vi "Engine.vi"(8 "Error In":errorcluster, 11 "Message Queues":T1) -> (0 "Error Out":errorcluster)   [LabVIEW 2014]
uses:
  Thread.ctl
  Teszt/Teszt.ctl
  Teszt/Command.ctl
  support/Message Queue/All Message Queues.ctl
  support/Message Queue/Message Cluster.ctl
  Message.ctl
  Thread Flag Control.ctl
  <vilib>/Utility/miscctls.llb/LVRectTypeDef.ctl
  support/Message Queue/Enqueue Message (Single).vi
  global/Global 1.vi
  <vilib>/Utility/error.llb/Error Cluster From Error Code.vi
  <vilib>/ErrorRing/Error Ring.xnode
  support/Message Queue/Message Queue.lvlib
panel:
  out "Threads":T2[](array[typedef])
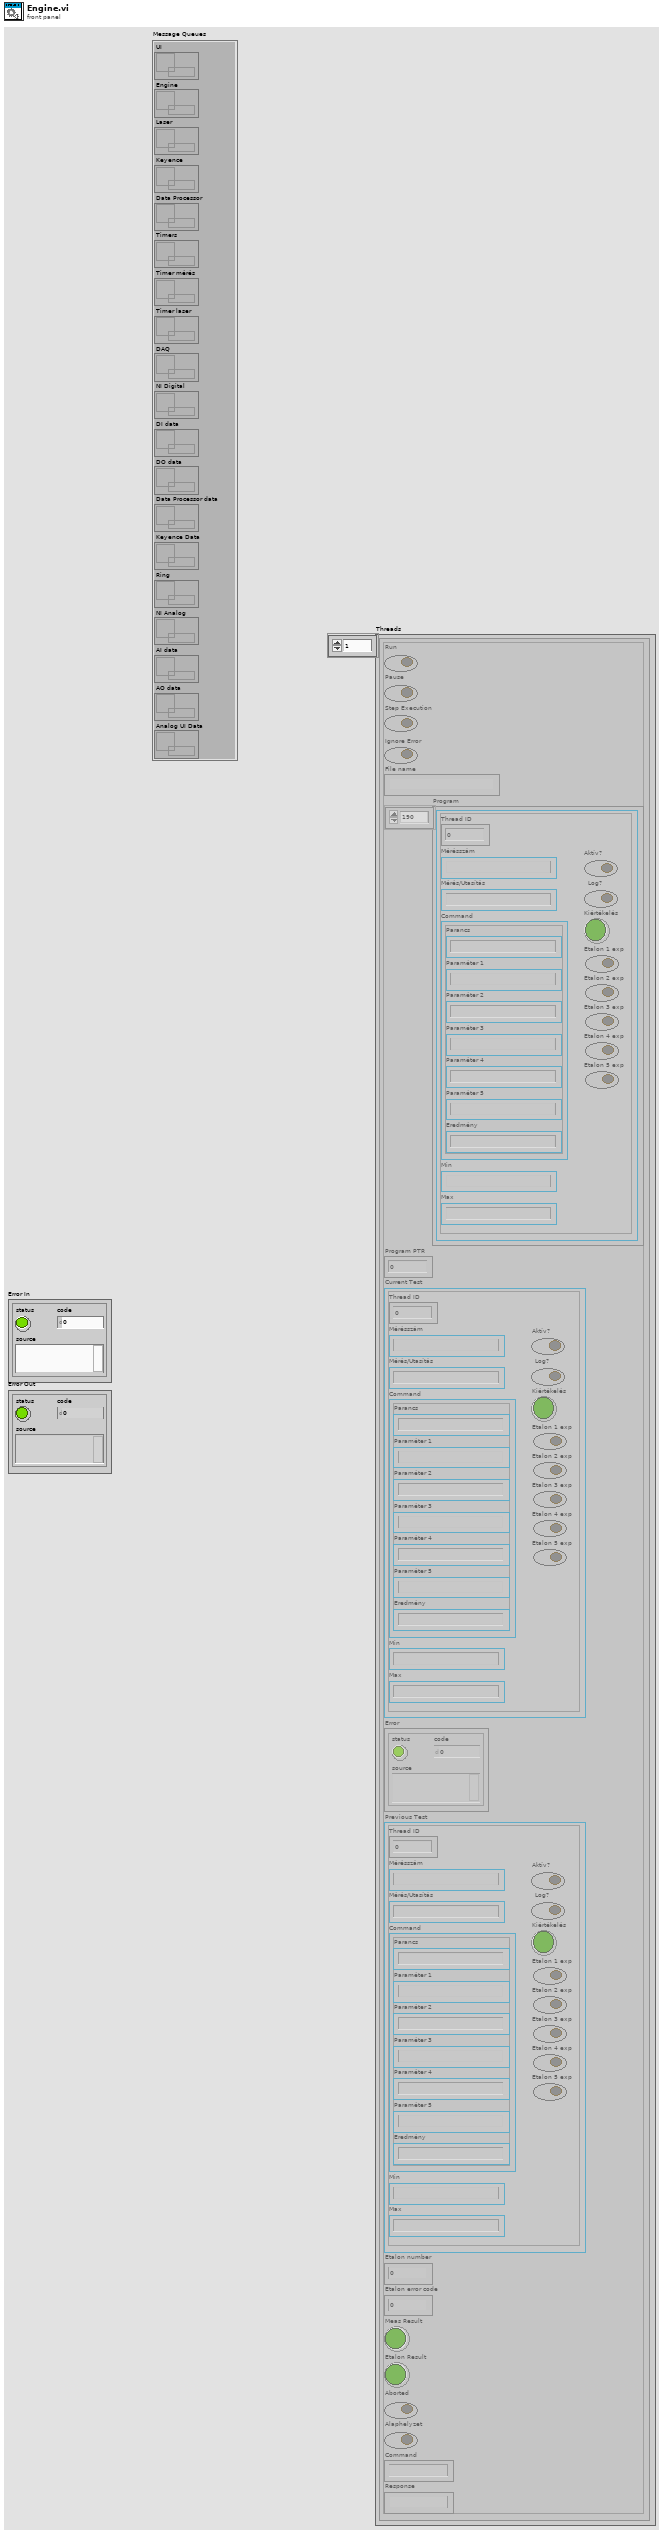
[diagram p1: front panel]
types:
  T1 = typedef "Message Queue.lvlib/All Message Queues.ctl" = cluster{"UI":refnum<queue>, "Engine":refnum<queue>, "Laser":refnum<queue>, "Keyence":refnum<queue>, "Data Processor":refnum<queue>, "Timers":refnum<queue>, "Timer mérés":refnum<queue>, "Timer laser":refnum<queue>, "DAQ":refnum<queue>, "NI Digital":refnum<queue>, "DI data":refnum<queue>, "DO data":refnum<queue>, "Data Processor data":refnum<queue>, "Keyence Data":refnum<queue>, "Ring":refnum<queue>, "NI Analog":refnum<queue>, "AI data":refnum<queue>, "AO data":refnum<queue>, "Analog UI Data":refnum<queue>}
  T2 = typedef "Thread.ctl" = cluster{"Run":bool, "Pause":bool, "Step Execution":bool, "Ignore Error":bool, "File name":string, "Program":T3[], "Program PTR":u32, "Current Test":T3, "Error":errorcluster, "Previous Test":T3, "Etalon number":u32, "Etalon error code":u32, "Meas Result":bool, "Etalon Result":bool, "Aborted":bool, "Alaphelyzet":bool, "Command":string, "Response":string}
  T3 = typedef "Teszt.ctl" = cluster{"Thread ID":dbl, "Mérésszám":string, "Mérés/Utasítás":string, "Command":T4, "Min":string, "Max":string, "Aktív?":bool, "Log?":bool, "Kiértékelés":bool, "Etalon 1 exp":bool, "Etalon 2 exp":bool, "Etalon 3 exp":bool, "Etalon 4 exp":bool, "Etalon 5 exp":bool}
  T4 = typedef "Command.ctl" = cluster{"Parancs":string, "Paraméter 1":string, "Paraméter 2":string, "Paraméter 3":string, "Paraméter 4":string, "Paraméter 5":string, "Eredmény":string}
  T5 = typedef "Termék cluster.ctl" = cluster{"Termék név":string, "Teszt szekvencia":path, "Etalonok száma":i8}
  T6 = typedef "LVRectTypeDef.ctl" = cluster{"Left":i16, "Top":i16, "Right":i16, "Bottom":i16}
  T7 = typedef "Message.ctl" = cluster{"Thread ID":u16, "Callback":string, "Data":variant, "Error":errorcluster}
  T8 = typedef "Thread Flag Control.ctl" = cluster{"Thread ID":u16, "Thread Flag":bool}
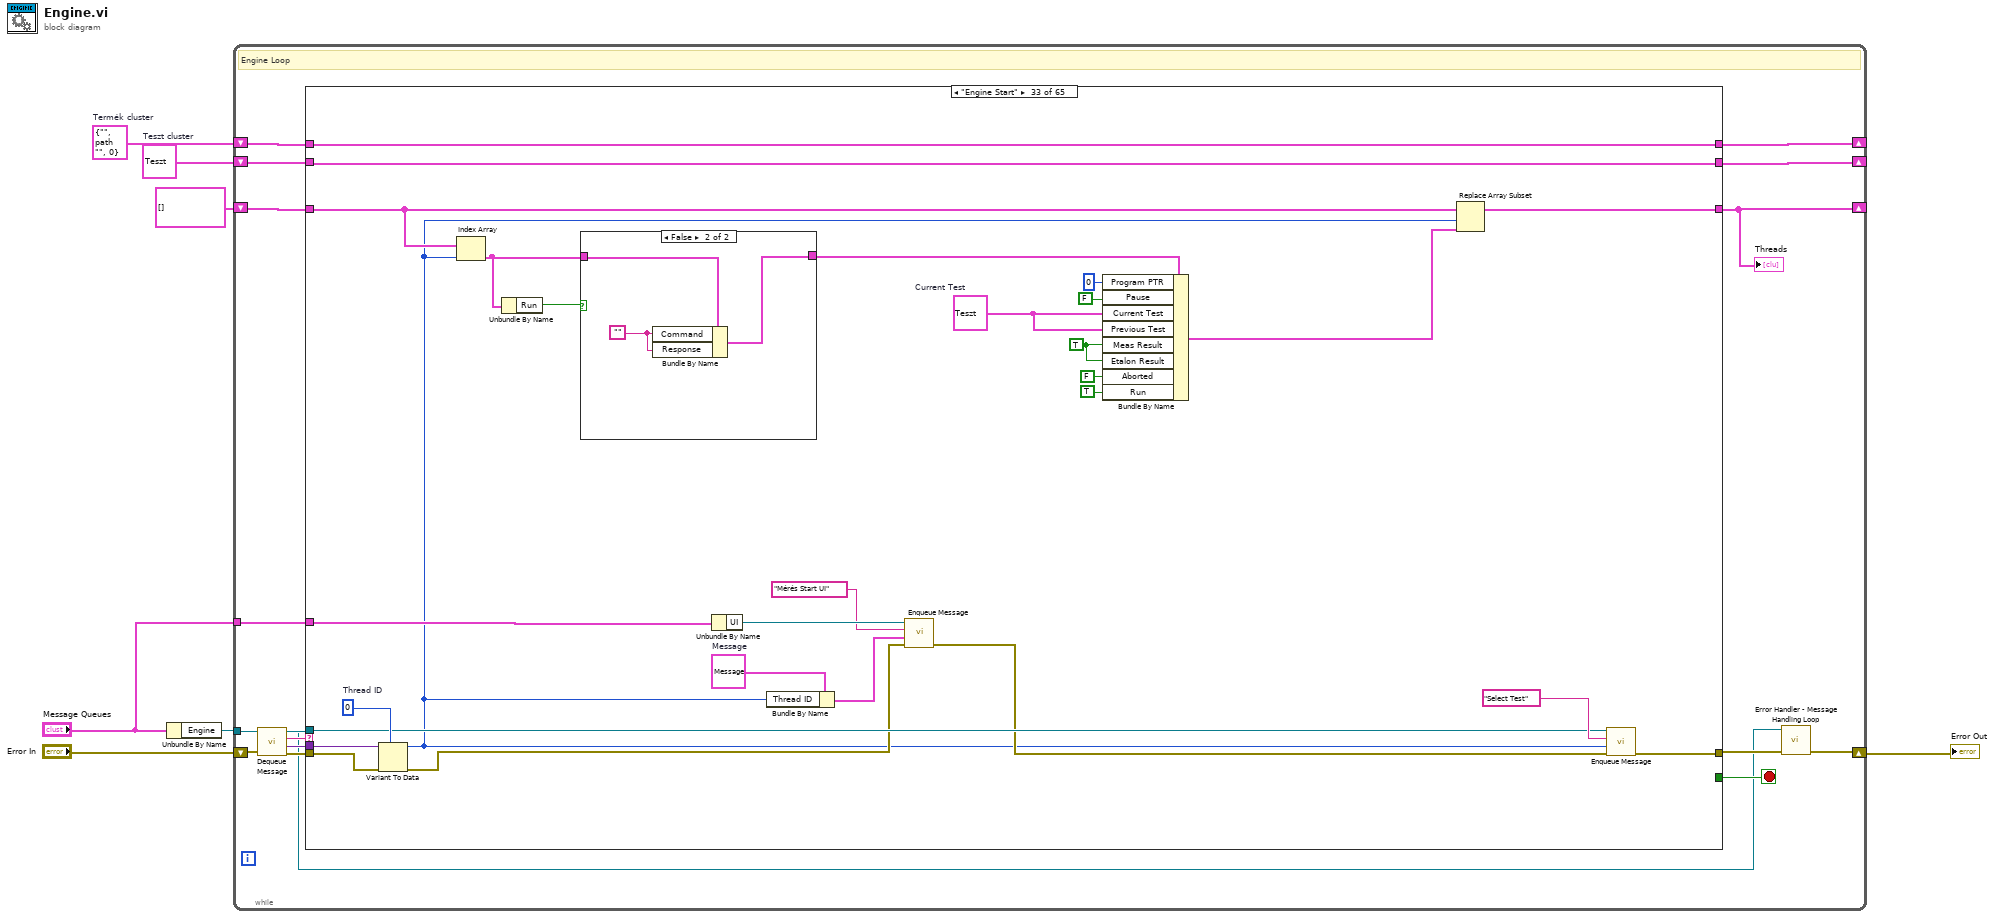
[diagram p0: block diagram]
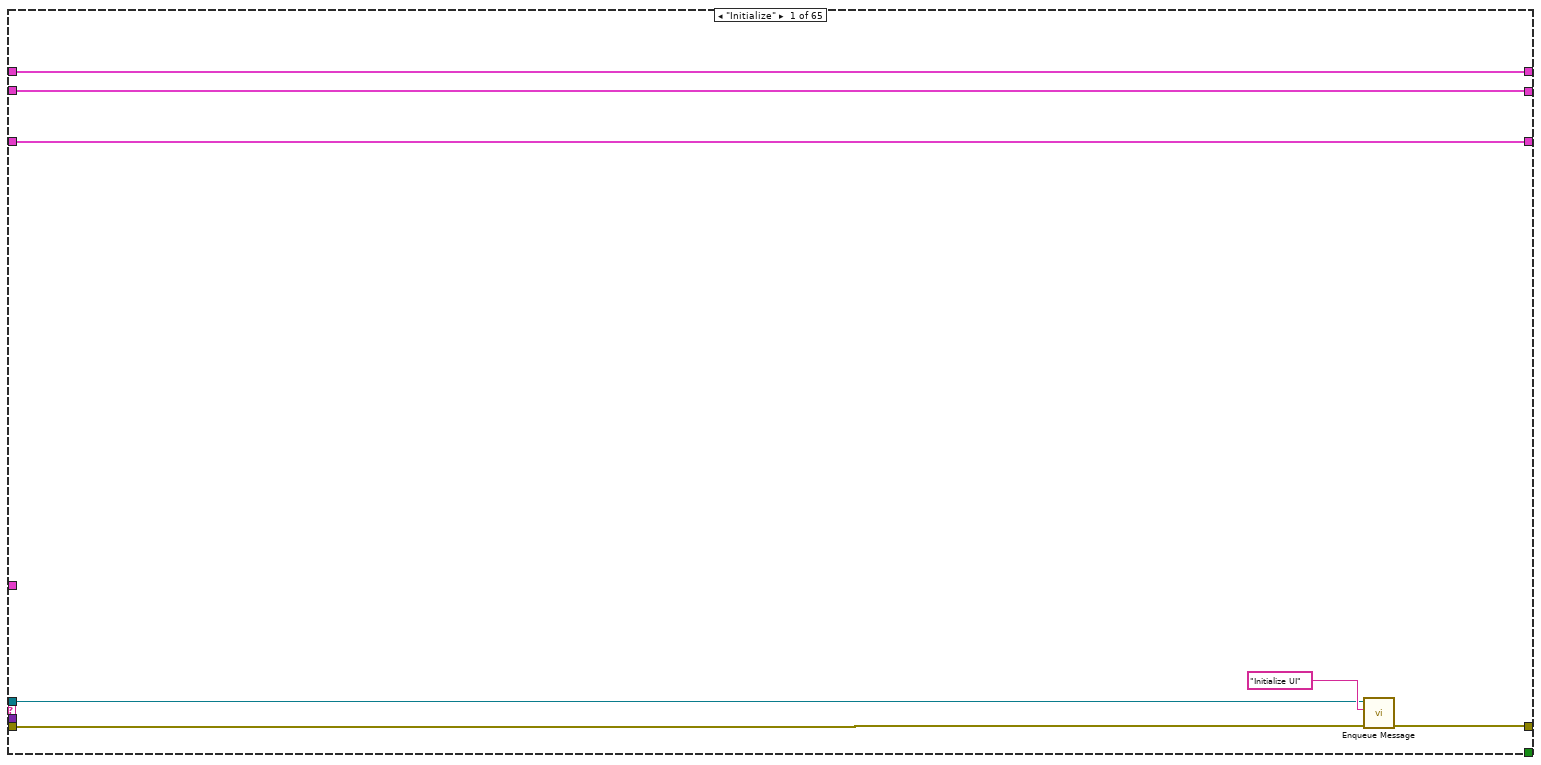
[diagram p2: hidden frame]
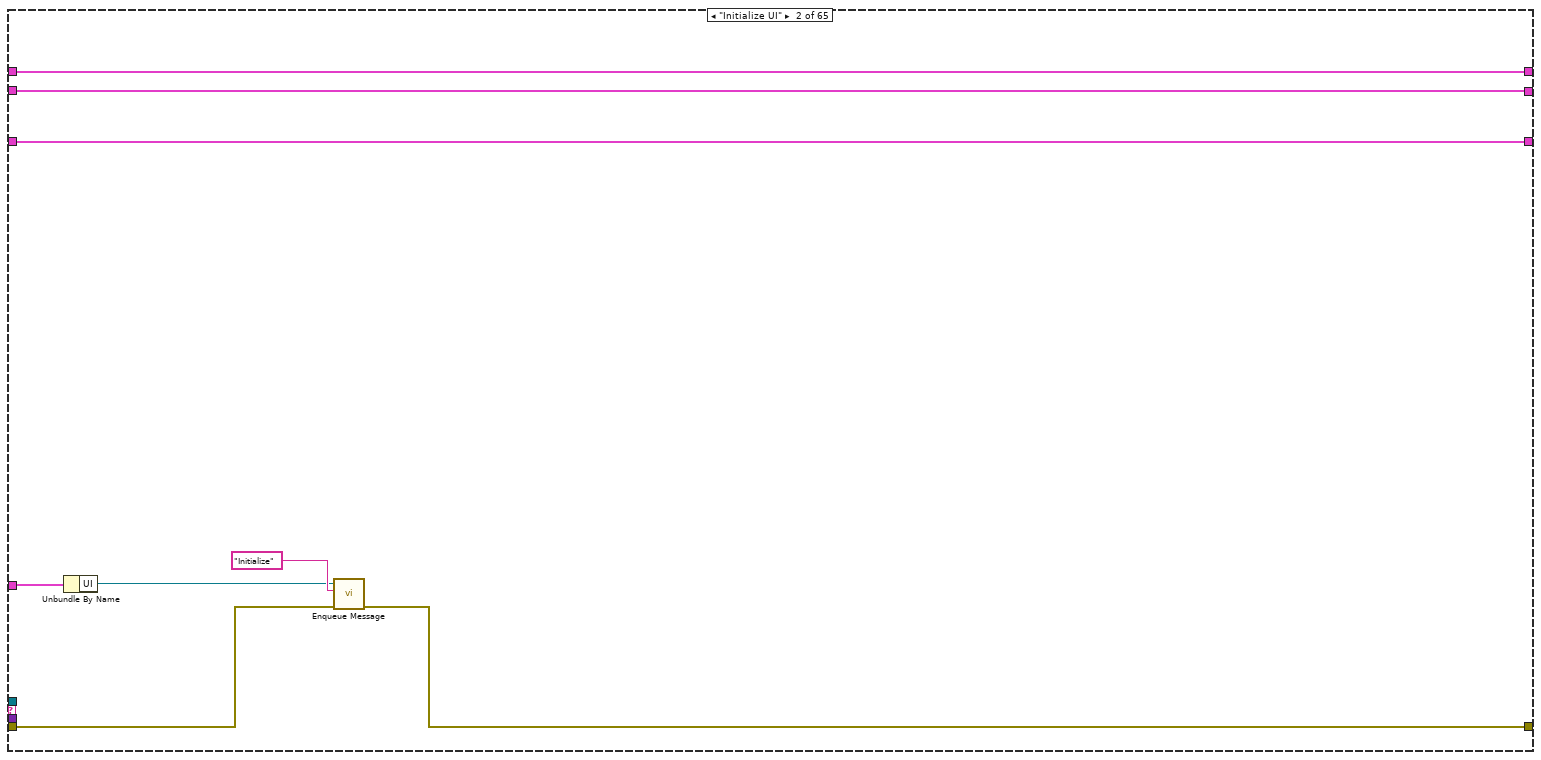
[diagram p3: hidden frame]
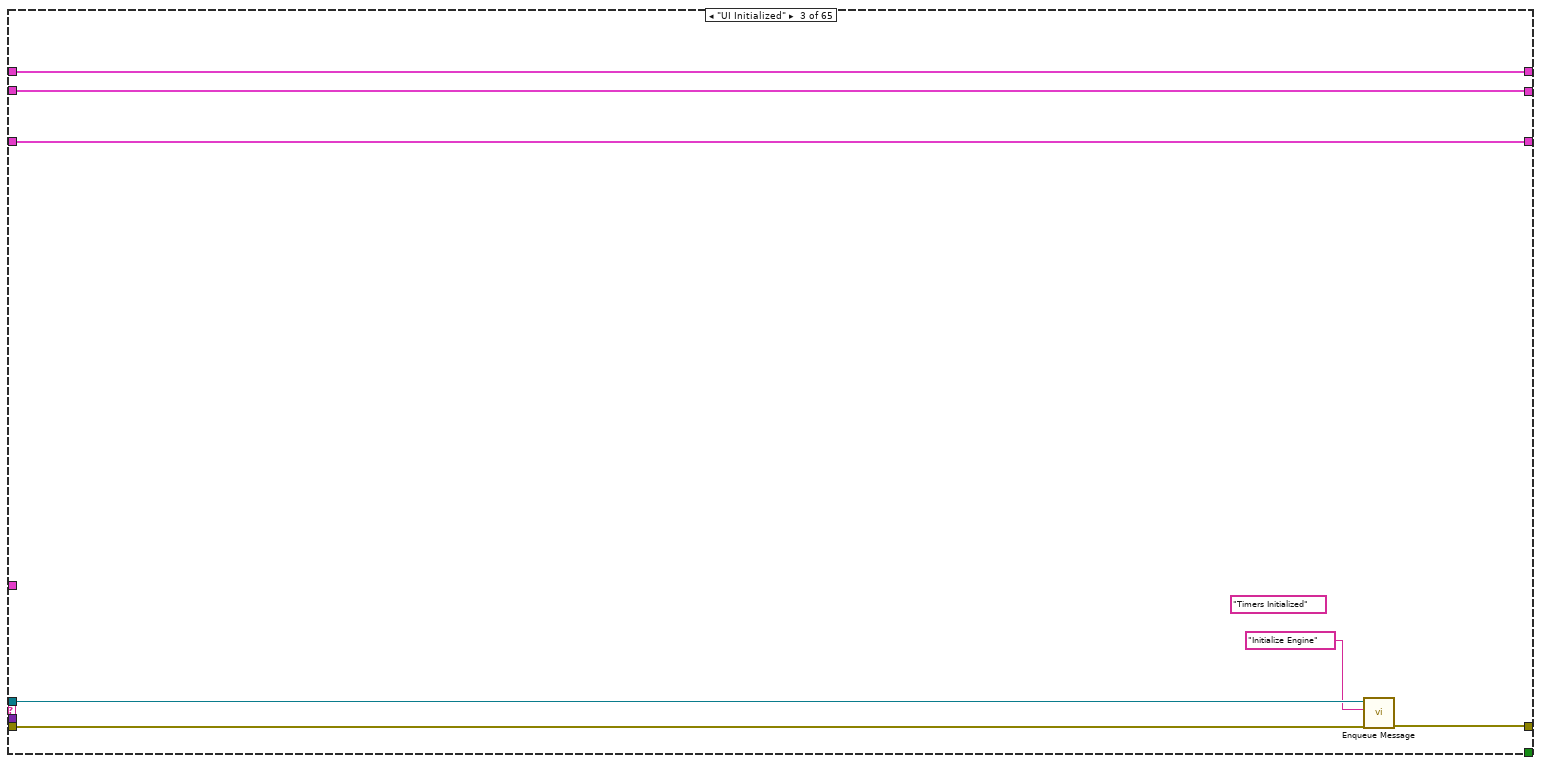
[diagram p4: hidden frame]
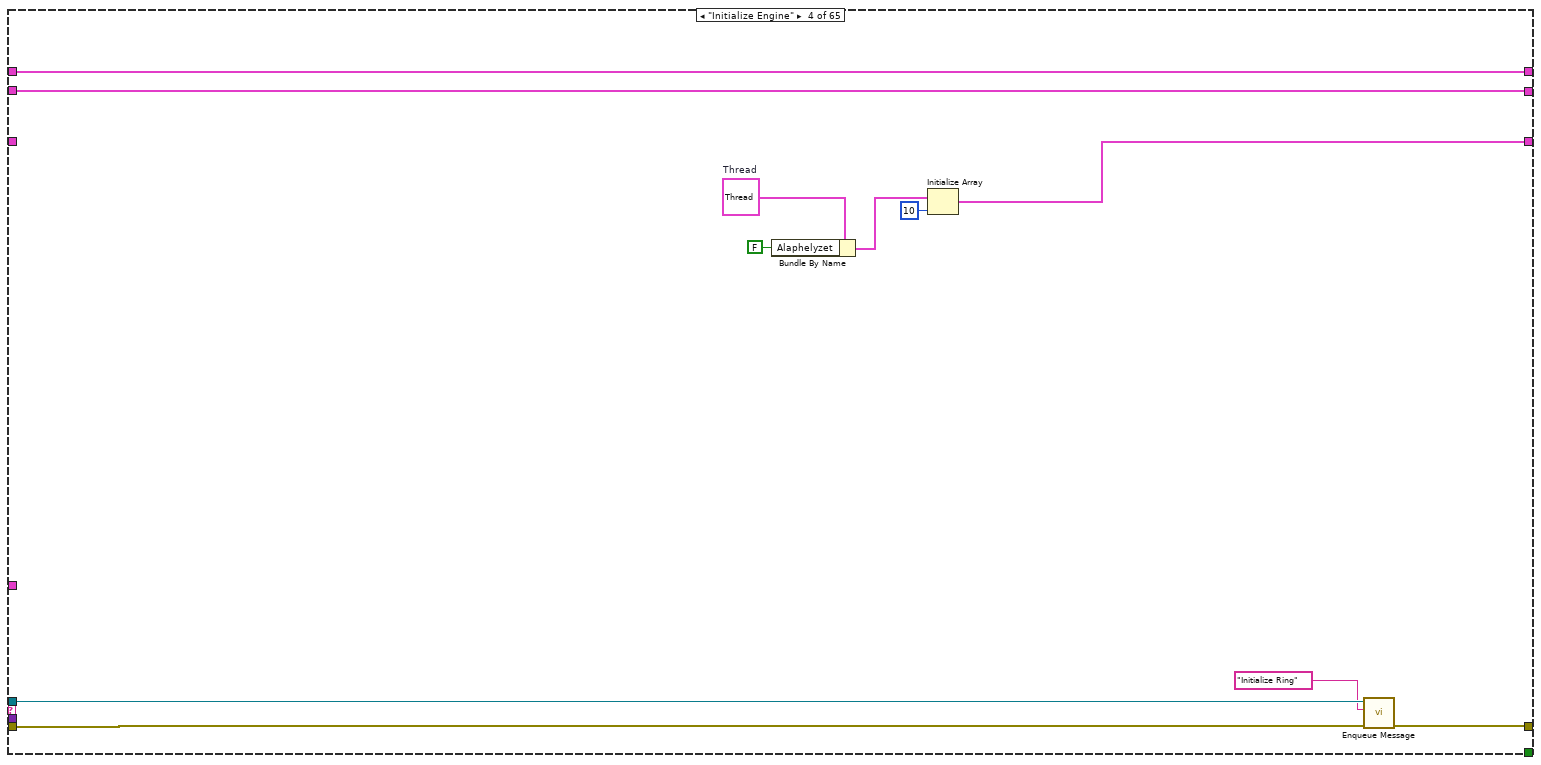
[diagram p5: hidden frame]
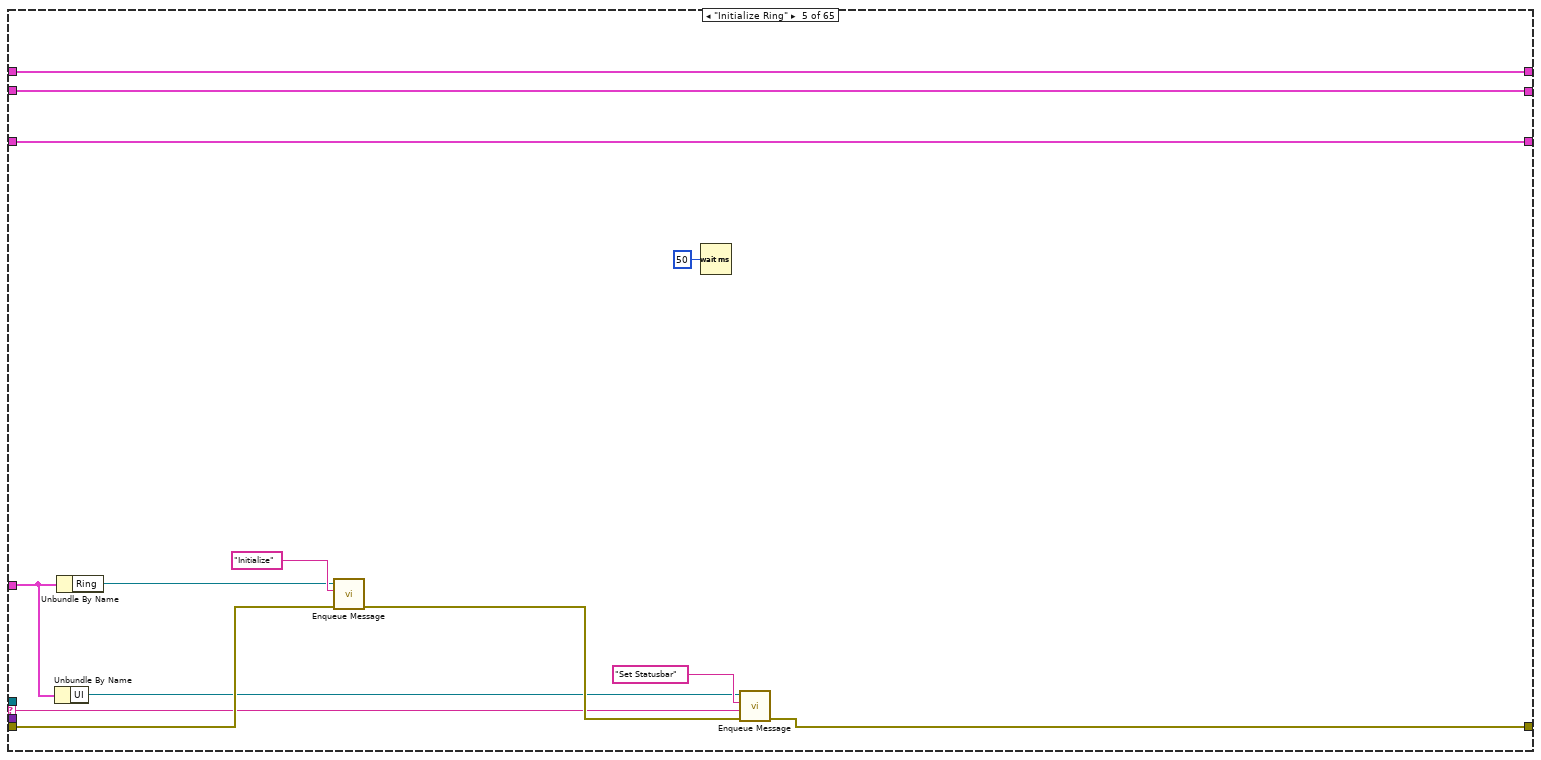
[diagram p6: hidden frame]
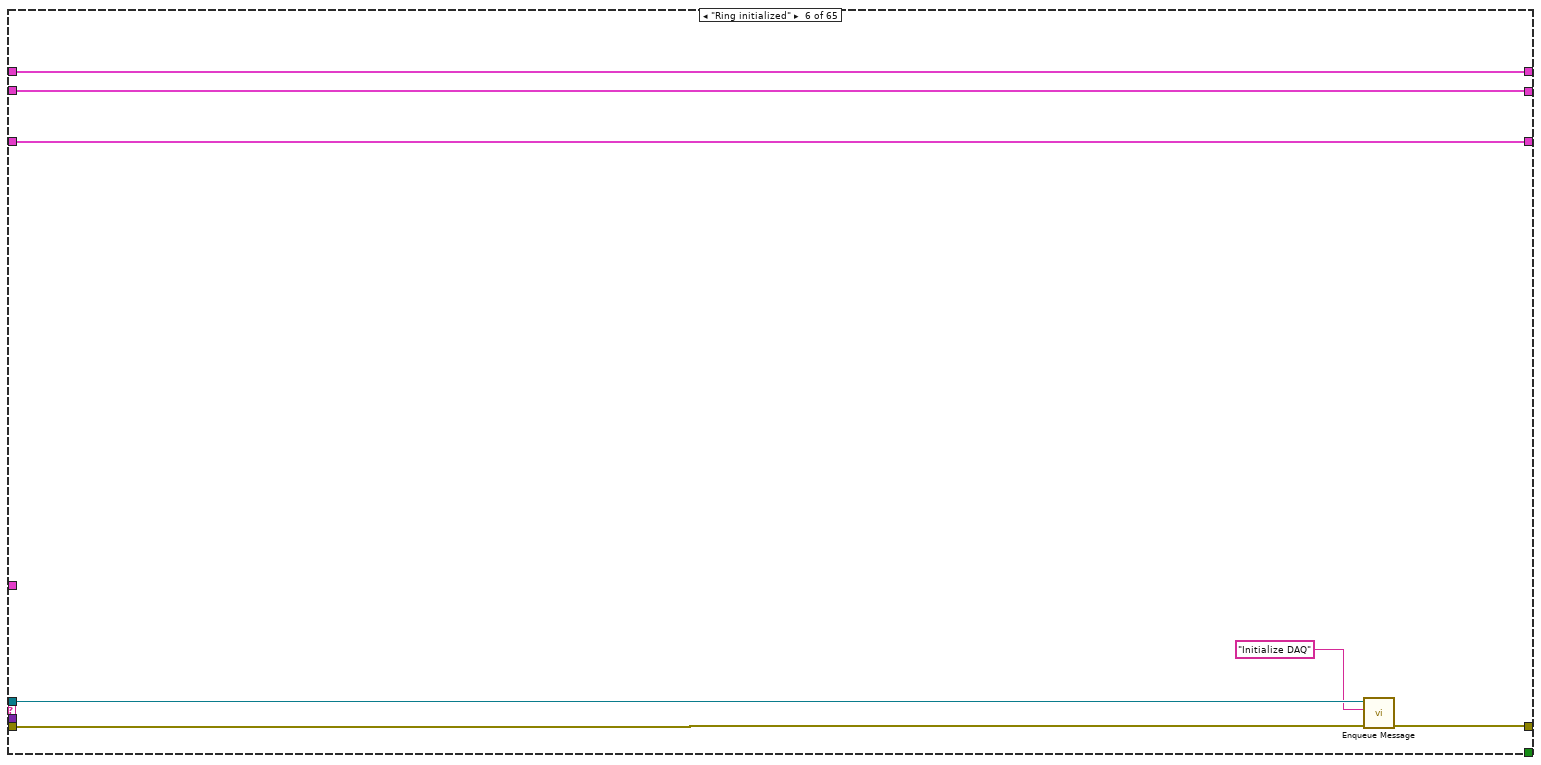
[diagram p7: hidden frame]
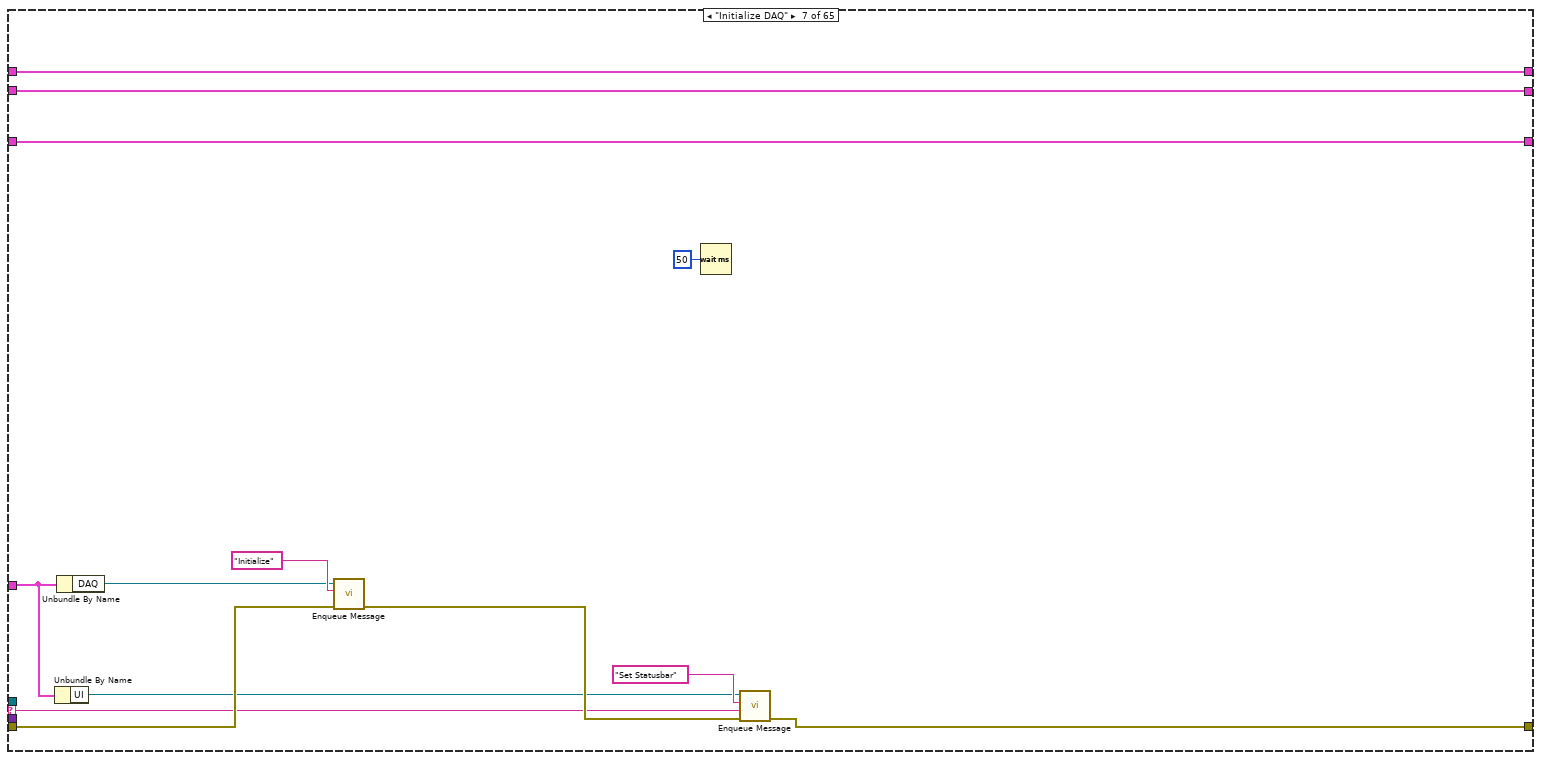
[diagram p8: hidden frame]
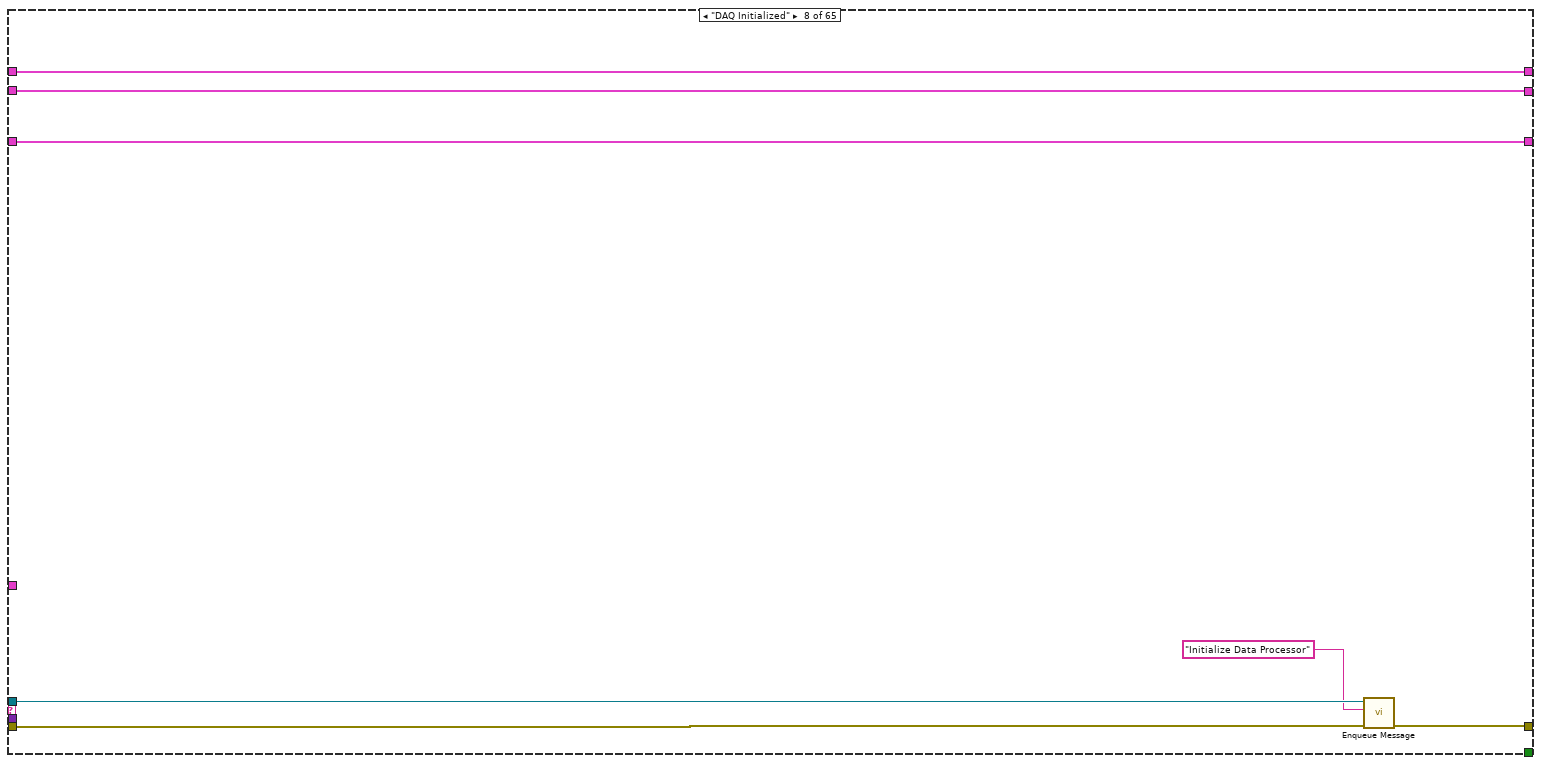
[diagram p9: hidden frame]
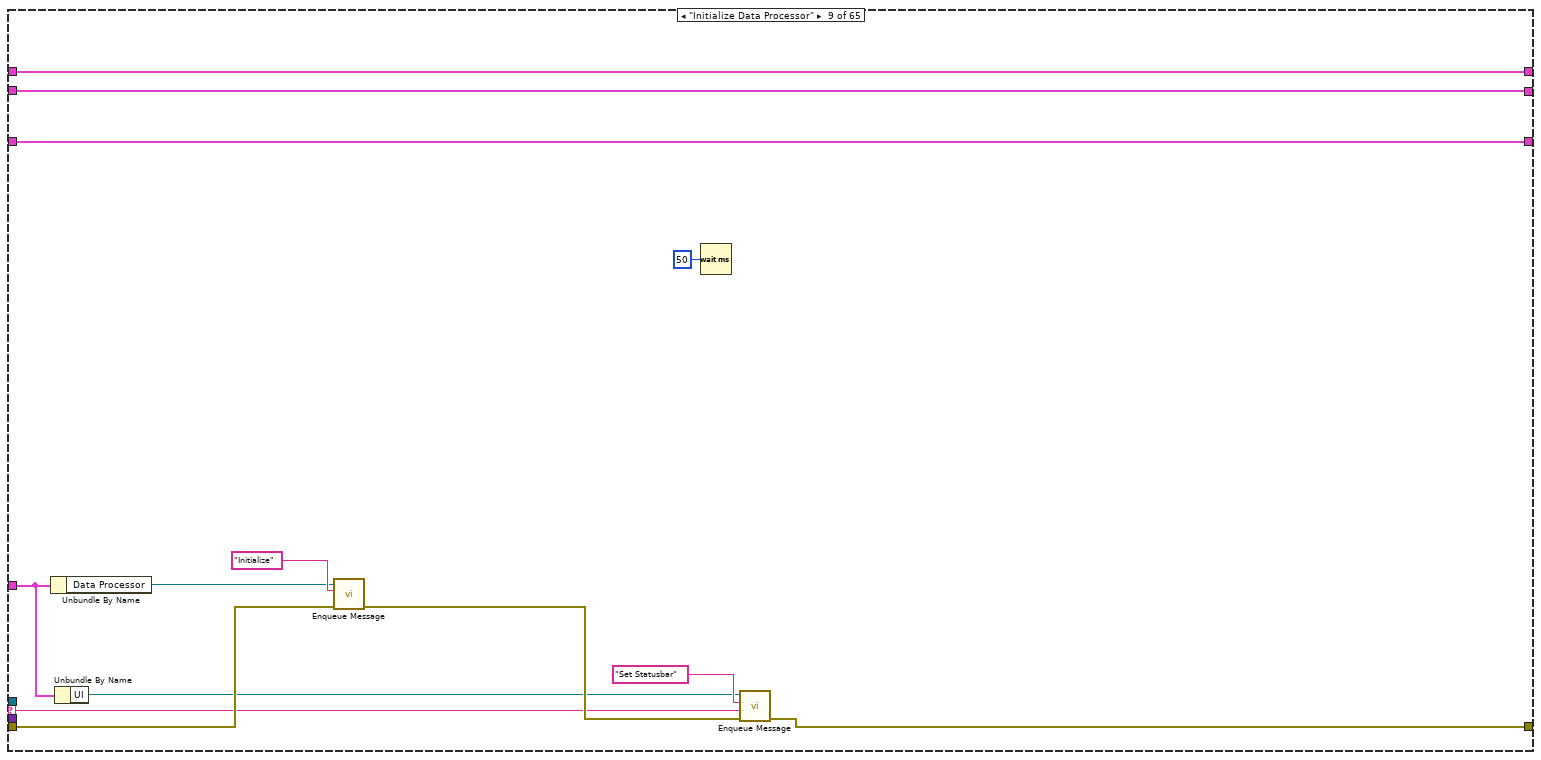
[diagram p10: hidden frame]
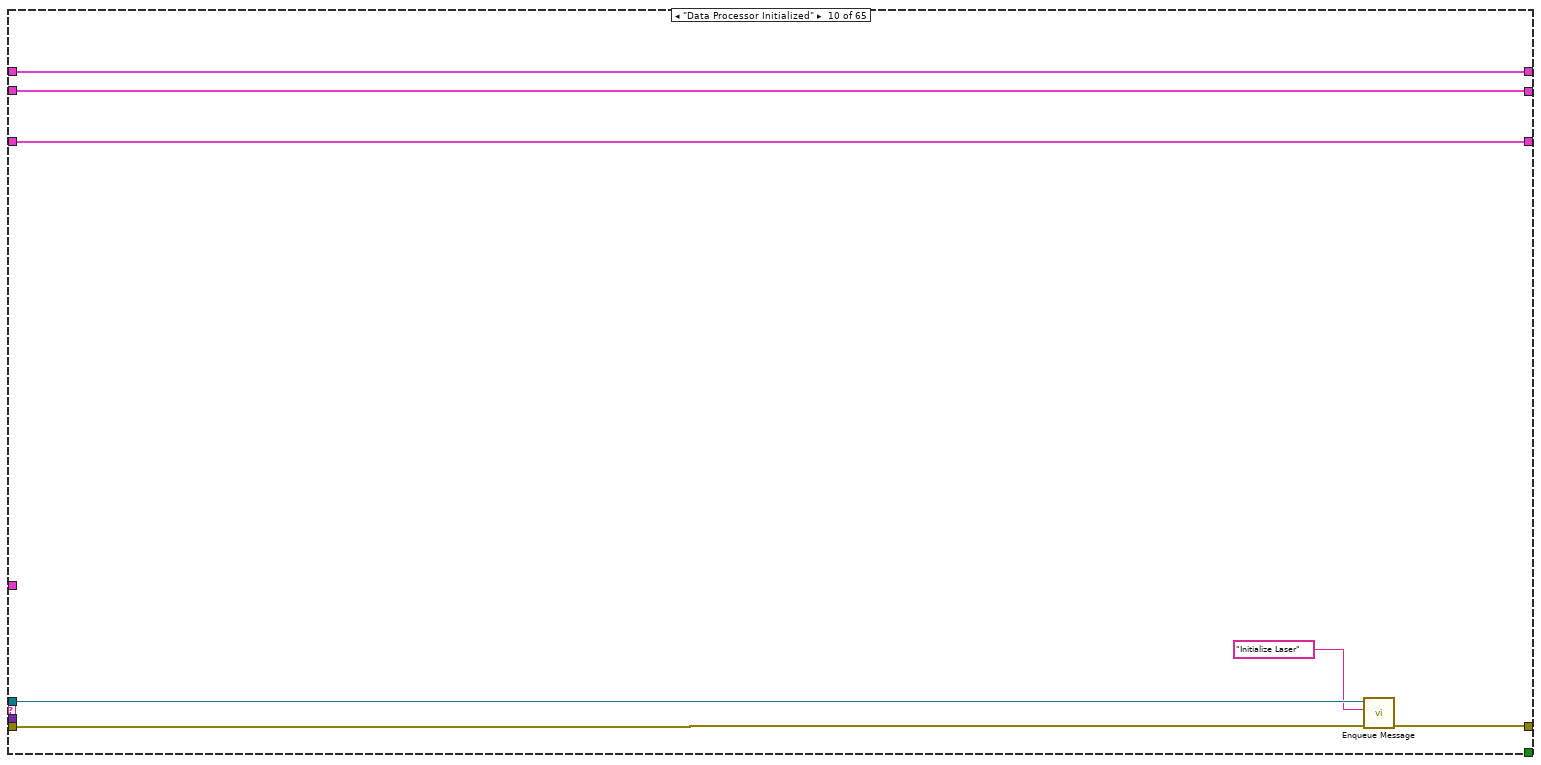
[diagram p11: hidden frame]
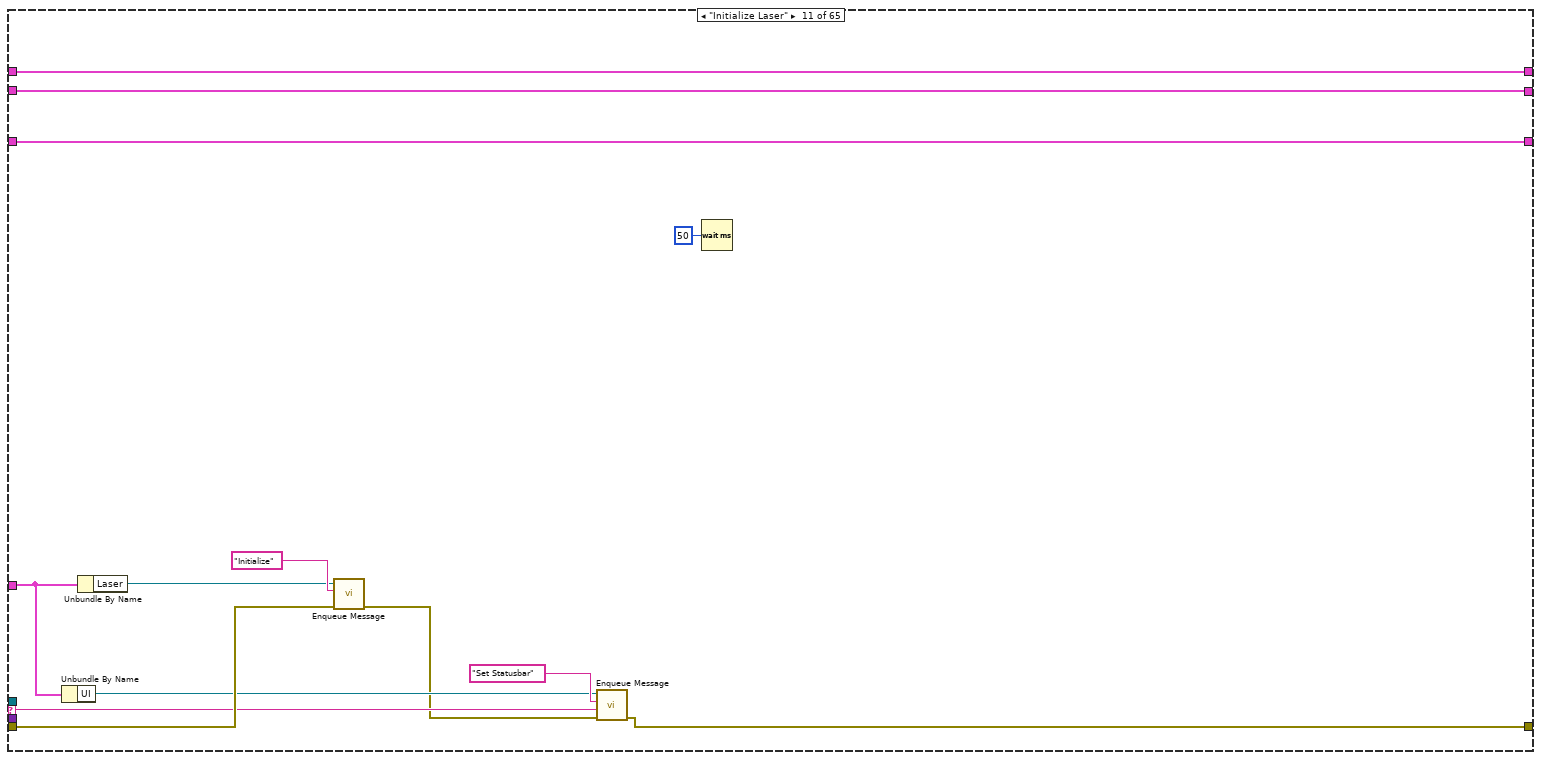
[diagram p12: hidden frame]
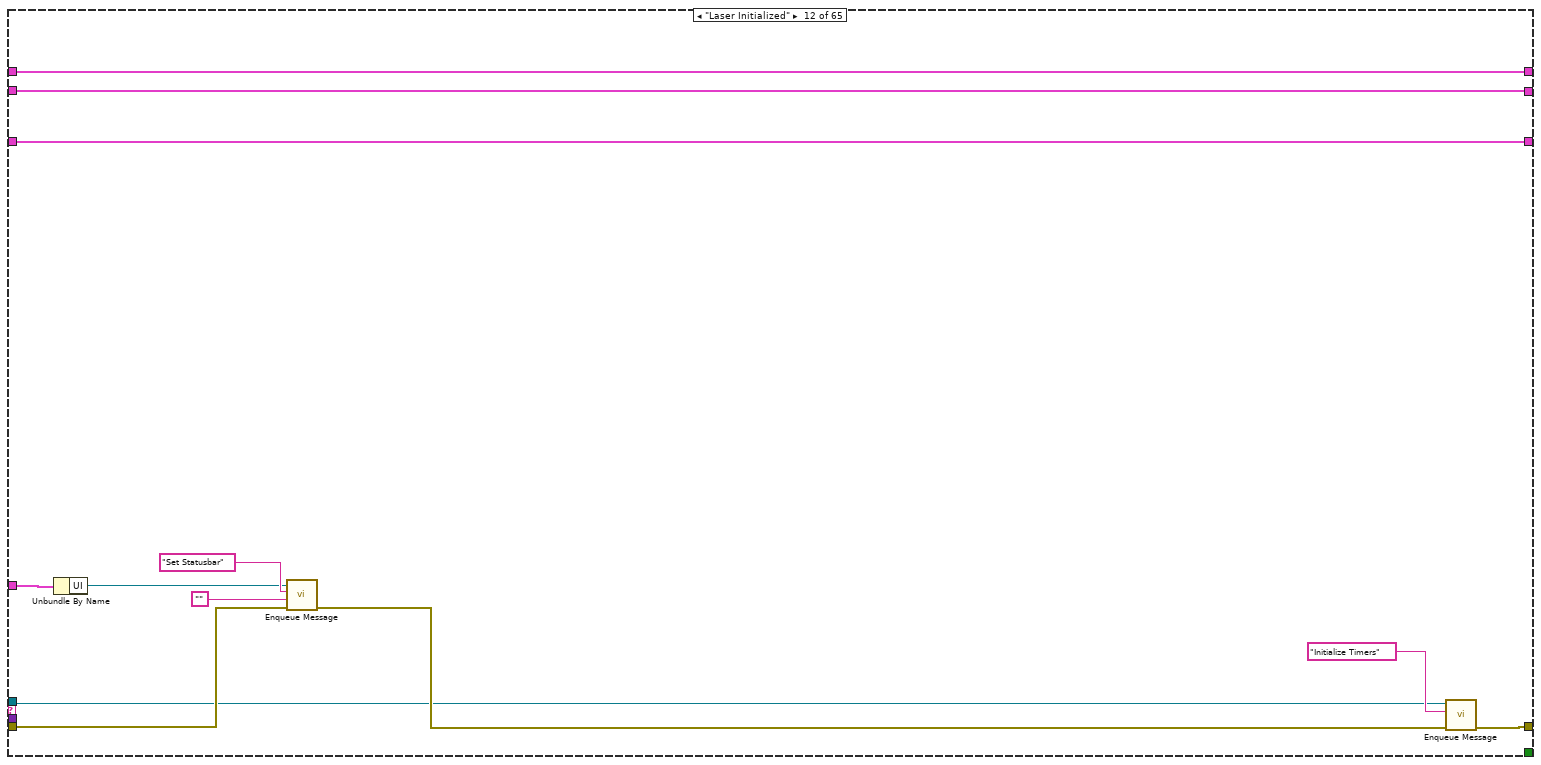
[diagram p13: hidden frame]
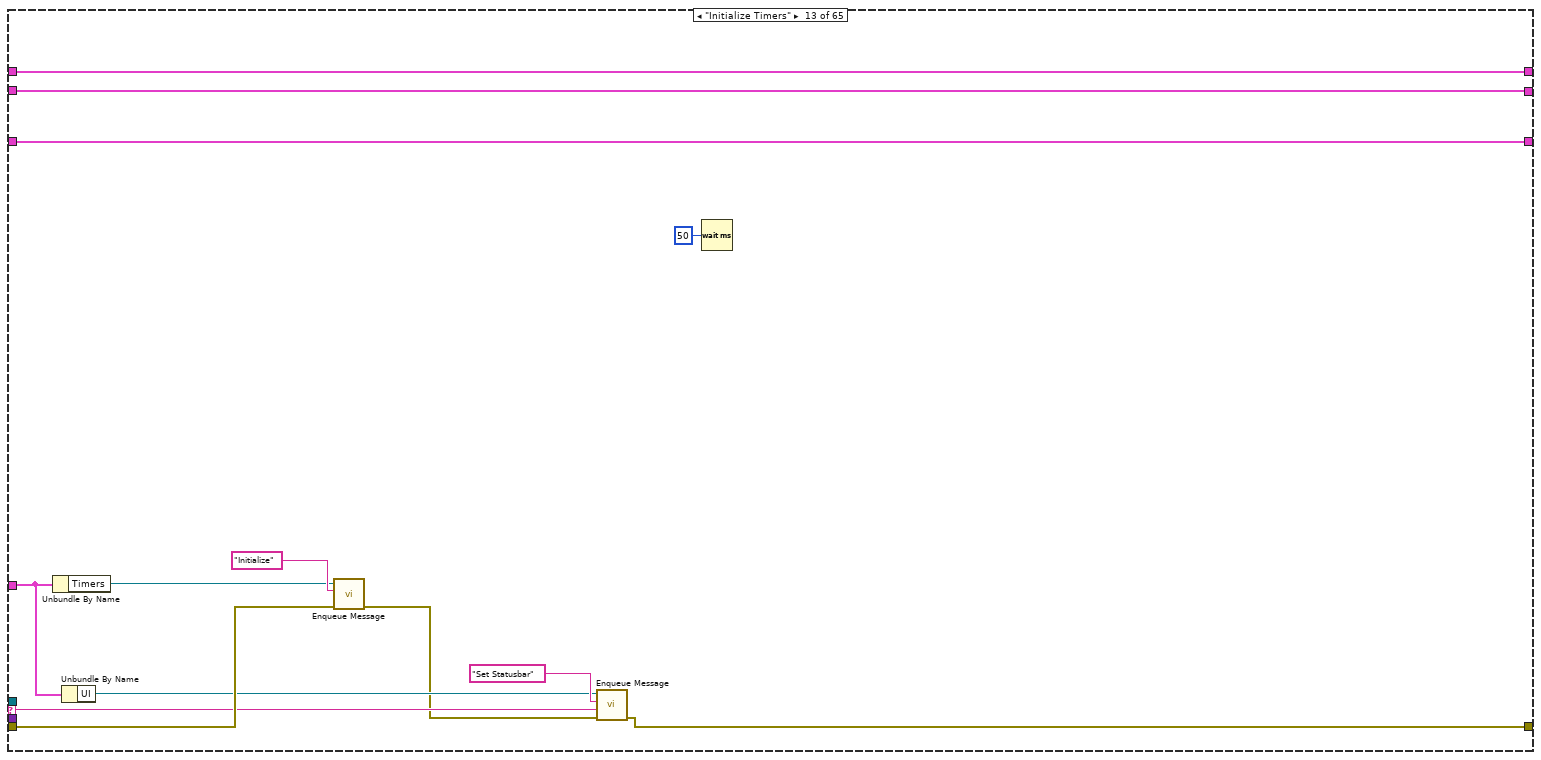
[diagram p14: hidden frame]
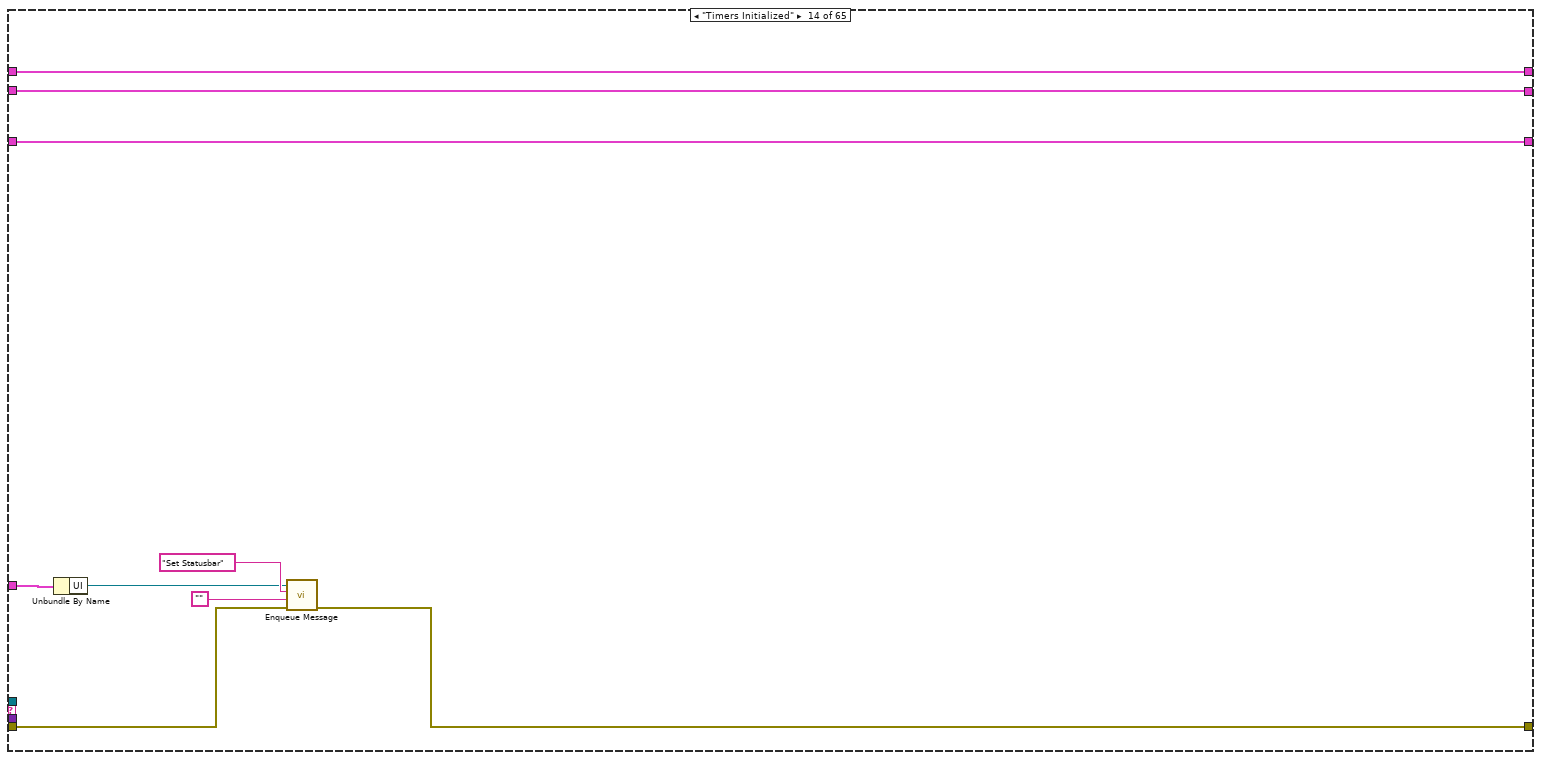
[diagram p15: hidden frame]
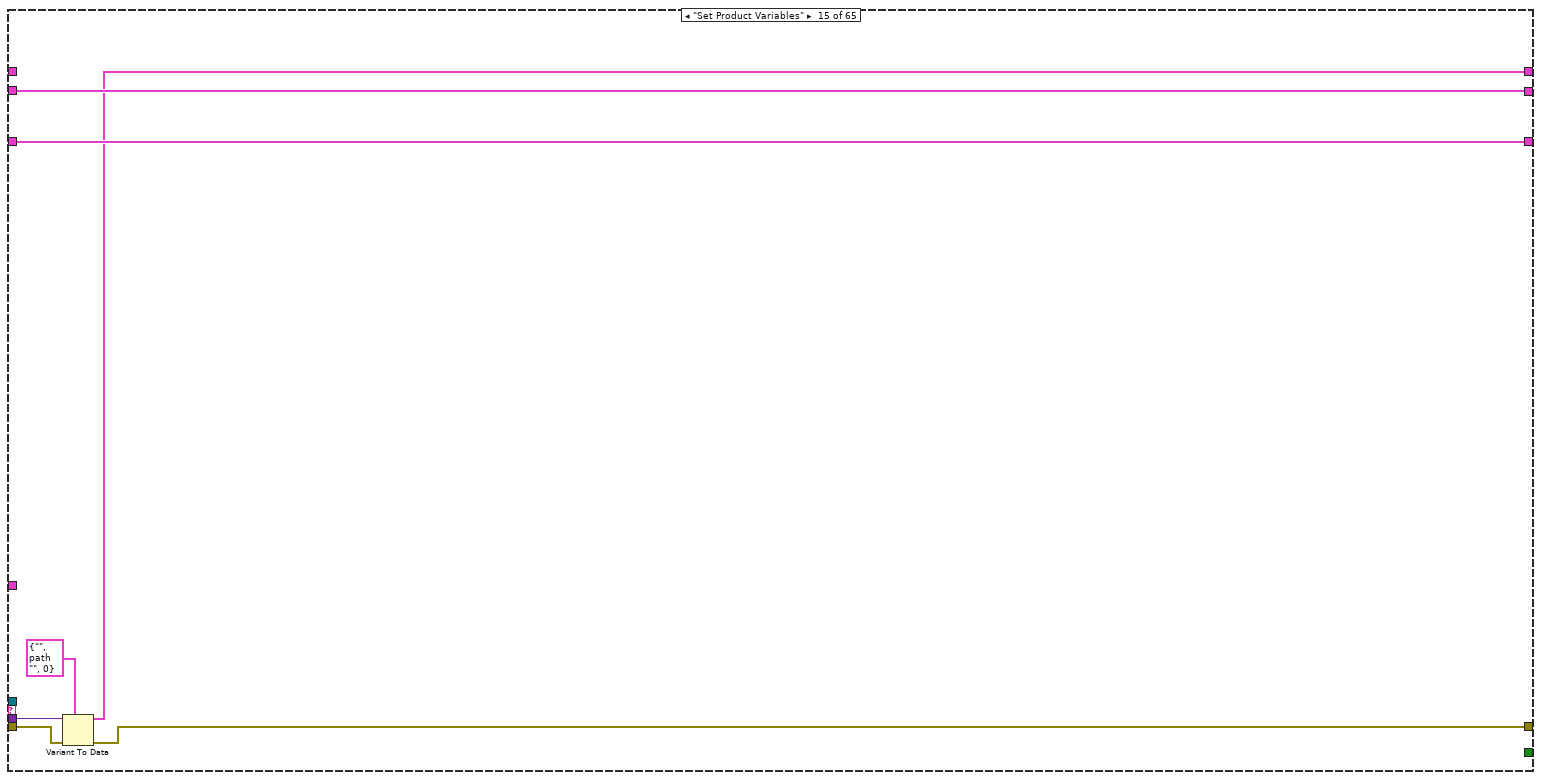
[diagram p16: hidden frame]
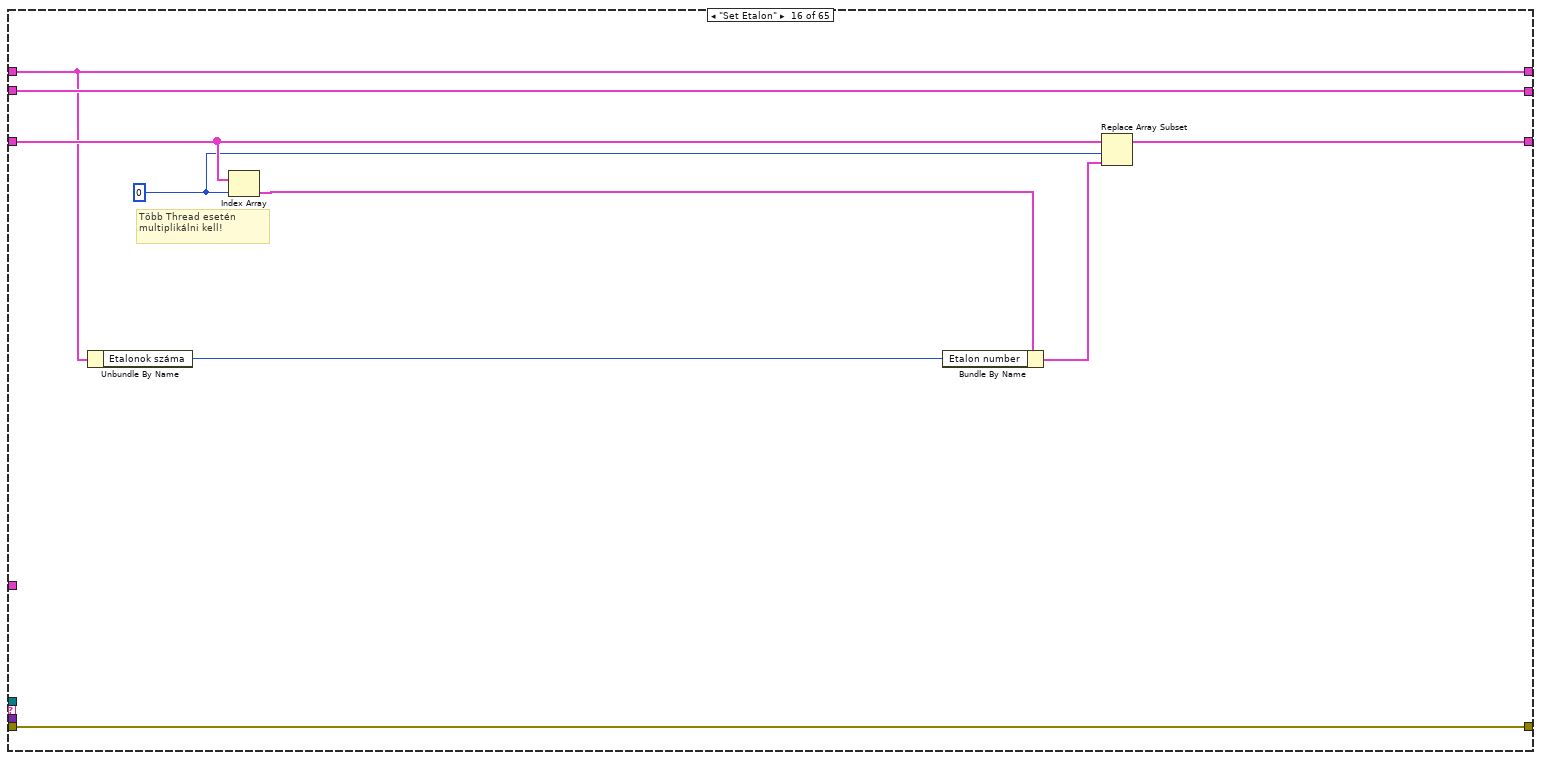
[diagram p17: hidden frame]
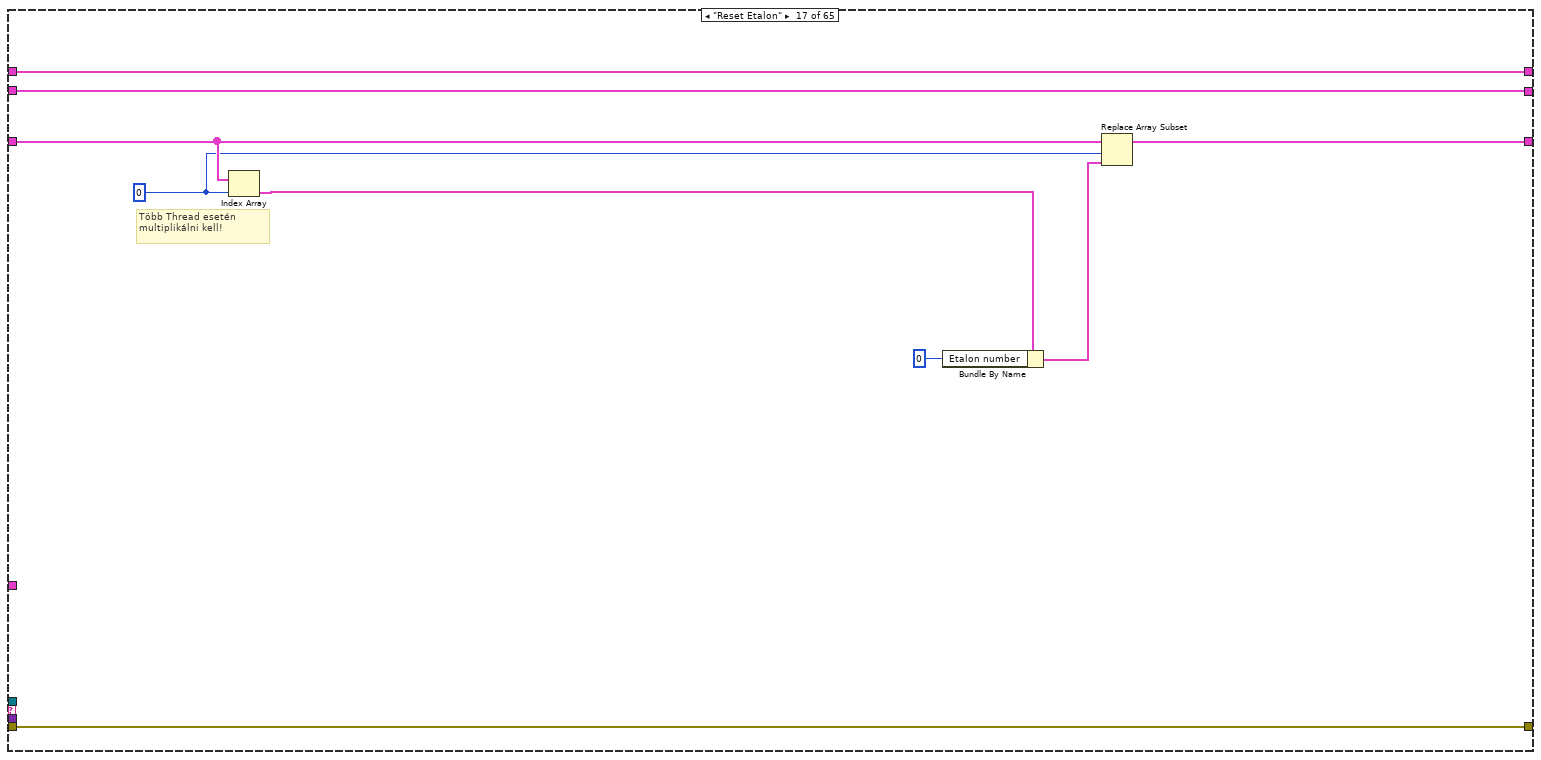
[diagram p18: hidden frame]
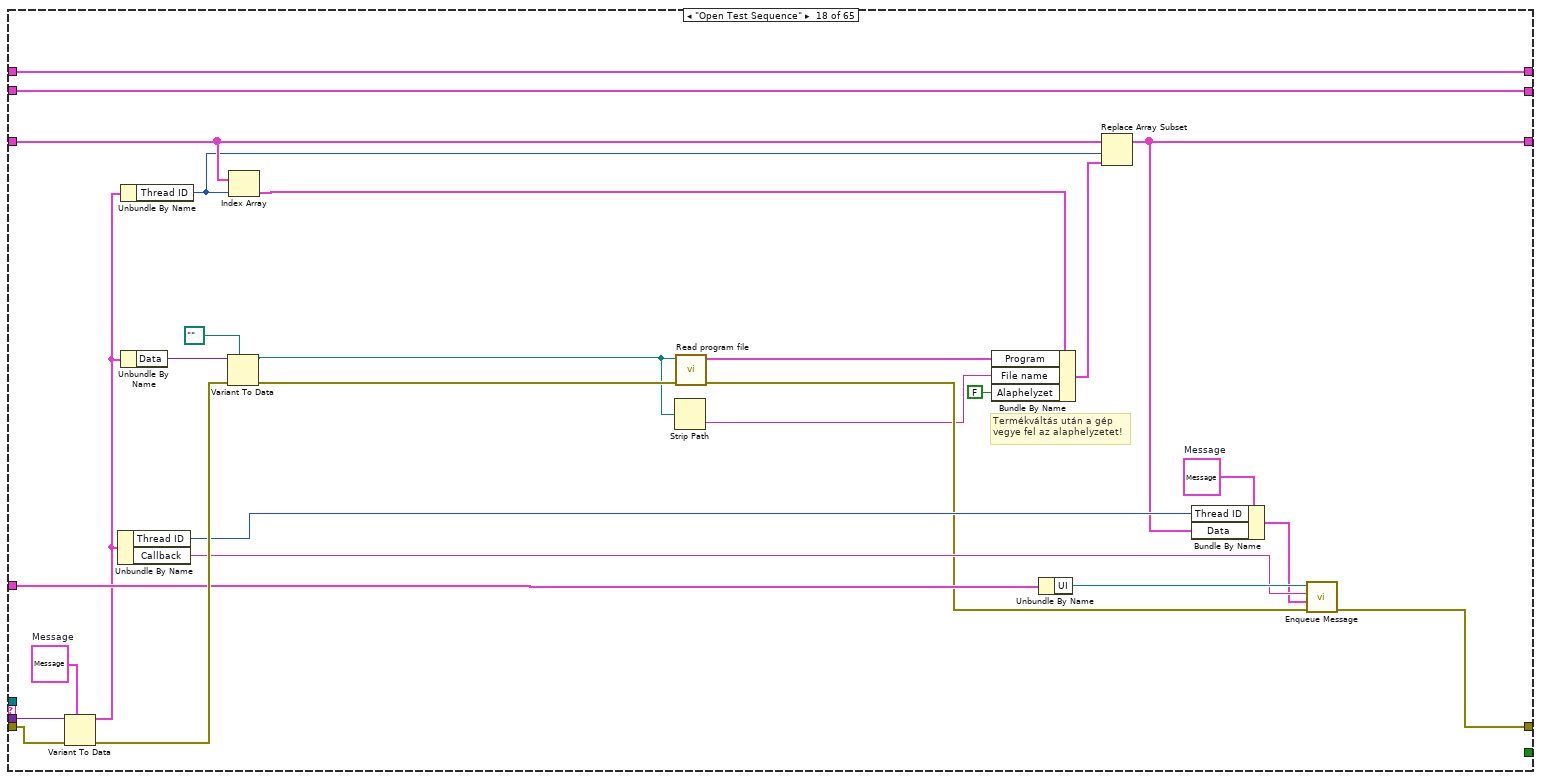
[diagram p19: hidden frame]
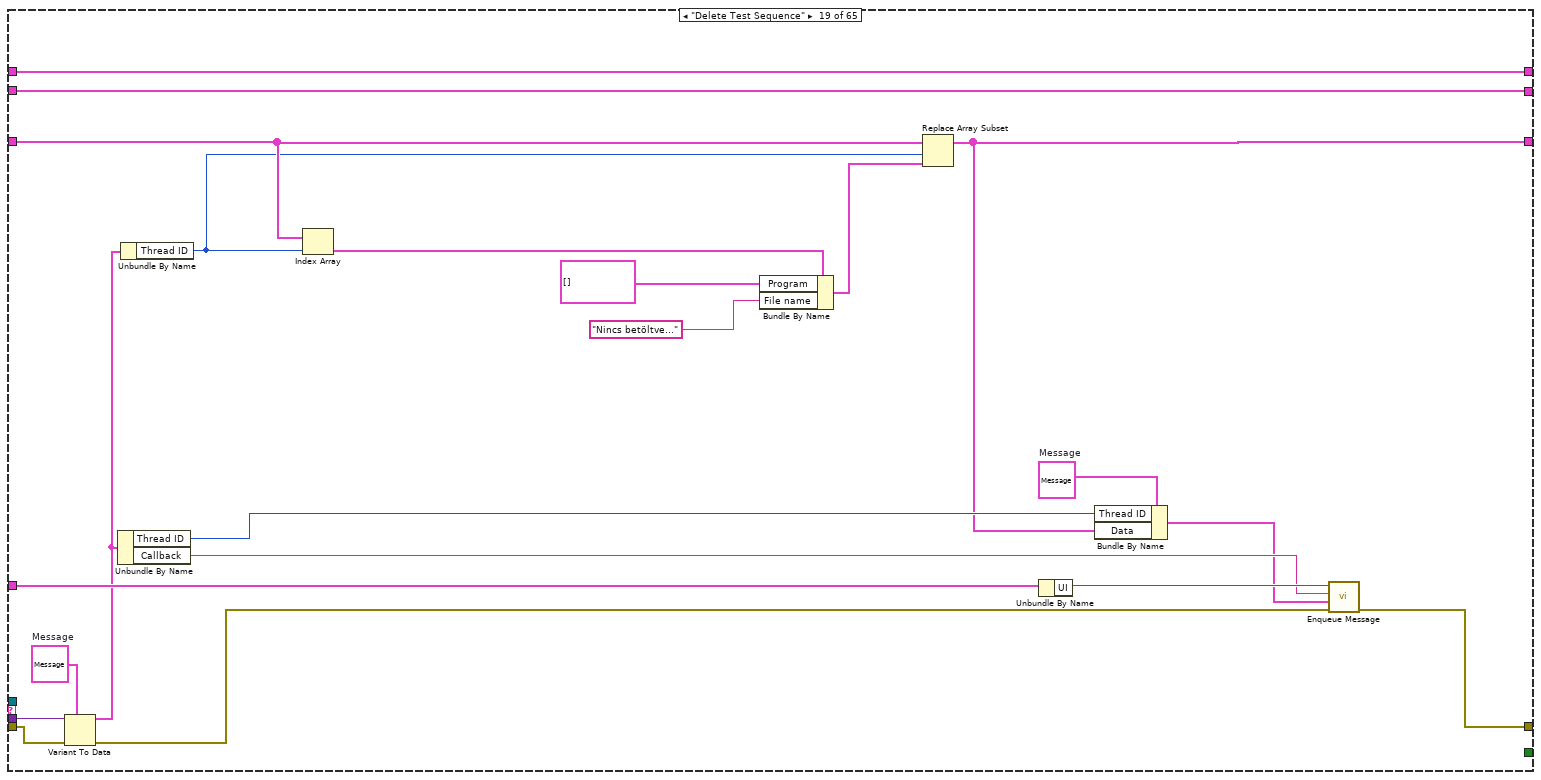
[diagram p20: hidden frame]
diagram:
  w2 = T5 {"Termék név"="", "Teszt szekvencia"=path "", "Etalonok száma"=0}  # Termék cluster
  w3 = T3 {"Thread ID"=0.0, "Mérésszám"="", "Mérés/Utasítás"="", "Command"={"Parancs"="", "Paraméter 1"="", "Paraméter 2"="", "Paraméter 3"="", "Paraméter 4"="", "Paraméter 5"="", "Eredmény"=""}, "Min"="", "Max"="", "Aktív?"=TRUE, "Log?"=TRUE, "Kiértékelés"=FALSE, "Etalon 1 exp"=TRUE, "Etalon 2 exp"=TRUE, "Etalon 3 exp"=TRUE, "Etalon 4 exp"=TRUE, "Etalon 5 exp"=TRUE}  # Teszt cluster
  n1 = Unbundle By Name("Message Queues") -> ("Engine"=w7:refnum<queue>)
  n2 = while {
    tunnel: "Message Queues" -> [w20]
    tunnel: w7 -> [w8]
    shift-right: [w16] -> _
    shift-left: T2[] [] -> [w18]
    shift-right: [w9] -> w5
    shift-left: "Error In" -> [w17]
    shift-right: [w14] -> _
    shift-left: w3 -> [w15]
    shift-right: [w13] -> _
    shift-left: w2 -> [w12]
    stop <- w19 stop-if-true
    # "Engine Loop"
    n3 = call "Dequeue Message.vi"("error in (no error)"=w17, "Message Queue"=w8) -> ("error out"=w23:errorcluster, "Message Data"=w22:variant, "Message"=w11:string, "dup Message Queue"=w21:refnum<queue>)  [unwired: 5 in, 1 out]
    n4 = case "Message Cases" shown="\"Engine Start\"" w11 {
      selector: w11 -> [_ _ _ _ w61 _ w81 _ w101 _ w121 _ w146 _ _ _ _ _ _ _ _ _ _ _ _ _ _ _ _ _ _ _ _ _ _ _ _ _ _ _ _ _ _ _ _ _ _ _ _ _ _ _ _ _ _ _ _ _ _ _ _ _ _ _ w1892]
      tunnel: w21 -> [w24 _ w42 w51 _ w72 _ w92 _ w112 _ w130 _ _ _ _ _ _ _ _ _ _ _ _ _ _ _ w405 w448 w486 _ _ w549 w582 w718 w766 w794 w878 w923 w951 w1038 w1061 w1095 w1136 w1205 w1255 w1287 w1318 w1381 w1402 w1431 w1454 w1538 w1583 w1639 w1665 w1694 w1730 w1769 w1801 w1826 w1862 w1877 w1887 _]
      tunnel: w23 -> [w25 w34 w40 w46 w66 w74 w86 w94 w106 w114 w126 w137 w151 w158 w167 w171 w181 w212 w232 w249 w275 w278 w299 w316 w339 w364 w390 w407 w452 w494 w516 w529 w557 w575 w726 w773 w790 w880 w934 w959 w1047 w1073 w1107 w1144 w1213 w1265 w1305 w1336 w1385 w1410 w1435 w1458 w1551 w1593 w1648 w1671 w1701 w1736 w1775 w1810 w1828 w1860 w1878 w1888 _]
      tunnel: [w28 w36 w43 w52 w60 w73 w80 w93 w100 w113 w118 w132 w143 w161 w166 w171 w181 w193 w222 w240 w259 w278 w289 w304 w330 w355 w381 w406 w467 w487 w507 w520 w551 w581 w704 w767 w793 w883 w924 w952 w1039 w1071 w1105 w1142 w1211 w1263 w1292 w1333 w1382 w1403 w1432 w1455 w1543 w1586 w1644 w1668 w1697 w1733 w1772 w1806 w1823 w1864 w1879 w1883 w1893] -> w10
      tunnel: w22 -> [_ _ _ _ _ _ _ _ _ _ _ _ _ _ w168 _ _ w213 w233 w250 w276 _ w300 w317 w340 w365 w391 w408 w451 w495 w517 w530 w558 w576 w727 w774 w791 w881 w935 w960 w1048 w1074 w1108 w1145 w1214 w1266 w1306 w1337 w1386 w1411 w1436 w1459 w1552 w1594 w1649 w1672 w1702 w1737 w1776 w1811 w1829 w1868 _ _ _]
      tunnel: w20 -> [_ w32 _ _ w59 _ w79 _ w99 _ w120 w136 w145 w157 _ _ _ w207 w229 w247 w261 _ w296 _ w336 w361 w387 w404 _ w485 _ _ w546 w567 w716 _ w795 w884 _ _ _ _ _ _ _ _ _ w1326 w1373 _ _ _ _ _ _ _ w1691 w1727 w1766 _ _ w1870 _ _ _]
      tunnel: [_ _ _ _ _ _ _ _ _ _ _ _ _ _ _ _ _ _ _ _ _ _ _ _ _ _ _ _ _ _ _ _ _ _ _ _ _ _ _ _ _ _ _ _ _ _ _ _ _ _ _ _ _ _ _ _ _ _ _ _ _ _ _ TRUE _] -> w19
      tunnel: w18 -> [w26 w33 w41 _ w65 w71 w85 w91 w105 w111 w125 w138 w150 w159 w170 w178 w187 w214 w234 w238 w255 w281 w301 w306 w341 w366 w392 w394 w456 w490 w512 w525 w553 w570 w710 w770 w783 w876 w928 w956 w1046 w1057 w1091 w1131 w1196 w1256 w1301 w1328 w1375 w1409 w1424 w1451 w1549 w1591 w1647 w1660 w1700 w1722 w1761 w1809 w1818 w1872 w1881 w1885 w1891]
      tunnel: [w26 w33 w41 w55 w65 w71 w85 w91 w105 w111 w125 w138 w150 w159 w170 w177 w186 w200 w221 w238 w252 w281 w288 w306 w329 w354 w380 w394 w454 w489 w511 w524 w552 w571 w721 w769 w788 w877 w927 w955 w1045 w1057 w1091 w1134 w1196 w1256 w1302 w1328 w1375 w1408 w1424 w1451 w1549 w1591 w1647 w1660 w1700 w1722 w1761 w1809 w1818 w1872 w1881 w1885 w1891] -> w16
      tunnel: w15 -> [w30 w38 w45 w54 w69 w76 w89 w96 w109 w116 w129 w141 w154 w163 w169 w175 w184 w195 w220 w239 w268 w280 w285 _ w321 w345 w373 w397 w466 w479 w506 w519 w540 w564 w714 w760 w784 w874 w940 w965 w1053 w1079 w1113 w1139 w1208 w1261 w1303 w1342 w1391 w1416 w1441 w1464 w1557 w1599 w1654 w1677 w1707 w1742 w1781 w1816 w1819 w1873 w1880 w1884 w1890]
      tunnel: [w30 w38 w45 w54 w69 w76 w89 w96 w109 w116 w129 w141 w154 w163 w169 w175 w184 w195 w220 w239 w268 w279 w285 w305 w321 w345 w373 w397 w466 w479 w506 w519 w540 w564 w714 w760 w784 w874 w940 w965 w1053 w1079 w1113 w1139 w1208 w1261 w1303 w1342 w1391 w1416 w1441 w1464 w1557 w1599 w1654 w1677 w1707 w1742 w1781 w1816 w1819 w1873 w1880 w1884 w1890] -> w14
      tunnel: [w29 w37 w44 w53 w68 w75 w88 w95 w108 w115 w128 w140 w153 w162 w165 w173 w182 w194 w217 w237 w251 w277 w282 w303 w318 w343 w368 w396 w465 w478 w505 w518 w538 w563 w712 w759 w779 w873 w918 w948 w1043 w1072 w1106 w1143 w1212 w1264 w1304 w1335 w1384 w1406 w1434 w1457 w1533 w1574 w1640 w1656 w1695 w1731 w1770 w1802 w1820 w1871 w1875 w1882 w1889] -> w13
      tunnel: w12 -> [w29 w37 w44 w53 w68 w75 w88 w95 w108 w115 w128 w140 w153 w162 _ w173 w182 w194 w217 w237 w251 w277 w282 w303 w318 w343 w368 w396 w465 w478 w505 w518 w538 w563 w712 w759 w779 w873 w918 w948 w1043 w1072 w1106 w1143 w1212 w1264 w1304 w1335 w1384 w1406 w1434 w1457 w1533 w1574 w1640 w1656 w1695 w1731 w1770 w1802 w1820 w1871 w1875 w1882 w1889]
      frame "Initialize" {
        n5 = call-poly "Enqueue Message.vi"("error in (no error)"=w25, "Message"="Initialize UI", "Message Queue"=w24) -> ("error out"=w28:errorcluster)  [unwired: 7 in, 1 out]
      }
      frame "Initialize UI" {
        n6 = Unbundle By Name(w32) -> ("UI"=w31:refnum<queue>)
        n7 = call-poly "Enqueue Message.vi"("error in (no error)"=w34, "Message"="Initialize", "Message Queue"=w31) -> ("error out"=w36:errorcluster)  [unwired: 7 in, 1 out]
      }
      frame "UI Initialized" {
        (unwired) "Timers Initialized" ("Message")
        n8 = call-poly "Enqueue Message.vi"("error in (no error)"=w40, "Message"="Initialize Engine", "Message Queue"=w42) -> ("error out"=w43:errorcluster)  [unwired: 7 in, 1 out]
      }
      frame "Initialize Engine" {
        w49 = T2 {"Run"=FALSE, "Pause"=FALSE, "Step Execution"=FALSE, "Ignore Error"=FALSE, "File name"="", "Program"=[], "Program PTR"=0, "Current Test"={"Thread ID"=0.0, "Mérésszám"="", "Mérés/Utasítás"="", "Command"={"Parancs"="", "Paraméter 1"="", "Paraméter 2"="", "Paraméter 3"="", "Paraméter 4"="", "Paraméter 5"="", "Eredmény"=""}, "Min"="", "Max"="", "Aktív?"=FALSE, "Log?"=FALSE, "Kiértékelés"=FALSE, "Etalon 1 exp"=FALSE, "Etalon 2 exp"=FALSE, "Etalon 3 exp"=FALSE, "Etalon 4 exp"=FALSE, "Etalon 5 exp"=FALSE}, "Error"={"status"=FALSE, "code"=0, "source"=""}, "Previous Test"={"Thread ID"=0.0, "Mérésszám"="", "Mérés/Utasítás"="", "Command"={"Parancs"="", "Paraméter 1"="", "Paraméter 2"="", "Paraméter 3"="", "Paraméter 4"="", "Paraméter 5"="", "Eredmény"=""}, "Min"="", "Max"="", "Aktív?"=FALSE, "Log?"=FALSE, "Kiértékelés"=FALSE, "Etalon 1 exp"=FALSE, "Etalon 2 exp"=FALSE, "Etalon 3 exp"=FALSE, "Etalon 4 exp"=FALSE, "Etalon 5 exp"=FALSE}, "Etalon number"=0, "Etalon error code"=0, "Meas Result"=FALSE, "Etalon Result"=FALSE, "Aborted"=FALSE, "Alaphelyzet"=FALSE, "Command"="", "Response"=""}  # Thread
        n9 = Bundle By Name(cluster=w49, "Alaphelyzet"=FALSE) -> (w47:T2)
        n10 = Initialize Array(w47, 10 ("dimension size")) -> (w55:T2[])
        n11 = call-poly "Enqueue Message.vi"("error in (no error)"=w46, "Message"="Initialize Ring", "Message Queue"=w51) -> ("error out"=w52:errorcluster)  [unwired: 7 in, 1 out]
      }
      frame "Initialize Ring" {
        n12 = Unbundle By Name(w59) -> ("UI"=w58:refnum<queue>)
        n13 = Unbundle By Name(w59) -> ("Ring"=w64:refnum<queue>)
        n14 = call-poly "Enqueue Message.vi"("error in (no error)"=w66, "Message"="Initialize", "Message Queue"=w64) -> ("error out"=w62:errorcluster)  [unwired: 7 in, 1 out]
        n15 = Wait (ms)(milliseconds to wait=u32 50) -> ()  [unwired: 1 out]
        n16 = call-poly "Enqueue Message.vi"("error in (no error)"=w62, "Message Data"=w61, "Message"="Set Statusbar", "Message Queue"=w58) -> ("error out"=w60:errorcluster)  [unwired: 6 in, 1 out]
      }
      frame "Ring initialized" {
        n17 = call-poly "Enqueue Message.vi"("error in (no error)"=w74, "Message"="Initialize DAQ", "Message Queue"=w72) -> ("error out"=w73:errorcluster)  [unwired: 7 in, 1 out]
      }
      frame "Initialize DAQ" {
        n18 = Unbundle By Name(w79) -> ("UI"=w78:refnum<queue>)
        n19 = Unbundle By Name(w79) -> ("DAQ"=w84:refnum<queue>)
        n20 = call-poly "Enqueue Message.vi"("error in (no error)"=w86, "Message"="Initialize", "Message Queue"=w84) -> ("error out"=w82:errorcluster)  [unwired: 7 in, 1 out]
        n21 = Wait (ms)(milliseconds to wait=u32 50) -> ()  [unwired: 1 out]
        n22 = call-poly "Enqueue Message.vi"("error in (no error)"=w82, "Message Data"=w81, "Message"="Set Statusbar", "Message Queue"=w78) -> ("error out"=w80:errorcluster)  [unwired: 6 in, 1 out]
      }
      frame "DAQ Initialized" {
        n23 = call-poly "Enqueue Message.vi"("error in (no error)"=w94, "Message"="Initialize Data Processor", "Message Queue"=w92) -> ("error out"=w93:errorcluster)  [unwired: 7 in, 1 out]
      }
      frame "Initialize Data Processor" {
        n24 = Unbundle By Name(w99) -> ("Data Processor"=w104:refnum<queue>)
        n25 = Unbundle By Name(w99) -> ("UI"=w98:refnum<queue>)
        n26 = call-poly "Enqueue Message.vi"("error in (no error)"=w106, "Message"="Initialize", "Message Queue"=w104) -> ("error out"=w102:errorcluster)  [unwired: 7 in, 1 out]
        n27 = Wait (ms)(milliseconds to wait=u32 50) -> ()  [unwired: 1 out]
        n28 = call-poly "Enqueue Message.vi"("error in (no error)"=w102, "Message Data"=w101, "Message"="Set Statusbar", "Message Queue"=w98) -> ("error out"=w100:errorcluster)  [unwired: 6 in, 1 out]
      }
      frame "Data Processor Initialized" {
        n29 = call-poly "Enqueue Message.vi"("error in (no error)"=w114, "Message"="Initialize Laser", "Message Queue"=w112) -> ("error out"=w113:errorcluster)  [unwired: 7 in, 1 out]
      }
      frame "Initialize Laser" {
        n30 = Unbundle By Name(w120) -> ("UI"=w122:refnum<queue>)
        n31 = Unbundle By Name(w120) -> ("Laser"=w124:refnum<queue>)
        n32 = call-poly "Enqueue Message.vi"("error in (no error)"=w126, "Message"="Initialize", "Message Queue"=w124) -> ("error out"=w119:errorcluster)  [unwired: 7 in, 1 out]
        n33 = call-poly "Enqueue Message.vi"("error in (no error)"=w119, "Message Data"=w121, "Message"="Set Statusbar", "Message Queue"=w122) -> ("error out"=w118:errorcluster)  [unwired: 6 in, 1 out]
        n34 = Wait (ms)(milliseconds to wait=u32 50) -> ()  [unwired: 1 out]
      }
      frame "Laser Initialized" {
        n35 = Unbundle By Name(w136) -> ("UI"=w135:refnum<queue>)
        n36 = call-poly "Enqueue Message.vi"("error in (no error)"=w137, "Message Data"="", "Message"="Set Statusbar", "Message Queue"=w135) -> ("error out"=w131:errorcluster)  [unwired: 6 in, 1 out]
        n37 = call-poly "Enqueue Message.vi"("error in (no error)"=w131, "Message"="Initialize Timers", "Message Queue"=w130) -> ("error out"=w132:errorcluster)  [unwired: 7 in, 1 out]
      }
      frame "Initialize Timers" {
        n38 = Unbundle By Name(w145) -> ("Timers"=w149:refnum<queue>)
        n39 = Unbundle By Name(w145) -> ("UI"=w147:refnum<queue>)
        n40 = call-poly "Enqueue Message.vi"("error in (no error)"=w151, "Message"="Initialize", "Message Queue"=w149) -> ("error out"=w144:errorcluster)  [unwired: 7 in, 1 out]
        n41 = call-poly "Enqueue Message.vi"("error in (no error)"=w144, "Message Data"=w146, "Message"="Set Statusbar", "Message Queue"=w147) -> ("error out"=w143:errorcluster)  [unwired: 6 in, 1 out]
        n42 = Wait (ms)(milliseconds to wait=u32 50) -> ()  [unwired: 1 out]
      }
      frame "Timers Initialized" {
        n43 = Unbundle By Name(w157) -> ("UI"=w156:refnum<queue>)
        n44 = call-poly "Enqueue Message.vi"("error in (no error)"=w158, "Message Data"="", "Message"="Set Statusbar", "Message Queue"=w156) -> ("error out"=w161:errorcluster)  [unwired: 6 in, 1 out]
      }
      frame "Set Product Variables" {
        n45 = Variant To Data(error in=w167, type=T5 {"Termék név"="", "Teszt szekvencia"=path "", "Etalonok száma"=0} ("Termék cluster"), Variant=w168) -> (data=w165:T5, error out=w166:errorcluster)
      }
      frame "Set Etalon" {
        w174 = u16 0 ("Thread ID")
        # "Több Thread esetén multiplikálni kell!"
        n46 = Unbundle By Name(w173) -> ("Etalonok száma"=w172:i8)
        n47 = Index Array(array=w178, index=w174) -> (element=w176:T2)
        n48 = Bundle By Name(cluster=w176, "Etalon number"=w172) -> (w179:T2)
        n49 = Replace Array Subset(array=w178, new element=w179, index=w174) -> (w177:T2[])
      }
      frame "Reset Etalon" {
        w183 = u16 0 ("Thread ID")
        # "Több Thread esetén multiplikálni kell!"
        n50 = Index Array(array=w187, index=w183) -> (element=w185:T2)
        n51 = Bundle By Name(cluster=w185, "Etalon number"=u32 0) -> (w188:T2)
        n52 = Replace Array Subset(array=w187, new element=w188, index=w183) -> (w186:T2[])
      }
      frame "Open Test Sequence" {
        w205 = T7 {"Thread ID"=0, "Callback"="", "Data"=variant, "Error"={"status"=FALSE, "code"=0, "source"=""}}  # Message
        w211 = T7 {"Thread ID"=0, "Callback"="", "Data"=variant, "Error"={"status"=FALSE, "code"=0, "source"=""}}  # Message
        # "Termékváltás után a gép\nvegye fel az alaphelyzetet!"
        n53 = Variant To Data(error in=w212, type=w211, Variant=w213) -> (data=w204:T7, error out=w208:errorcluster)
        n54 = Unbundle By Name(w204) -> ("Thread ID"=w202:u16, "Callback"=w203:string)
        n55 = Unbundle By Name(w204) -> ("Thread ID"=w210:u16)
        n56 = Unbundle By Name(w204) -> ("Data"=w209:variant)
        n57 = Variant To Data(error in=w208, type=path "" ("Teszt szekvencia"), Variant=w209) -> (data=w190:path, error out=w199:errorcluster)
        n58 = Index Array(array=w214, index=w210) -> (element=w196:T2)
        n59 = Strip Path(path=w190) -> (name=w197:string)  [unwired: 1 out]
        n60 = call "Read program file.vi"("error in (no error)"=w199, "selected path"=w190) -> ("error out"=w198:errorcluster, "Program out 2"=w192:T3[])  [unwired: 7 in, 1 out]
        n61 = Bundle By Name(cluster=w196, "Program"=w192, "File name"=w197, "Alaphelyzet"=FALSE) -> (w215:T2)
        n62 = Unbundle By Name(w207) -> ("UI"=w206:refnum<queue>)
        n63 = Replace Array Subset(array=w214, new element=w215, index=w210) -> (w200:T2[])
        n64 = Bundle By Name(cluster=w205, "Thread ID"=w202, "Data"=w200) -> (w201:T7)
        n65 = call-poly "Enqueue Message.vi"("error in (no error)"=w198, "Message Data"=w201, "Message"=w203, "Message Queue"=w206) -> ("error out"=w193:errorcluster)  [unwired: 6 in, 1 out]
      }
      frame "Delete Test Sequence" {
        w227 = T7 {"Thread ID"=0, "Callback"="", "Data"=variant, "Error"={"status"=FALSE, "code"=0, "source"=""}}  # Message
        w231 = T7 {"Thread ID"=0, "Callback"="", "Data"=variant, "Error"={"status"=FALSE, "code"=0, "source"=""}}  # Message
        n66 = Variant To Data(error in=w232, type=w231, Variant=w233) -> (data=w226:T7, error out=w219:errorcluster)
        n67 = Unbundle By Name(w226) -> ("Thread ID"=w224:u16, "Callback"=w225:string)
        n68 = Unbundle By Name(w226) -> ("Thread ID"=w230:u16)
        n69 = Index Array(array=w234, index=w230) -> (element=w236:T2)
        n70 = Bundle By Name(cluster=w236, "Program"=T3[] [], "File name"="Nincs betöltve...") -> (w235:T2)
        n71 = Replace Array Subset(array=w234, new element=w235, index=w230) -> (w221:T2[])
        n72 = Unbundle By Name(w229) -> ("UI"=w228:refnum<queue>)
        n73 = Bundle By Name(cluster=w227, "Thread ID"=w224, "Data"=w221) -> (w223:T7)
        n74 = call-poly "Enqueue Message.vi"("error in (no error)"=w219, "Message Data"=w223, "Message"=w225, "Message Queue"=w228) -> ("error out"=w222:errorcluster)  [unwired: 6 in, 1 out]
      }
      frame "Select Test Sequence" {
        w245 = T7 {"Thread ID"=0, "Callback"="", "Data"=variant, "Error"={"status"=FALSE, "code"=0, "source"=""}}  # Message
        w248 = T7 {"Thread ID"=0, "Callback"="", "Data"=variant, "Error"={"status"=FALSE, "code"=0, "source"=""}}  # Message
        # "Ha csak 1 thread van, ez nincs használva!"
        n75 = Variant To Data(error in=w249, type=w248, Variant=w250) -> (data=w244:T7)  [unwired: 1 out]
        n76 = Unbundle By Name(w244) -> ("Thread ID"=w242:u16, "Callback"=w243:string)
        n77 = Unbundle By Name(w247) -> ("UI"=w246:refnum<queue>)
        n78 = Bundle By Name(cluster=w245, "Thread ID"=w242, "Data"=w238) -> (w241:T7)
        n79 = call-poly "Enqueue Message.vi"("Message Data"=w241, "Message"=w243, "Message Queue"=w246) -> ("error out"=w240:errorcluster)  [unwired: 7 in, 1 out]
      }
      frame "Save Test Sequence" {
        w263 = T7 {"Thread ID"=0, "Callback"="", "Data"=variant, "Error"={"status"=FALSE, "code"=0, "source"=""}}  # Message
        w274 = T7 {"Thread ID"=0, "Callback"="", "Data"=variant, "Error"={"status"=FALSE, "code"=0, "source"=""}}  # Message
        n80 = Variant To Data(error in=w275, type=w274, Variant=w276) -> (data=w258:T7, error out=w272:errorcluster)
        n81 = Unbundle By Name(w258) -> ("Data"=w273:variant)
        n82 = Unbundle By Name(w258) -> ("Thread ID"=w257:u16, "Callback"=w256:string)
        n83 = Unbundle By Name(w258) -> ("Thread ID"=w253:u16)
        n84 = Variant To Data(error in=w272, type=path "", Variant=w273) -> (data=w267:path, error out=w270:errorcluster)
        n85 = Index Array(array=w255, index=w253) -> (element=w266:T2)
        n86 = Unbundle By Name(w266) -> ("Program"=w269:T3[])
        n87 = call "Write program file.vi"("error in"=w270, "Program in"=w269, "selected path"=w267) -> ("error out"=w260:errorcluster)  [unwired: 8 in]
        n88 = Strip Path(path=w267) -> (name=w265:string)  [unwired: 1 out]
        n89 = Bundle By Name(cluster=w266, "File name"=w265) -> (w254:T2)
        n90 = Replace Array Subset(array=w255, new element=w254, index=w253) -> (w252:T2[])
        n91 = Unbundle By Name(w261) -> ("UI"=w264:refnum<queue>)
        n92 = Bundle By Name(cluster=w263, "Thread ID"=w257, "Data"=w252) -> (w262:T7)
        n93 = call-poly "Enqueue Message.vi"("error in (no error)"=w260, "Message Data"=w262, "Message"=w256, "Message Queue"=w264) -> ("error out"=w259:errorcluster)  [unwired: 6 in, 1 out]
      }
      frame "Edit Test" {
        n94 = call "Teszt szerkesztõ2.vi"("Teszt cluster in"=w280) -> ("Teszt cluster out"=w279:T3)  [unwired: 10 in]
      }
      frame "Add Test" {
        w294 = T7 {"Thread ID"=0, "Callback"="", "Data"=variant, "Error"={"status"=FALSE, "code"=0, "source"=""}}  # Message
        w298 = T7 {"Thread ID"=0, "Callback"="", "Data"=variant, "Error"={"status"=FALSE, "code"=0, "source"=""}}  # Message
        n95 = Variant To Data(error in=w299, type=w298, Variant=w300) -> (data=w293:T7, error out=w283:errorcluster)
        n96 = Unbundle By Name(w293) -> ("Thread ID"=w291:u16, "Callback"=w292:string)
        n97 = Unbundle By Name(w293) -> ("Thread ID"=w297:u16)
        n98 = Index Array(array=w301, index=w297) -> (element=w287:T2)
        n99 = Unbundle By Name(w287) -> ("Program"=w286:T3[])
        n100 = Build Array (concatenate)(w286, w285) -> (w284:T3[])
        n101 = Bundle By Name(cluster=w287, "Program"=w284) -> (w302:T2)
        n102 = Replace Array Subset(array=w301, new element=w302, index=w297) -> (w288:T2[])
        n103 = Unbundle By Name(w296) -> ("UI"=w295:refnum<queue>)
        n104 = Bundle By Name(cluster=w294, "Thread ID"=w291, "Data"=w288) -> (w290:T7)
        n105 = call-poly "Enqueue Message.vi"("error in (no error)"=w283, "Message Data"=w290, "Message"=w292, "Message Queue"=w295) -> ("error out"=w289:errorcluster)  [unwired: 6 in, 1 out]
      }
      frame "Copy Test" {
        w315 = T7 {"Thread ID"=0, "Callback"="", "Data"=variant, "Error"={"status"=FALSE, "code"=0, "source"=""}}  # Message
        n106 = Variant To Data(error in=w316, type=w315, Variant=w317) -> (data=w312:T7, error out=w309:errorcluster)
        n107 = Unbundle By Name(w312) -> ("Thread ID"=w314:u16)
        n108 = Unbundle By Name(w312) -> ("Data"=w311:variant)
        n109 = Variant To Data(error in=w309, type=0, Variant=w311) -> (data=w307:i32, error out=w304:errorcluster)
        n110 = Index Array(array=w306, index=w314) -> (element=w313:T2)
        n111 = Unbundle By Name(w313) -> ("Program"=w308:T3[])
        n112 = Index Array(array=w308, index=w307) -> (element=w305:T3)
      }
      frame "Paste Test" {
        w334 = T7 {"Thread ID"=0, "Callback"="", "Data"=variant, "Error"={"status"=FALSE, "code"=0, "source"=""}}  # Message
        w338 = T7 {"Thread ID"=0, "Callback"="", "Data"=variant, "Error"={"status"=FALSE, "code"=0, "source"=""}}  # Message
        n113 = Variant To Data(error in=w339, type=w338, Variant=w340) -> (data=w325:T7, error out=w324:errorcluster)
        n114 = Unbundle By Name(w325) -> ("Thread ID"=w337:u16)
        n115 = Unbundle By Name(w325) -> ("Data"=w327:variant)
        n116 = Unbundle By Name(w325) -> ("Thread ID"=w332:u16, "Callback"=w333:string)
        n117 = Variant To Data(error in=w324, type=0, Variant=w327) -> (data=w322:i32, error out=w319:errorcluster)
        n118 = Index Array(array=w341, index=w337) -> (element=w328:T2)
        n119 = Unbundle By Name(w328) -> ("Program"=w323:T3[])
        n120 = Insert Into Array(array=w323, index=w322, new element=w321) -> (w320:T3[])
        n121 = Bundle By Name(cluster=w328, "Program"=w320) -> (w342:T2)
        n122 = Replace Array Subset(array=w341, new element=w342, index=w337) -> (w329:T2[])
        n123 = Unbundle By Name(w336) -> ("UI"=w335:refnum<queue>)
        n124 = Bundle By Name(cluster=w334, "Thread ID"=w332, "Data"=w329) -> (w331:T7)
        n125 = call-poly "Enqueue Message.vi"("error in (no error)"=w319, "Message Data"=w331, "Message"=w333, "Message Queue"=w335) -> ("error out"=w330:errorcluster)  [unwired: 6 in, 1 out]
      }
      frame "Modify Test" {
        w359 = T7 {"Thread ID"=0, "Callback"="", "Data"=variant, "Error"={"status"=FALSE, "code"=0, "source"=""}}  # Message
        w363 = T7 {"Thread ID"=0, "Callback"="", "Data"=variant, "Error"={"status"=FALSE, "code"=0, "source"=""}}  # Message
        n126 = Variant To Data(error in=w364, type=w363, Variant=w365) -> (data=w350:T7, error out=w349:errorcluster)
        n127 = Unbundle By Name(w350) -> ("Thread ID"=w362:u16)
        n128 = Unbundle By Name(w350) -> ("Data"=w352:variant)
        n129 = Unbundle By Name(w350) -> ("Thread ID"=w357:u16, "Callback"=w358:string)
        n130 = Variant To Data(error in=w349, type=0, Variant=w352) -> (data=w346:i32, error out=w348:errorcluster)
        n131 = Index Array(array=w366, index=w362) -> (element=w353:T2)
        n132 = Unbundle By Name(w353) -> ("Program"=w347:T3[])
        n133 = Replace Array Subset(array=w347, new element=w345, index=w346) -> (w344:T3[])
        n134 = Bundle By Name(cluster=w353, "Program"=w344) -> (w367:T2)
        n135 = Replace Array Subset(array=w366, new element=w367, index=w362) -> (w354:T2[])
        n136 = Unbundle By Name(w361) -> ("UI"=w360:refnum<queue>)
        n137 = Bundle By Name(cluster=w359, "Thread ID"=w357, "Data"=w354) -> (w356:T7)
        n138 = call-poly "Enqueue Message.vi"("error in (no error)"=w348, "Message Data"=w356, "Message"=w358, "Message Queue"=w360) -> ("error out"=w355:errorcluster)  [unwired: 6 in, 1 out]
      }
      frame "Delete Test" {
        w385 = T7 {"Thread ID"=0, "Callback"="", "Data"=variant, "Error"={"status"=FALSE, "code"=0, "source"=""}}  # Message
        w389 = T7 {"Thread ID"=0, "Callback"="", "Data"=variant, "Error"={"status"=FALSE, "code"=0, "source"=""}}  # Message
        n139 = Variant To Data(error in=w390, type=w389, Variant=w391) -> (data=w376:T7, error out=w375:errorcluster)
        n140 = Unbundle By Name(w376) -> ("Thread ID"=w388:u16)
        n141 = Unbundle By Name(w376) -> ("Data"=w378:variant)
        n142 = Unbundle By Name(w376) -> ("Thread ID"=w383:u16, "Callback"=w384:string)
        n143 = Variant To Data(error in=w375, type=0, Variant=w378) -> (data=w371:i32, error out=w374:errorcluster)
        n144 = Index Array(array=w392, index=w388) -> (element=w379:T2)
        n145 = Unbundle By Name(w379) -> ("Program"=w372:T3[])
        n146 = Delete From Array(array=w372, length=1, index=w371) -> (array with subset deleted=w369:T3[])  [unwired: 1 out]
        n147 = Bundle By Name(cluster=w379, "Program"=w369) -> (w393:T2)
        n148 = Replace Array Subset(array=w392, new element=w393, index=w388) -> (w380:T2[])
        n149 = Unbundle By Name(w387) -> ("UI"=w386:refnum<queue>)
        n150 = Bundle By Name(cluster=w385, "Thread ID"=w383, "Data"=w380) -> (w382:T7)
        n151 = call-poly "Enqueue Message.vi"("error in (no error)"=w374, "Message Data"=w382, "Message"=w384, "Message Queue"=w386) -> ("error out"=w381:errorcluster)  [unwired: 6 in, 1 out]
      }
      frame "Run" {
        w401 = T8 {"Thread ID"=0, "Thread Flag"=FALSE}  # Thread Flag
        n152 = Variant To Data(error in=w407, type=w401, Variant=w408) -> (data=w402:T8, error out=w400:errorcluster)
        n153 = Unbundle By Name(w402) -> ("Thread ID"=w403:u16, "Thread Flag"=w395:bool)
        n154 = Index Array(array=w394, index=w403) -> (element=w399:T2)
        n155 = Unbundle By Name(w399) -> ("Run"=w398:bool)
        n156 = case shown="False" w398 {
          tunnel: [w412 w429] -> w406
          tunnel: w405 -> [w411 w428]
          tunnel: w404 -> [w409 w426]
          tunnel: w402 -> [w410 w427]
          tunnel: w400 -> [w413 w430]
          tunnel: w395 -> [w414 w431]
          frame False {
            # "MÉRÉS NEM FUT"
            n157 = case shown="True" w414 {
              tunnel: w413 -> [w415 w418]
              tunnel: [w415 w425] -> w412
              tunnel: w411 -> [_ w424]
              tunnel: w410 -> [_ w423]
              tunnel: w409 -> [_ w421]
              frame False {
                # "SEMMI"
              }
              frame True {
                # "MÉRÉS INDÍTÁS"
                n158 = Unbundle By Name(w423) -> ("Thread ID"=w422:u16)
                n159 = Unbundle By Name(w421) -> ("Ring"=w419:refnum<queue>)
                n160 = call-poly "Enqueue Message.vi"("error in (no error)"=w418, "Message"="Home", "Message Queue"=w419) -> ("error out"=w417:errorcluster)  [unwired: 7 in, 1 out]
                n161 = call-poly "Enqueue Message.vi"("error in (no error)"=w417, "Message Data"=w422, "Message"="Engine Start", "Message Queue"=w424) -> ("error out"=w425:errorcluster)  [unwired: 6 in, 1 out]
              }
            }
          }
          frame True {
            # "MÉRÉS FUT"
            n162 = case shown="False" w431 {
              tunnel: w430 -> [w434 w440]
              tunnel: [w439 w440] -> w429
              tunnel: w428 -> [w438 _]
              tunnel: w427 -> [w437 _]
              tunnel: w426 -> [w436 _]
              frame False {
                w435 = "Abort" ("Message")
                # "MÉRÉS MEGÁLLÍTÁS"
                n163 = call "Enqueue Message to all_.vi"("Priority Message? (F)"=TRUE, "error in (no error)"=w434, "Message"=w435, "Message Queues in"=w436) -> ("error out"=w433:errorcluster)  [unwired: 7 in]
                n164 = call-poly "Enqueue Message.vi"("error in (no error)"=w433, "Message Data"=w437, "Message"=w435, "Message Queue"=w438) -> ("error out"=w439:errorcluster)  [unwired: 6 in, 1 out]
              }
              frame True {
                # "SEMMI, KÉTSZERI GOMBNYOMÁS"
              }
            }
          }
        }
      }
      frame "Abort" {
        w453 = T8 {"Thread ID"=0, "Thread Flag"=FALSE}  # Thread Flag
        w464 = "ENGINE Jump" ("Command.Parancs")
        w461 = T3 {"Thread ID"=0.0, "Mérésszám"="", "Mérés/Utasítás"="", "Command"={"Parancs"="", "Paraméter 1"="", "Paraméter 2"="", "Paraméter 3"="", "Paraméter 4"="", "Paraméter 5"="", "Eredmény"=""}, "Min"="", "Max"="", "Aktív?"=FALSE, "Log?"=FALSE, "Kiértékelés"=FALSE, "Etalon 1 exp"=FALSE, "Etalon 2 exp"=FALSE, "Etalon 3 exp"=FALSE, "Etalon 4 exp"=FALSE, "Etalon 5 exp"=FALSE}  # Teszt cluster
        w462 = T7 {"Thread ID"=0, "Callback"="", "Data"=variant, "Error"={"status"=FALSE, "code"=0, "source"=""}}  # Message
        n165 = Variant To Data(error in=w452, type=w453, Variant=w451) -> (data=w450:T8, error out=w445:errorcluster)
        n166 = Unbundle By Name(w450) -> ("Thread ID"=w444:u16)
        n167 = flat-sequence {
          tunnel: w445 -> [w475]
          tunnel: [w475] -> w449
          frame #0 {
            n168 = Wait (ms)(milliseconds to wait=u32 200) -> ()  [unwired: 1 out]
          }
        }
        n169 = Index Array(array=w456, index=w444) -> (element=w458:T2)
        n170 = Bundle By Name(cluster=w458, "Aborted"=TRUE, "Etalon Result"=FALSE ("Alaphelyzet"), "Meas Result"=FALSE ("Aborted")) -> (w455:T2)
        n171 = Equal To 0?(x=w444) -> (x = 0?=w443:bool)
        n172 = case shown="False" w443 {
          tunnel: w449 -> [w468 w473]
          tunnel: w448 -> [w469 w472]
          tunnel: [w468 w471] -> w447
          tunnel: [w469 w470] -> w446
          frame False {
          }
          frame True {
            n173 = Flush Queue(queue=w472, error in (no error)=w473) -> (queue out=w470:refnum<queue>, error out=w471:errorcluster)  [unwired: 1 out]
          }
        }
        n174 = Replace Array Subset(array=w456, new element=w455, index=w444) -> (w454:T2[])
        n175 = Bundle By Name(cluster=w461, "Command.Parancs"=w464, "Command.Paraméter 1"="ABORT") -> (w459:T3)
        n176 = Bundle By Name(cluster=w462, "Thread ID"=w444, "Data"=w459) -> (w463:T7)
        n177 = call-poly "Enqueue Message.vi"("error in (no error)"=w447, "Message Data"=w463, "Message"=w464, "Message Queue"=w446) -> ("error out"=w467:errorcluster)  [unwired: 6 in, 1 out]
      }
      frame "Pause" {
        w488 = T8 {"Thread ID"=0, "Thread Flag"=FALSE}  # Thread Flag
        n178 = Variant To Data(error in=w494, type=w488, Variant=w495) -> (data=w483:T8, error out=w481:errorcluster)
        n179 = Unbundle By Name(w483) -> ("Thread ID"=w492:u16, "Thread Flag"=w484:bool)
        n180 = Unbundle By Name(w483) -> ("Thread ID"=w482:u16)
        n181 = Index Array(array=w490, index=w492) -> (element=w493:T2)
        n182 = case shown="False" w484 {
          tunnel: w485 -> [w499 _]
          tunnel: w482 -> [w498 _]
          tunnel: w481 -> [w497 w504]
          tunnel: [w496 w504] -> w480
          frame False {
            w501 = T7 {"Thread ID"=0, "Callback"="", "Data"=variant, "Error"={"status"=FALSE, "code"=0, "source"=""}}  # Message
            n183 = Unbundle By Name(w499) -> ("UI"=w503:refnum<queue>)
            n184 = Bundle By Name(cluster=w501, "Thread ID"=w498) -> (w500:T7)
            n185 = call-poly "Enqueue Message.vi"("error in (no error)"=w497, "Message Data"=w500, "Message"="Mérés Continue UI", "Message Queue"=w503) -> ("error out"=w496:errorcluster)  [unwired: 6 in, 1 out]
          }
          frame True {
          }
        }
        n186 = Bundle By Name(cluster=w493, "Pause"=w484) -> (w491:T2)
        n187 = Replace Array Subset(array=w490, new element=w491, index=w492) -> (w489:T2[])
        n188 = Unbundle By Name(w483) -> ("Thread ID"=w476:u16)
        n189 = call-poly "Enqueue Message.vi"("error in (no error)"=w480, "Message Data"=w476, "Message"="Select Test", "Message Queue"=w486) -> ("error out"=w487:errorcluster)  [unwired: 6 in, 1 out]
      }
      frame "Step Execution" {
        w509 = T8 {"Thread ID"=0, "Thread Flag"=FALSE}  # Thread Flag
        n190 = Variant To Data(error in=w516, type=w509, Variant=w517) -> (data=w510:T8, error out=w507:errorcluster)
        n191 = Unbundle By Name(w510) -> ("Thread ID"=w514:u16, "Thread Flag"=w508:bool)
        n192 = Index Array(array=w512, index=w514) -> (element=w515:T2)
        n193 = Bundle By Name(cluster=w515, "Step Execution"=w508) -> (w513:T2)
        n194 = Replace Array Subset(array=w512, new element=w513, index=w514) -> (w511:T2[])
      }
      frame "Ignore Error" {
        w522 = T8 {"Thread ID"=0, "Thread Flag"=FALSE}  # Thread Flag
        n195 = Variant To Data(error in=w529, type=w522, Variant=w530) -> (data=w523:T8, error out=w520:errorcluster)
        n196 = Unbundle By Name(w523) -> ("Thread ID"=w527:u16, "Thread Flag"=w521:bool)
        n197 = Index Array(array=w525, index=w527) -> (element=w528:T2)
        n198 = Bundle By Name(cluster=w528, "Ignore Error"=w521) -> (w526:T2)
        n199 = Replace Array Subset(array=w525, new element=w526, index=w527) -> (w524:T2[])
      }
      frame "Engine Start" {
        w537 = TRUE ("Meas Result")
        w539 = T3 {"Thread ID"=0.0, "Mérésszám"="", "Mérés/Utasítás"="", "Command"={"Parancs"="", "Paraméter 1"="", "Paraméter 2"="", "Paraméter 3"="", "Paraméter 4"="", "Paraméter 5"="", "Eredmény"=""}, "Min"="", "Max"="", "Aktív?"=FALSE, "Log?"=FALSE, "Kiértékelés"=FALSE, "Etalon 1 exp"=FALSE, "Etalon 2 exp"=FALSE, "Etalon 3 exp"=FALSE, "Etalon 4 exp"=FALSE, "Etalon 5 exp"=FALSE}  # Current Test
        w545 = T7 {"Thread ID"=0, "Callback"="", "Data"=variant, "Error"={"status"=FALSE, "code"=0, "source"=""}}  # Message
        w556 = u16 0  # Thread ID
        n200 = Variant To Data(error in=w557, type=w556, Variant=w558) -> (data=w541:u16, error out=w543:errorcluster)
        n201 = Index Array(array=w553, index=w541) -> (element=w533:T2)
        n202 = Unbundle By Name(w533) -> ("Run"=w534:bool)
        n203 = case shown="False" w534 {
          tunnel: w533 -> [w559 w562]
          tunnel: [w559 w560] -> w532
          frame True {
          }
          frame False {
            w561 = ""
            n204 = Bundle By Name(cluster=w562, "Command"=w561, "Response"=w561) -> (w560:T2)
          }
        }
        n205 = Unbundle By Name(w546) -> ("UI"=w548:refnum<queue>)
        n206 = Bundle By Name(cluster=w545, "Thread ID"=w541) -> (w544:T7)
        n207 = call-poly "Enqueue Message.vi"("error in (no error)"=w543, "Message Data"=w544, "Message"="Mérés Start UI", "Message Queue"=w548) -> ("error out"=w542:errorcluster)  [unwired: 6 in, 1 out]
        n208 = Bundle By Name(cluster=w532, "Program PTR"=u32 0, "Pause"=FALSE, "Current Test"=w539, "Previous Test"=w539, "Meas Result"=w537, "Etalon Result"=w537, "Aborted"=FALSE, "Run"=TRUE) -> (w531:T2)
        n209 = Replace Array Subset(array=w553, new element=w531, index=w541) -> (w552:T2[])
        n210 = call-poly "Enqueue Message.vi"("error in (no error)"=w542, "Message Data"=w541, "Message"="Select Test", "Message Queue"=w549) -> ("error out"=w551:errorcluster)  [unwired: 6 in, 1 out]
      }
      frame "Select Test" {
        w568 = u16 0  # Thread ID
        # "OK, de még ki kell egészíteni"
        n211 = Variant To Data(error in=w575, type=w568, Variant=w576) -> (data=w566:u16, error out=w565:errorcluster)
        n212 = Index Array(array=w570, index=w566) -> (element=w572:T2)
        n213 = Unbundle By Name(w572) -> ("Run"=w577:bool, "Pause"=w578:bool, "Step Execution"=w579:bool, "Program PTR"=w580:u32, "Program"=w574:T3[])
        n214 = Array Size(array=w574) -> (size(s)=w573:i32)
        n215 = case shown="True" w577 {
          tunnel: w582 -> [w587 w600]
          tunnel: [w588 w598] -> w581
          tunnel: w580 -> [_ w594]
          tunnel: w579 -> [_ w593]
          tunnel: w578 -> [_ w597]
          tunnel: w573 -> [_ w596]
          tunnel: w572 -> [w585 w595]
          tunnel: [w585 w592] -> w569
          tunnel: w567 -> [_ w591]
          tunnel: w566 -> [w583 w590]
          tunnel: w565 -> [w584 w589]
          frame False {
            # "ENGINE NEM FUT"
            n216 = call-poly "Enqueue Message.vi"("error in (no error)"=w584, "Message Data"=w583, "Message"="Meas End", "Message Queue"=w587) -> ("error out"=w588:errorcluster)  [unwired: 6 in, 1 out]
          }
          frame True {
            # "ENGINE FUT"
            n217 = Less?(x=w594, y=w596) -> (x < y?=w599:bool)
            n218 = case shown="True" w593 {
              tunnel: w600 -> [w608 w649]
              tunnel: w599 -> [w607 w650]
              tunnel: [w606 w648] -> w598
              tunnel: w597 -> [_ w647]
              tunnel: w595 -> [w605 w646]
              tunnel: [w604 w645] -> w592
              tunnel: w591 -> [w603 w644]
              tunnel: w590 -> [w601 w643]
              tunnel: w589 -> [w602 w642]
              frame False {
                # "FOLYAMATOS MÉRÉS"
                n219 = case shown="True" w607 {
                  tunnel: w608 -> [w614 w616]
                  tunnel: [w612 w621] -> w606
                  tunnel: w605 -> [w611 w623]
                  tunnel: [w611 w617] -> w604
                  tunnel: w603 -> [_ w622]
                  tunnel: w602 -> [w610 w624]
                  tunnel: w601 -> [w609 w620]
                  frame False {
                    (unwired) "Score" ("Message")
                    # "TESZT VEKTOR VÉGE"
                    n220 = call-poly "Enqueue Message.vi"("error in (no error)"=w610, "Message Data"=w609, "Message"="Meas End", "Message Queue"=w614) -> ("error out"=w612:errorcluster)  [unwired: 6 in, 1 out]
                  }
                  frame True {
                    # "TESZT KIVÁLASZTÁSA"
                    n221 = call "Select Test.vi"("Thread in"=w623) -> ("Aktív?"=w615:bool, "Current Test"=w619:T3, "Thread out"=w618:T2)  [unwired: 7 in, 1 out]
                    n222 = case shown="True" w615 {
                      tunnel: w624 -> [w628 w641]
                      tunnel: w622 -> [_ w640]
                      tunnel: [w627 w639] -> w621
                      tunnel: w620 -> [w625 w634]
                      tunnel: w619 -> [_ w632]
                      tunnel: w618 -> [w630 w631]
                      tunnel: [w630 w631] -> w617
                      tunnel: w616 -> [w626 _]
                      frame False {
                        n223 = call-poly "Enqueue Message.vi"("error in (no error)"=w628, "Message Data"=w625, "Message"="Step Up PTR", "Message Queue"=w626) -> ("error out"=w627:errorcluster)  [unwired: 6 in, 1 out]
                      }
                      frame True {
                        w635 = T7 {"Thread ID"=0, "Callback"="", "Data"=variant, "Error"={"status"=FALSE, "code"=0, "source"=""}}  # Message
                        # "Ide fel kell még venni mindent!"
                        n224 = call "Send Command.vi"("error in (no error)"=w641, "Thread ID"=w634, "Message Queues"=w640, "Current Test"=w632) -> ("error out"=w638:errorcluster)  [unwired: 7 in]
                        n225 = Bundle By Name(cluster=w635, "Thread ID"=w634, "Data"=w632) -> (w633:T7)
                        n226 = Unbundle By Name(w640) -> ("UI"=w637:refnum<queue>)
                        n227 = call-poly "Enqueue Message.vi"("error in (no error)"=w638, "Message Data"=w633, "Message"="Set Meas Statusbar", "Message Queue"=w637) -> ("error out"=w639:errorcluster)  [unwired: 6 in, 1 out]
                      }
                    }
                  }
                }
              }
              frame True {
                # "LÉPÉSENKÉNTI MÉRÉS"
                n228 = case shown="False" w647 {
                  tunnel: w650 -> [w658 _]
                  tunnel: w649 -> [w657 _]
                  tunnel: [w656 w693] -> w648
                  tunnel: w646 -> [w655 w700]
                  tunnel: [w654 w700] -> w645
                  tunnel: w644 -> [w653 w696]
                  tunnel: w643 -> [w652 w695]
                  tunnel: w642 -> [w651 w694]
                  frame False {
                    # "KÖVETKEZÕ MÉRÉS"
                    n229 = case shown="True" w658 {
                      tunnel: w657 -> [w664 w666]
                      tunnel: [w662 w672] -> w656
                      tunnel: w655 -> [w661 w674]
                      tunnel: [w661 w667] -> w654
                      tunnel: w653 -> [_ w671]
                      tunnel: w652 -> [w659 w669]
                      tunnel: w651 -> [w660 w673]
                      frame False {
                        (unwired) "Score" ("Message")
                        # "TESZT VEKTOR VÉGE"
                        n230 = call-poly "Enqueue Message.vi"("error in (no error)"=w660, "Message Data"=w659, "Message"="Meas End", "Message Queue"=w664) -> ("error out"=w662:errorcluster)  [unwired: 6 in, 1 out]
                      }
                      frame True {
                        # "TESZT KIVÁLASZTÁSA"
                        n231 = call "Select Test.vi"("Thread in"=w674) -> ("Aktív?"=w665:bool, "Current Test"=w670:T3, "Thread out"=w668:T2)  [unwired: 7 in, 1 out]
                        n232 = case shown="True" w665 {
                          tunnel: w673 -> [w679 w691]
                          tunnel: [w678 w686] -> w672
                          tunnel: w671 -> [_ w684]
                          tunnel: w670 -> [_ w683]
                          tunnel: w669 -> [w676 w682]
                          tunnel: w668 -> [w675 w681]
                          tunnel: [w675 w681] -> w667
                          tunnel: w666 -> [w677 _]
                          frame False {
                            n233 = call-poly "Enqueue Message.vi"("error in (no error)"=w679, "Message Data"=w676, "Message"="Step Up PTR", "Message Queue"=w677) -> ("error out"=w678:errorcluster)  [unwired: 6 in, 1 out]
                          }
                          frame True {
                            w688 = T7 {"Thread ID"=0, "Callback"="", "Data"=variant, "Error"={"status"=FALSE, "code"=0, "source"=""}}  # Message
                            n234 = call "Send Command.vi"("error in (no error)"=w691, "Thread ID"=w682, "Message Queues"=w684, "Current Test"=w683) -> ("error out"=w685:errorcluster)  [unwired: 7 in]
                            n235 = Bundle By Name(cluster=w688, "Thread ID"=w682, "Data"=w683) -> (w687:T7)
                            n236 = Unbundle By Name(w684) -> ("UI"=w690:refnum<queue>)
                            n237 = call-poly "Enqueue Message.vi"("error in (no error)"=w685, "Message Data"=w687, "Message"="Set Meas Statusbar", "Message Queue"=w690) -> ("error out"=w686:errorcluster)  [unwired: 6 in, 1 out]
                          }
                        }
                      }
                    }
                  }
                  frame True {
                    w698 = T7 {"Thread ID"=0, "Callback"="", "Data"=variant, "Error"={"status"=FALSE, "code"=0, "source"=""}}  # Message
                    # "PAUSE ÁLLAPOT"
                    n238 = Unbundle By Name(w696) -> ("UI"=w699:refnum<queue>)
                    n239 = Bundle By Name(cluster=w698, "Thread ID"=w695) -> (w697:T7)
                    n240 = call-poly "Enqueue Message.vi"("error in (no error)"=w694, "Message Data"=w697, "Message"="Mérés Pause UI", "Message Queue"=w699) -> ("error out"=w693:errorcluster)  [unwired: 6 in, 1 out]
                  }
                }
              }
            }
          }
        }
        n241 = Replace Array Subset(array=w570, new element=w569, index=w566) -> (w571:T2[])
      }
      frame "DAQ Result", "DATAPROC Result", "ENGINE Result", "LASER Result", "TIMER Result" {
        w719 = T3 {"Thread ID"=0.0, "Mérésszám"="", "Mérés/Utasítás"="", "Command"={"Parancs"="", "Paraméter 1"="", "Paraméter 2"="", "Paraméter 3"="", "Paraméter 4"="", "Paraméter 5"="", "Eredmény"=""}, "Min"="", "Max"="", "Aktív?"=FALSE, "Log?"=FALSE, "Kiértékelés"=FALSE, "Etalon 1 exp"=FALSE, "Etalon 2 exp"=FALSE, "Etalon 3 exp"=FALSE, "Etalon 4 exp"=FALSE, "Etalon 5 exp"=FALSE}  # Teszt cluster
        w725 = T7 {"Thread ID"=0, "Callback"="", "Data"=variant, "Error"={"status"=FALSE, "code"=0, "source"=""}}  # Message
        n242 = Variant To Data(error in=w726, type=w725, Variant=w727) -> (data=w707:T7, error out=w723:errorcluster)
        n243 = Unbundle By Name(w707) -> ("Thread ID"=w711:u16, "Data"=w724:variant, "Error"=w722:errorcluster)
        n244 = Unbundle By Name(w716) -> ("UI"=w701:refnum<queue>)
        n245 = Index Array(array=w710, index=w711) -> (element=w713:T2)
        n246 = Variant To Data(error in=w723, type=w719, Variant=w724) -> (data=w709:T3, error out=w717:errorcluster)
        n247 = disable-structure shown="Disabled" {
          disable-tunnel: w717 -> [w732 w733]
          disable-tunnel: [w730 w733] -> w715
          disable-tunnel: w707 -> [w729 _]
          disable-tunnel: w701 -> [w728 _]
          frame Disabled {
            n248 = call-poly "Enqueue Message.vi"("error in (no error)"=w732, "Message Data"=w729, "Message"="Méréseredmény UI", "Message Queue"=w728) -> ("error out"=w730:errorcluster)  [unwired: 6 in, 1 out]
          }
          frame Enabled {
          }
        }
        n249 = case shown="No Error" w722 {
          selector: w722 -> [_ w756]
          tunnel: w713 -> [w737 w757]
          tunnel: w709 -> [w748 w755]
          tunnel: [w754 w758] -> w720
          tunnel: [w753 w756] -> w705
          tunnel: w718 -> [w752 _]
          tunnel: w711 -> [w751 _]
          tunnel: w715 -> [w750 _]
          tunnel: [w746 w755] -> w708
          frame No Error {
            n250 = Unbundle By Name(w737) -> ("Etalon number"=w745:u32, "Ignore Error"=w740:bool, "Aborted"=w739:bool)
            n251 = Or(x=w740, y=w739) -> (x .or. y?=w738:bool)
            n252 = call "Test Line Result.vi"("Etalon number"=w745, "Ignore Error"=w738, "error in (no error)"=w750, "Teszt cluster"=w748, "Thread ID"=w751, "Queue in"=w752) -> ("error out"=w753:errorcluster, "Abort"=w735:bool, "Etalon Kiértékelés"=w741:bool, "Kiértékelés"=w747:bool)  [unwired: 2 in]
            n253 = Unbundle By Name(w737) -> ("Etalon Result"=w743:bool)
            n254 = Unbundle By Name(w737) -> ("Meas Result"=w749:bool)
            n255 = Unbundle By Name(w737) -> ("Aborted"=w736:bool)
            n256 = And(x=w749, y=w747) -> (x .and. y?=w744:bool)
            n257 = And(x=w743, y=w741) -> (x .and. y?=w742:bool)
            n258 = Or(x=w736, y=w735) -> (x .or. y?=w734:bool)
            n259 = Bundle By Name(cluster=w748, "Kiértékelés"=w747) -> (w746:T3)
            n260 = Bundle By Name(cluster=w737, "Current Test"=w748, "Meas Result"=w744, "Etalon Result"=w742, "Aborted"=w734) -> (w754:T2)
          }
          frame Error {
            # "Ezt ki kell még találni!"
            n261 = Bundle By Name(cluster=w757, "Current Test"=w755) -> (w758:T2)
          }
        }
        n262 = To Variant(anything=w708) -> (Variant=w702:variant)
        n263 = Bundle By Name(cluster=w707, "Data"=w702) -> (w703:T7)
        n264 = call-poly "Enqueue Message.vi"("error in (no error)"=w705, "Message Data"=w703, "Message"="Méréseredmény UI", "Message Queue"=w701) -> ("error out"=w704:errorcluster)  [unwired: 6 in, 1 out]
        n265 = Replace Array Subset(array=w710, new element=w720, index=w711) -> (w721:T2[])
      }
      frame "Step Up PTR" {
        w775 = u16 0  # Thread ID
        n266 = Variant To Data(error in=w773, type=w775, Variant=w774) -> (data=w764:u16, error out=w765:errorcluster)
        n267 = Index Array(array=w770, index=w764) -> (element=w762:T2)
        n268 = Unbundle By Name(w762) -> ("Program PTR"=w772:u32, "Step Execution"=w761:bool)
        n269 = Increment(x=w772) -> (x+1=w771:u32)
        n270 = Bundle By Name(cluster=w762, "Program PTR"=w771, "Pause"=w761) -> (w768:T2)
        n271 = call-poly "Enqueue Message.vi"("error in (no error)"=w765, "Message Data"=w764, "Message"="Select Test", "Message Queue"=w766) -> ("error out"=w767:errorcluster)  [unwired: 6 in, 1 out]
        n272 = Replace Array Subset(array=w770, new element=w768, index=w764) -> (w769:T2[])
      }
      frame "Score" {
        w786 = T7 {"Thread ID"=0, "Callback"="", "Data"=variant, "Error"={"status"=FALSE, "code"=0, "source"=""}}  # Message
        w792 = u16 0  # Thread ID
        # "NINCS HASZNÁLVA"
        n273 = Variant To Data(error in=w790, type=w792, Variant=w791) -> (data=w782:u16, error out=w789:errorcluster)
        n274 = Index Array(array=w783, index=w782) -> (element=w781:T2)
        n275 = Unbundle By Name(w781) -> ("Etalon number"=w776:u32)
        n276 = Unbundle By Name(w781) -> ("Meas Result"=w780:bool, "Etalon Result"=w777:bool)
        n277 = Bundle By Name(cluster=w786, "Thread ID"=w782, "Data"=w780) -> (w785:T7)
        n278 = Greater Than 0?(x=w776) -> (x > 0?=w778:bool)
        n279 = case shown="True" w778 {
          selector: w778 -> [_ w825]
          tunnel: w789 -> [w804 w823]
          tunnel: [w803 w827] -> w793
          tunnel: w795 -> [w802 w826]
          tunnel: w794 -> [w801 w824]
          tunnel: w780 -> [w800 _]
          tunnel: w781 -> [w799 w821]
          tunnel: [w798 w822] -> w787
          tunnel: w782 -> [w797 w819]
          tunnel: w785 -> [w796 w820]
          tunnel: w779 -> [_ w818]
          tunnel: w777 -> [_ w817]
          frame False {
            # "TERMÉK MÉRÉS"
            n280 = case shown="False" w800 {
              tunnel: [w810 w814] -> w803
              tunnel: w804 -> [w805 w812]
              tunnel: w802 -> [_ _]
              tunnel: w801 -> [w806 w811]
              tunnel: w799 -> [w808 w813]
              tunnel: [w808 w813] -> w798
              tunnel: w797 -> [w807 w815]
              tunnel: w796 -> [_ _]
              frame True {
                # "TERMÉK OK"
                n281 = call-poly "Enqueue Message.vi"("error in (no error)"=w805, "Message Data"=w807, "Message"="Meas End", "Message Queue"=w806) -> ("error out"=w810:errorcluster)  [unwired: 6 in, 1 out]
              }
              frame False {
                # "TERMÉK NEM OK"
                n282 = call-poly "Enqueue Message.vi"("error in (no error)"=w812, "Message Data"=w815, "Message"="Meas End", "Message Queue"=w811) -> ("error out"=w814:errorcluster)  [unwired: 6 in, 1 out]
              }
            }
          }
          frame True {
            # "ETALON MÉRÉS"
            n283 = case shown="True" w817 {
              tunnel: [w828 w849] -> w827
              tunnel: w826 -> [w829 w850]
              tunnel: w825 -> [_ _]
              tunnel: w824 -> [w833 w854]
              tunnel: w823 -> [w831 w852]
              tunnel: [w836 w845] -> w822
              tunnel: w821 -> [w836 w846]
              tunnel: w820 -> [w832 w853]
              tunnel: w819 -> [w830 w851]
              tunnel: w818 -> [_ _]
              frame False {
                # "ETALON NEM OK"
                n284 = disable-structure shown="Disabled" {
                  disable-tunnel: [w840 w843] -> w835
                  disable-tunnel: w832 -> [w839 _]
                  disable-tunnel: w831 -> [w838 w843]
                  disable-tunnel: w829 -> [w837 _]
                  frame Disabled {
                    n285 = Unbundle By Name(w837) -> ("UI"=w841:refnum<queue>)
                    n286 = call-poly "Enqueue Message.vi"("error in (no error)"=w838, "Message Data"=w839, "Message"="Kiértékelés UI", "Message Queue"=w841) -> ("error out"=w840:errorcluster)  [unwired: 6 in, 1 out]
                  }
                  frame Enabled {
                  }
                }
                n287 = call-poly "Enqueue Message.vi"("error in (no error)"=w835, "Message Data"=w830, "Message"="Meas End", "Message Queue"=w833) -> ("error out"=w828:errorcluster)  [unwired: 6 in, 1 out]
              }
              frame True {
                # "ETALON OK"
                n288 = disable-structure shown="Disabled" {
                  disable-tunnel: w853 -> [w862 _]
                  disable-tunnel: w852 -> [w861 w865]
                  disable-tunnel: w850 -> [w860 _]
                  disable-tunnel: [w856 w865] -> w844
                  frame Disabled {
                    # "Hogy ne számolja a számláló az etalont"
                    n289 = Unbundle By Name(w860) -> ("UI"=w863:refnum<queue>)
                    n290 = call-poly "Enqueue Message.vi"("error in (no error)"=w861, "Message Data"=w862, "Message"="Kiértékelés UI", "Message Queue"=w863) -> ("error out"=w859:errorcluster, "dup Message Queue"=w858:refnum<queue>)  [unwired: 6 in]
                    n291 = call-poly "Enqueue Message.vi"("error in (no error)"=w859, "Message"="Reset Result Number Variables", "Message Queue"=w858) -> ("error out"=w856:errorcluster)  [unwired: 7 in, 1 out]
                  }
                  frame Enabled {
                  }
                }
                n292 = Unbundle By Name(w846) -> ("Etalon number"=w848:u32)
                n293 = Decrement(x=w848) -> (x-1=w847:u32)
                n294 = Bundle By Name(cluster=w846, "Etalon number"=w847) -> (w845:T2)
                n295 = call-poly "Enqueue Message.vi"("error in (no error)"=w844, "Message Data"=w851, "Message"="Meas End", "Message Queue"=w854) -> ("error out"=w849:errorcluster)  [unwired: 6 in, 1 out]
              }
            }
          }
        }
        n296 = Replace Array Subset(array=w783, new element=w787, index=w782) -> (w788:T2[])
      }
      frame "Meas End" {
        w882 = u16 0  # Thread ID
        n297 = Variant To Data(error in=w880, type=w882, Variant=w881) -> (data=w875:u16, error out=w879:errorcluster)
        n298 = Index Array(array=w876, index=w875) -> (element=w868:T2)
        n299 = Unbundle By Name(w868) -> ("Etalon number"=w871:u32, "Etalon Result"=w869:bool)
        n300 = Unbundle By Name(w868) -> ("Run"=w872:bool)
        n301 = Greater Than 0?(x=w871) -> (x > 0?=w870:bool)
        n302 = And(x=w870, y=w869) -> (x .and. y?=w867:bool)
        n303 = case shown="False" w872 {
          tunnel: [w894 w910] -> w883
          tunnel: w879 -> [w893 w903]
          tunnel: w884 -> [w895 w911]
          tunnel: w878 -> [_ w907]
          tunnel: w875 -> [w891 w905]
          frame False {
            w892 = T7 {"Thread ID"=0, "Callback"="", "Data"=variant, "Error"={"status"=FALSE, "code"=0, "source"=""}}  # Message
            # "ENGINE LEÁLL"
            n304 = Unbundle By Name(w895) -> ("UI"=w896:refnum<queue>)
            n305 = Bundle By Name(cluster=w892, "Thread ID"=w891) -> (w890:T7)
            n306 = call-poly "Enqueue Message.vi"("error in (no error)"=w893, "Message Data"=w890, "Message"="Mérés Vége UI", "Message Queue"=w896) -> ("error out"=w894:errorcluster)  [unwired: 6 in, 1 out]
          }
          frame True {
            w908 = T7 {"Thread ID"=0, "Callback"="", "Data"=variant, "Error"={"status"=FALSE, "code"=0, "source"=""}}  # Message
            # "ENGINE TOVÁBB FUT"
            n307 = Unbundle By Name(w911) -> ("UI"=w900:refnum<queue>)
            n308 = Bundle By Name(cluster=w908, "Thread ID"=w905) -> (w899:T7)
            n309 = flat-sequence {
              tunnel: w907 -> [w917]
              tunnel: [w917] -> w906
              tunnel: w905 -> [w916]
              tunnel: [w916] -> w904
              tunnel: w903 -> [w915]
              tunnel: [w915] -> w902
              tunnel: [w913] -> w898
              tunnel: w899 -> [w913]
              frame #0 {
                n310 = Wait (ms)(milliseconds to wait=u32 1000) -> ()  [unwired: 1 out]
              }
            }
            n311 = call-poly "Enqueue Message.vi"("error in (no error)"=w902, "Message Data"=w898, "Message"="Mérés Start UI", "Message Queue"=w900) -> ("error out"=w901:errorcluster)  [unwired: 6 in, 1 out]
            n312 = call-poly "Enqueue Message.vi"("error in (no error)"=w901, "Message Data"=w904, "Message"="Engine Start", "Message Queue"=w906) -> ("error out"=w910:errorcluster)  [unwired: 6 in, 1 out]
          }
        }
        n313 = case shown="True" w867 {
          tunnel: w868 -> [w885 w887]
          tunnel: [w885 w886] -> w866
          frame False {
          }
          frame True {
            # "Score állaptból ide áthelyezve\nScore állapot innentõl kezdve nem szükséges"
            n314 = Unbundle By Name(w887) -> ("Etalon number"=w889:u32)
            n315 = Decrement(x=w889) -> (x-1=w888:u32)
            n316 = Bundle By Name(cluster=w887, "Etalon number"=w888) -> (w886:T2)
          }
        }
        n317 = Replace Array Subset(array=w876, new element=w866, index=w875) -> (w877:T2[])
      }
      frame "ENGINE Jump" {
        w937 = T3 {"Thread ID"=0.0, "Mérésszám"="", "Mérés/Utasítás"="", "Command"={"Parancs"="", "Paraméter 1"="", "Paraméter 2"="", "Paraméter 3"="", "Paraméter 4"="", "Paraméter 5"="", "Eredmény"=""}, "Min"="", "Max"="", "Aktív?"=FALSE, "Log?"=FALSE, "Kiértékelés"=FALSE, "Etalon 1 exp"=FALSE, "Etalon 2 exp"=FALSE, "Etalon 3 exp"=FALSE, "Etalon 4 exp"=FALSE, "Etalon 5 exp"=FALSE}  # Teszt cluster
        w939 = T7 {"Thread ID"=0, "Callback"="", "Data"=variant, "Error"={"status"=FALSE, "code"=0, "source"=""}}  # Message
        n318 = Variant To Data(error in=w934, type=w939, Variant=w935) -> (data=w933:T7, error out=w936:errorcluster)
        n319 = Unbundle By Name(w933) -> ("Thread ID"=w921:u16)
        n320 = Unbundle By Name(w933) -> ("Data"=w938:variant)
        n321 = Index Array(array=w928, index=w921) -> (element=w929:T2)
        n322 = Variant To Data(error in=w936, type=w937, Variant=w938) -> (data=w931:T3, error out=w922:errorcluster)
        n323 = Unbundle By Name(w929) -> ("Program"=w932:T3[])
        n324 = Unbundle By Name(w931) -> ("Command.Paraméter 1"=w930:string)
        n325 = for {
          tunnel: w932 -> [w945] mode=indexing
          tunnel: w930 -> [w943]
          tunnel: [w941] -> w920
          i -> [w941]
          stop <- w942 stop-if-true
          n326 = Unbundle By Name(w945) -> ("Command.Parancs"=w944:string)
          n327 = Equal?(x=w944, y=w943) -> (x = y?=w942:bool)
        }
        n328 = Increment(x=w920) -> (x+1=w919:i32)
        n329 = Bundle By Name(cluster=w929, "Program PTR"=w919) -> (w926:T2)
        n330 = Replace Array Subset(array=w928, new element=w926, index=w921) -> (w927:T2[])
        n331 = call-poly "Enqueue Message.vi"("error in (no error)"=w922, "Message Data"=w921, "Message"="Select Test", "Message Queue"=w923) -> ("error out"=w924:errorcluster)  [unwired: 6 in, 1 out]
      }
      frame "ENGINE Etalon Meas?" {
        w962 = T3 {"Thread ID"=0.0, "Mérésszám"="", "Mérés/Utasítás"="", "Command"={"Parancs"="", "Paraméter 1"="", "Paraméter 2"="", "Paraméter 3"="", "Paraméter 4"="", "Paraméter 5"="", "Eredmény"=""}, "Min"="", "Max"="", "Aktív?"=FALSE, "Log?"=FALSE, "Kiértékelés"=FALSE, "Etalon 1 exp"=FALSE, "Etalon 2 exp"=FALSE, "Etalon 3 exp"=FALSE, "Etalon 4 exp"=FALSE, "Etalon 5 exp"=FALSE}  # Teszt cluster
        w964 = T7 {"Thread ID"=0, "Callback"="", "Data"=variant, "Error"={"status"=FALSE, "code"=0, "source"=""}}  # Message
        # "5 etalon lehet max"
        n332 = Variant To Data(error in=w959, type=w964, Variant=w960) -> (data=w958:T7, error out=w961:errorcluster)
        n333 = Unbundle By Name(w958) -> ("Thread ID"=w949:u16)
        n334 = Unbundle By Name(w958) -> ("Data"=w963:variant)
        n335 = Index Array(array=w956, index=w949) -> (element=w947:T2)
        n336 = Variant To Data(error in=w961, type=w962, Variant=w963) -> (data=w957:T3, error out=w950:errorcluster)
        n337 = Unbundle By Name(w947) -> ("Etalon number"=w946:u32)
        n338 = case shown="0, Default" w946 {
          tunnel: w957 -> [_ w975 w987 w999 w1011 w1023]
          tunnel: [w966 w973 w985 w997 w1009 w1021] -> w954
          tunnel: w947 -> [w968 w970 w982 w994 w1006 w1018]
          frame 0, Default {
            n339 = Unbundle By Name(w968) -> ("Program PTR"=w967:u32)
            n340 = Increment(x=w967) -> (x+1=w969:u32)
            n341 = Bundle By Name(cluster=w968, "Program PTR"=w969) -> (w966:T2)
          }
          frame 1 {
            n342 = Unbundle By Name(w970) -> ("Program"=w976:T3[])
            n343 = Unbundle By Name(w975) -> ("Command.Paraméter 1"=w974:string)
            n344 = for {
              tunnel: w976 -> [w981] mode=indexing
              tunnel: w974 -> [w979]
              tunnel: [w977] -> w972
              i -> [w977]
              stop <- w978 stop-if-true
              n345 = Unbundle By Name(w981) -> ("Command.Parancs"=w980:string)
              n346 = Equal?(x=w980, y=w979) -> (x = y?=w978:bool)
            }
            n347 = Increment(x=w972) -> (x+1=w971:i32)
            n348 = Bundle By Name(cluster=w970, "Program PTR"=w971) -> (w973:T2)
          }
          frame 2 {
            n349 = Unbundle By Name(w982) -> ("Program"=w988:T3[])
            n350 = Unbundle By Name(w987) -> ("Command.Paraméter 2"=w986:string)
            n351 = for {
              tunnel: w988 -> [w993] mode=indexing
              tunnel: w986 -> [w991]
              tunnel: [w989] -> w984
              i -> [w989]
              stop <- w990 stop-if-true
              n352 = Unbundle By Name(w993) -> ("Command.Parancs"=w992:string)
              n353 = Equal?(x=w992, y=w991) -> (x = y?=w990:bool)
            }
            n354 = Increment(x=w984) -> (x+1=w983:i32)
            n355 = Bundle By Name(cluster=w982, "Program PTR"=w983) -> (w985:T2)
          }
          frame 3 {
            n356 = Unbundle By Name(w994) -> ("Program"=w1000:T3[])
            n357 = Unbundle By Name(w999) -> ("Command.Paraméter 3"=w998:string)
            n358 = for {
              tunnel: w1000 -> [w1005] mode=indexing
              tunnel: w998 -> [w1003]
              tunnel: [w1001] -> w996
              i -> [w1001]
              stop <- w1002 stop-if-true
              n359 = Unbundle By Name(w1005) -> ("Command.Parancs"=w1004:string)
              n360 = Equal?(x=w1004, y=w1003) -> (x = y?=w1002:bool)
            }
            n361 = Increment(x=w996) -> (x+1=w995:i32)
            n362 = Bundle By Name(cluster=w994, "Program PTR"=w995) -> (w997:T2)
          }
          frame 4 {
            n363 = Unbundle By Name(w1006) -> ("Program"=w1012:T3[])
            n364 = Unbundle By Name(w1011) -> ("Command.Paraméter 4"=w1010:string)
            n365 = for {
              tunnel: w1012 -> [w1017] mode=indexing
              tunnel: w1010 -> [w1015]
              tunnel: [w1013] -> w1008
              i -> [w1013]
              stop <- w1014 stop-if-true
              n366 = Unbundle By Name(w1017) -> ("Command.Parancs"=w1016:string)
              n367 = Equal?(x=w1016, y=w1015) -> (x = y?=w1014:bool)
            }
            n368 = Increment(x=w1008) -> (x+1=w1007:i32)
            n369 = Bundle By Name(cluster=w1006, "Program PTR"=w1007) -> (w1009:T2)
          }
          frame 5 {
            n370 = Unbundle By Name(w1018) -> ("Program"=w1024:T3[])
            n371 = Unbundle By Name(w1023) -> ("Command.Paraméter 5"=w1022:string)
            n372 = for {
              tunnel: w1024 -> [w1029] mode=indexing
              tunnel: w1022 -> [w1027]
              tunnel: [w1025] -> w1020
              i -> [w1025]
              stop <- w1026 stop-if-true
              n373 = Unbundle By Name(w1029) -> ("Command.Parancs"=w1028:string)
              n374 = Equal?(x=w1028, y=w1027) -> (x = y?=w1026:bool)
            }
            n375 = Increment(x=w1020) -> (x+1=w1019:i32)
            n376 = Bundle By Name(cluster=w1018, "Program PTR"=w1019) -> (w1021:T2)
          }
        }
        n377 = Replace Array Subset(array=w956, new element=w954, index=w949) -> (w955:T2[])
        n378 = call-poly "Enqueue Message.vi"("error in (no error)"=w950, "Message Data"=w949, "Message"="Select Test", "Message Queue"=w951) -> ("error out"=w952:errorcluster)  [unwired: 6 in, 1 out]
      }
      frame "ENGINE Stop" {
        w1050 = T3 {"Thread ID"=0.0, "Mérésszám"="", "Mérés/Utasítás"="", "Command"={"Parancs"="", "Paraméter 1"="", "Paraméter 2"="", "Paraméter 3"="", "Paraméter 4"="", "Paraméter 5"="", "Eredmény"=""}, "Min"="", "Max"="", "Aktív?"=FALSE, "Log?"=FALSE, "Kiértékelés"=FALSE, "Etalon 1 exp"=FALSE, "Etalon 2 exp"=FALSE, "Etalon 3 exp"=FALSE, "Etalon 4 exp"=FALSE, "Etalon 5 exp"=FALSE}  # Teszt cluster
        w1052 = T7 {"Thread ID"=0, "Callback"="", "Data"=variant, "Error"={"status"=FALSE, "code"=0, "source"=""}}  # Message
        n379 = Variant To Data(error in=w1047, type=w1052, Variant=w1048) -> (data=w1034:T7, error out=w1049:errorcluster)
        n380 = Unbundle By Name(w1034) -> ("Data"=w1051:variant)
        n381 = Variant To Data(error in=w1049, type=w1050, Variant=w1051) -> (data=w1037:T3, error out=w1030:errorcluster)
        n382 = Unbundle By Name(w1034) -> ("Thread ID"=w1040:u16)
        n383 = Index Array(array=w1046, index=w1040) -> (element=w1042:T2)
        n384 = Bundle By Name(cluster=w1042, "Run"=FALSE) -> (w1044:T2)
        n385 = Bundle By Name(cluster=w1037, "Kiértékelés"=TRUE, "Command.Eredmény"="Program futás leállítva!") -> (w1033:T3)
        n386 = Bundle By Name(cluster=w1034, "Data"=w1033) -> (w1032:T7)
        n387 = Replace Array Subset(array=w1046, new element=w1044, index=w1040) -> (w1045:T2[])
        n388 = Unbundle By Name(w1032) -> ("Callback"=w1031:string)
        n389 = call-poly "Enqueue Message.vi"("error in (no error)"=w1030, "Message Data"=w1032, "Message"=w1031, "Message Queue"=w1038) -> ("error out"=w1039:errorcluster)  [unwired: 6 in, 1 out]
      }
      frame "ENGINE Start Thread" {
        w1076 = T3 {"Thread ID"=0.0, "Mérésszám"="", "Mérés/Utasítás"="", "Command"={"Parancs"="", "Paraméter 1"="", "Paraméter 2"="", "Paraméter 3"="", "Paraméter 4"="", "Paraméter 5"="", "Eredmény"=""}, "Min"="", "Max"="", "Aktív?"=FALSE, "Log?"=FALSE, "Kiértékelés"=FALSE, "Etalon 1 exp"=FALSE, "Etalon 2 exp"=FALSE, "Etalon 3 exp"=FALSE, "Etalon 4 exp"=FALSE, "Etalon 5 exp"=FALSE}  # Teszt cluster
        w1078 = T7 {"Thread ID"=0, "Callback"="", "Data"=variant, "Error"={"status"=FALSE, "code"=0, "source"=""}}  # Message
        n390 = Variant To Data(error in=w1073, type=w1078, Variant=w1074) -> (data=w1068:T7, error out=w1075:errorcluster)
        n391 = Unbundle By Name(w1068) -> ("Data"=w1077:variant)
        n392 = Variant To Data(error in=w1075, type=w1076, Variant=w1077) -> (data=w1064:T3, error out=w1060:errorcluster)
        n393 = Unbundle By Name(w1064) -> ("Command.Paraméter 1"=w1063:string)
        n394 = Decimal String To Number(string=w1063, default (0L)=u16 0 ("default (0 I32)")) -> (number=w1056:u16)  [unwired: 1 in, 1 out]
        n395 = Index Array(array=w1057, index=w1056) -> (element=w1055:T2)
        n396 = Unbundle By Name(w1055) -> ("Run"=w1054:bool)
        n397 = case shown="False" w1054 {
          tunnel: w1061 -> [w1084 w1086]
          tunnel: w1060 -> [w1083 w1087]
          tunnel: [w1082 w1086] -> w1059
          tunnel: [w1081 w1087] -> w1058
          tunnel: w1056 -> [w1080 _]
          frame False {
            n398 = call-poly "Enqueue Message.vi"("error in (no error)"=w1083, "Message Data"=w1080, "Message"="Engine Start", "Message Queue"=w1084) -> ("error out"=w1081:errorcluster, "dup Message Queue"=w1082:refnum<queue>)  [unwired: 6 in]
          }
          frame True {
          }
        }
        n399 = Bundle By Name(cluster=w1064, "Kiértékelés"=TRUE, "Command.Eredmény"="Párhuzamos szál elindítása") -> (w1067:T3)
        n400 = Bundle By Name(cluster=w1068, "Data"=w1067) -> (w1066:T7)
        n401 = Unbundle By Name(w1066) -> ("Callback"=w1065:string)
        n402 = call-poly "Enqueue Message.vi"("error in (no error)"=w1058, "Message Data"=w1066, "Message"=w1065, "Message Queue"=w1059) -> ("error out"=w1071:errorcluster)  [unwired: 6 in, 1 out]
      }
      frame "ENGINE Stop Thread" {
        w1110 = T3 {"Thread ID"=0.0, "Mérésszám"="", "Mérés/Utasítás"="", "Command"={"Parancs"="", "Paraméter 1"="", "Paraméter 2"="", "Paraméter 3"="", "Paraméter 4"="", "Paraméter 5"="", "Eredmény"=""}, "Min"="", "Max"="", "Aktív?"=FALSE, "Log?"=FALSE, "Kiértékelés"=FALSE, "Etalon 1 exp"=FALSE, "Etalon 2 exp"=FALSE, "Etalon 3 exp"=FALSE, "Etalon 4 exp"=FALSE, "Etalon 5 exp"=FALSE}  # Teszt cluster
        w1112 = T7 {"Thread ID"=0, "Callback"="", "Data"=variant, "Error"={"status"=FALSE, "code"=0, "source"=""}}  # Message
        n403 = Variant To Data(error in=w1107, type=w1112, Variant=w1108) -> (data=w1102:T7, error out=w1109:errorcluster)
        n404 = Unbundle By Name(w1102) -> ("Data"=w1111:variant)
        n405 = Variant To Data(error in=w1109, type=w1110, Variant=w1111) -> (data=w1098:T3, error out=w1094:errorcluster)
        n406 = Unbundle By Name(w1098) -> ("Command.Paraméter 1"=w1097:string)
        n407 = Decimal String To Number(string=w1097, default (0L)=u16 0 ("default (0 I32)")) -> (number=w1090:u16)  [unwired: 1 in, 1 out]
        n408 = Index Array(array=w1091, index=w1090) -> (element=w1089:T2)
        n409 = Unbundle By Name(w1089) -> ("Run"=w1088:bool)
        n410 = case shown="True" w1088 {
          tunnel: w1095 -> [w1114 w1122]
          tunnel: w1094 -> [w1115 w1121]
          tunnel: [w1114 w1120] -> w1093
          tunnel: [w1115 w1119] -> w1092
          tunnel: w1090 -> [_ w1117]
          frame False {
          }
          frame True {
            w1118 = T8 {"Thread ID"=0, "Thread Flag"=FALSE}  # Thread Flag
            n411 = Bundle By Name(cluster=w1118, "Thread ID"=w1117) -> (w1116:T8)
            n412 = call-poly "Enqueue Message.vi"("error in (no error)"=w1121, "Message Data"=w1116, "Message"="Abort", "Message Queue"=w1122) -> ("error out"=w1119:errorcluster, "dup Message Queue"=w1120:refnum<queue>)  [unwired: 6 in]
          }
        }
        n413 = Bundle By Name(cluster=w1098, "Kiértékelés"=TRUE, "Command.Eredmény"="Párhuzamos szál leállítása") -> (w1101:T3)
        n414 = Bundle By Name(cluster=w1102, "Data"=w1101) -> (w1100:T7)
        n415 = Unbundle By Name(w1100) -> ("Callback"=w1099:string)
        n416 = call-poly "Enqueue Message.vi"("error in (no error)"=w1092, "Message Data"=w1100, "Message"=w1099, "Message Queue"=w1093) -> ("error out"=w1105:errorcluster)  [unwired: 6 in, 1 out]
      }
      frame "ENGINE Send Command" {
        w1126 = ""
        w1147 = T3 {"Thread ID"=0.0, "Mérésszám"="", "Mérés/Utasítás"="", "Command"={"Parancs"="", "Paraméter 1"="", "Paraméter 2"="", "Paraméter 3"="", "Paraméter 4"="", "Paraméter 5"="", "Eredmény"=""}, "Min"="", "Max"="", "Aktív?"=FALSE, "Log?"=FALSE, "Kiértékelés"=FALSE, "Etalon 1 exp"=FALSE, "Etalon 2 exp"=FALSE, "Etalon 3 exp"=FALSE, "Etalon 4 exp"=FALSE, "Etalon 5 exp"=FALSE}  # Teszt cluster
        w1149 = T7 {"Thread ID"=0, "Callback"="", "Data"=variant, "Error"={"status"=FALSE, "code"=0, "source"=""}}  # Message
        # "Command"
        # "Thread ID"
        n417 = Variant To Data(error in=w1144, type=w1149, Variant=w1145) -> (data=w1138:T7, error out=w1146:errorcluster)
        n418 = Unbundle By Name(w1138) -> ("Data"=w1148:variant)
        n419 = Variant To Data(error in=w1146, type=w1147, Variant=w1148) -> (data=w1137:T3, error out=w1135:errorcluster)
        n420 = Unbundle By Name(w1137) -> ("Command.Paraméter 1"=w1141:string)
        n421 = Unbundle By Name(w1137) -> ("Command.Paraméter 2"=w1128:string)
        n422 = Decimal String To Number(string=w1141, default (0L)=u16 0 ("default (0 I32)")) -> (number=w1133:u16)  [unwired: 1 in, 1 out]
        n423 = Index Array(array=w1131, index=w1133) -> (element=w1130:T2)
        n424 = Unbundle By Name(w1130) -> ("Command"=w1132:string, "Response"=w1124:string)
        n425 = Equal?(x=w1132, y=w1126) -> (x = y?=w1127:bool)
        n426 = Equal?(x=w1124, y=w1126) -> (x = y?=w1125:bool)
        n427 = case shown="True" w1127 {
          tunnel: [w1160 w1195] -> w1142
          tunnel: w1138 -> [w1159 w1189]
          tunnel: w1137 -> [w1158 _]
          tunnel: w1136 -> [w1157 w1194]
          tunnel: w1135 -> [w1156 w1193]
          tunnel: w1132 -> [w1151 w1190]
          tunnel: w1130 -> [w1155 w1192]
          tunnel: [w1154 w1191] -> w1129
          tunnel: w1128 -> [w1153 _]
          tunnel: w1125 -> [w1152 _]
          tunnel: w1124 -> [w1150 _]
          frame True {
            # "Elõzõ parancs lefutott"
            n428 = case shown="True" w1152 {
              tunnel: [w1173 w1186] -> w1160
              tunnel: w1159 -> [w1168 w1181]
              tunnel: w1158 -> [w1167 w1180]
              tunnel: w1157 -> [w1166 w1179]
              tunnel: w1156 -> [w1165 w1178]
              tunnel: w1155 -> [w1163 w1177]
              tunnel: [w1162 w1176] -> w1154
              tunnel: w1153 -> [w1161 _]
              tunnel: w1151 -> [_ w1175]
              tunnel: w1150 -> [_ w1174]
              frame True {
                # "Nem volt hiba ->új parancs küldése"
                n429 = Bundle By Name(cluster=w1163, "Command"=w1161) -> (w1162:T2)
                n430 = Bundle By Name(cluster=w1167, "Kiértékelés"=TRUE, "Command.Eredmény"="Command Sent") -> (w1171:T3)
                n431 = Bundle By Name(cluster=w1168, "Data"=w1171) -> (w1170:T7)
                n432 = Unbundle By Name(w1170) -> ("Callback"=w1169:string)
                n433 = call-poly "Enqueue Message.vi"("error in (no error)"=w1165, "Message Data"=w1170, "Message"=w1169, "Message Queue"=w1166) -> ("error out"=w1173:errorcluster)  [unwired: 6 in, 1 out]
              }
              frame False {
                # "Hiba volt -> nem küldhetõ új parancs"
                n434 = Bundle By Name(cluster=w1177, "Command"=w1175) -> (w1176:T2)
                n435 = Bundle By Name(cluster=w1180, "Kiértékelés"=FALSE, "Command.Eredmény"=w1174) -> (w1184:T3)
                n436 = Bundle By Name(cluster=w1181, "Data"=w1184) -> (w1183:T7)
                n437 = Unbundle By Name(w1183) -> ("Callback"=w1182:string)
                n438 = call-poly "Enqueue Message.vi"("error in (no error)"=w1178, "Message Data"=w1183, "Message"=w1182, "Message Queue"=w1179) -> ("error out"=w1186:errorcluster)  [unwired: 6 in, 1 out]
              }
            }
          }
          frame False {
            # "Elõzõ parancs nem futott le"
            n439 = Bundle By Name(cluster=w1192, "Command"=w1190) -> (w1191:T2)
            n440 = Wait (ms)(milliseconds to wait=u32 10) -> ()  [unwired: 1 out]
            n441 = call-poly "Enqueue Message.vi"("error in (no error)"=w1193, "Message Data"=w1189, "Message"="ENGINE Send Command", "Message Queue"=w1194) -> ("error out"=w1195:errorcluster)  [unwired: 6 in, 1 out]
          }
        }
        n442 = Replace Array Subset(array=w1131, new element=w1129, index=w1133) -> (w1134:T2[])
      }
      frame "ENGINE Wait Command Execution" {
        w1199 = ""
        w1216 = T3 {"Thread ID"=0.0, "Mérésszám"="", "Mérés/Utasítás"="", "Command"={"Parancs"="", "Paraméter 1"="", "Paraméter 2"="", "Paraméter 3"="", "Paraméter 4"="", "Paraméter 5"="", "Eredmény"=""}, "Min"="", "Max"="", "Aktív?"=FALSE, "Log?"=FALSE, "Kiértékelés"=FALSE, "Etalon 1 exp"=FALSE, "Etalon 2 exp"=FALSE, "Etalon 3 exp"=FALSE, "Etalon 4 exp"=FALSE, "Etalon 5 exp"=FALSE}  # Teszt cluster
        w1218 = T7 {"Thread ID"=0, "Callback"="", "Data"=variant, "Error"={"status"=FALSE, "code"=0, "source"=""}}  # Message
        # "Thread ID"
        n443 = Variant To Data(error in=w1213, type=w1218, Variant=w1214) -> (data=w1207:T7, error out=w1215:errorcluster)
        n444 = Unbundle By Name(w1207) -> ("Data"=w1217:variant)
        n445 = Variant To Data(error in=w1215, type=w1216, Variant=w1217) -> (data=w1206:T3, error out=w1204:errorcluster)
        n446 = Unbundle By Name(w1206) -> ("Command.Paraméter 1"=w1210:string)
        n447 = Decimal String To Number(string=w1210, default (0L)=u16 0 ("default (0 I32)")) -> (number=w1203:u16)  [unwired: 1 in, 1 out]
        n448 = Index Array(array=w1196, index=w1203) -> (element=w1201:T2)
        n449 = Unbundle By Name(w1201) -> ("Command"=w1202:string, "Response"=w1197:string)
        n450 = Equal?(x=w1202, y=w1199) -> (x = y?=w1200:bool)
        n451 = Equal?(x=w1197, y=w1199) -> (x = y?=w1198:bool)
        n452 = case shown="True" w1200 {
          tunnel: [w1225 w1251] -> w1211
          tunnel: w1207 -> [w1224 w1248]
          tunnel: w1206 -> [w1223 _]
          tunnel: w1205 -> [w1222 w1250]
          tunnel: w1204 -> [w1221 w1249]
          tunnel: w1198 -> [w1220 _]
          tunnel: w1197 -> [w1219 _]
          frame True {
            # "Elõzõ parancs lefutott"
            n453 = case shown="True" w1220 {
              tunnel: [w1235 w1245] -> w1225
              tunnel: w1224 -> [w1230 w1240]
              tunnel: w1223 -> [w1229 w1239]
              tunnel: w1222 -> [w1228 w1238]
              tunnel: w1221 -> [w1227 w1237]
              tunnel: w1219 -> [_ w1236]
              frame True {
                # "Nem volt hiba"
                n454 = Bundle By Name(cluster=w1229, "Kiértékelés"=TRUE, "Command.Eredmény"="Command Exetuted") -> (w1233:T3)
                n455 = Bundle By Name(cluster=w1230, "Data"=w1233) -> (w1232:T7)
                n456 = Unbundle By Name(w1232) -> ("Callback"=w1231:string)
                n457 = call-poly "Enqueue Message.vi"("error in (no error)"=w1227, "Message Data"=w1232, "Message"=w1231, "Message Queue"=w1228) -> ("error out"=w1235:errorcluster)  [unwired: 6 in, 1 out]
              }
              frame False {
                # "Hiba volt"
                n458 = Bundle By Name(cluster=w1239, "Kiértékelés"=FALSE, "Command.Eredmény"=w1236) -> (w1243:T3)
                n459 = Bundle By Name(cluster=w1240, "Data"=w1243) -> (w1242:T7)
                n460 = Unbundle By Name(w1242) -> ("Callback"=w1241:string)
                n461 = call-poly "Enqueue Message.vi"("error in (no error)"=w1237, "Message Data"=w1242, "Message"=w1241, "Message Queue"=w1238) -> ("error out"=w1245:errorcluster)  [unwired: 6 in, 1 out]
              }
            }
          }
          frame False {
            # "Vátakozás lefutásra"
            n462 = Wait (ms)(milliseconds to wait=u32 10) -> ()  [unwired: 1 out]
            n463 = call-poly "Enqueue Message.vi"("error in (no error)"=w1249, "Message Data"=w1248, "Message"="ENGINE Wait Command Execution", "Message Queue"=w1250) -> ("error out"=w1251:errorcluster)  [unwired: 6 in, 1 out]
          }
        }
      }
      frame "ENGINE Wait Command" {
        w1268 = T3 {"Thread ID"=0.0, "Mérésszám"="", "Mérés/Utasítás"="", "Command"={"Parancs"="", "Paraméter 1"="", "Paraméter 2"="", "Paraméter 3"="", "Paraméter 4"="", "Paraméter 5"="", "Eredmény"=""}, "Min"="", "Max"="", "Aktív?"=FALSE, "Log?"=FALSE, "Kiértékelés"=FALSE, "Etalon 1 exp"=FALSE, "Etalon 2 exp"=FALSE, "Etalon 3 exp"=FALSE, "Etalon 4 exp"=FALSE, "Etalon 5 exp"=FALSE}  # Teszt cluster
        w1270 = T7 {"Thread ID"=0, "Callback"="", "Data"=variant, "Error"={"status"=FALSE, "code"=0, "source"=""}}  # Message
        n464 = Variant To Data(error in=w1265, type=w1270, Variant=w1266) -> (data=w1260:T7, error out=w1267:errorcluster)
        n465 = Unbundle By Name(w1260) -> ("Data"=w1269:variant)
        n466 = Unbundle By Name(w1260) -> ("Thread ID"=w1259:u16)
        n467 = Variant To Data(error in=w1267, type=w1268, Variant=w1269) -> (data=w1262:T3, error out=w1254:errorcluster)
        n468 = Index Array(array=w1256, index=w1259) -> (element=w1258:T2)
        n469 = Unbundle By Name(w1258) -> ("Command"=w1252:string)
        n470 = Not Equal?(x=w1252, y="") -> (x != y?=w1253:bool)
        n471 = case shown="False" w1253 {
          tunnel: [w1279 w1285] -> w1263
          tunnel: w1262 -> [w1276 _]
          tunnel: w1260 -> [w1275 w1282]
          tunnel: w1255 -> [w1273 w1284]
          tunnel: w1254 -> [w1272 w1283]
          tunnel: w1252 -> [w1271 _]
          frame True {
            w1274 = "Engine Jump" ("Message")
            n472 = Bundle By Name(cluster=w1276, "Command.Parancs"=w1274, "Command.Paraméter 1"=w1271) -> (w1278:T3)
            n473 = Bundle By Name(cluster=w1275, "Data"=w1278) -> (w1277:T7)
            n474 = call-poly "Enqueue Message.vi"("error in (no error)"=w1272, "Message Data"=w1277, "Message"=w1274, "Message Queue"=w1273) -> ("error out"=w1279:errorcluster)  [unwired: 6 in, 1 out]
          }
          frame False {
            n475 = Wait (ms)(milliseconds to wait=u32 10) -> ()  [unwired: 1 out]
            n476 = call-poly "Enqueue Message.vi"("error in (no error)"=w1283, "Message Data"=w1282, "Message"="ENGINE Wait Command", "Message Queue"=w1284) -> ("error out"=w1285:errorcluster)  [unwired: 6 in, 1 out]
          }
        }
      }
      frame "ENGINE Send Response" {
        w1308 = T3 {"Thread ID"=0.0, "Mérésszám"="", "Mérés/Utasítás"="", "Command"={"Parancs"="", "Paraméter 1"="", "Paraméter 2"="", "Paraméter 3"="", "Paraméter 4"="", "Paraméter 5"="", "Eredmény"=""}, "Min"="", "Max"="", "Aktív?"=FALSE, "Log?"=FALSE, "Kiértékelés"=FALSE, "Etalon 1 exp"=FALSE, "Etalon 2 exp"=FALSE, "Etalon 3 exp"=FALSE, "Etalon 4 exp"=FALSE, "Etalon 5 exp"=FALSE}  # Teszt cluster
        w1310 = T7 {"Thread ID"=0, "Callback"="", "Data"=variant, "Error"={"status"=FALSE, "code"=0, "source"=""}}  # Message
        # "OK / ERROR"
        n477 = Variant To Data(error in=w1305, type=w1310, Variant=w1306) -> (data=w1290:T7, error out=w1307:errorcluster)
        n478 = Unbundle By Name(w1290) -> ("Data"=w1309:variant)
        n479 = Unbundle By Name(w1290) -> ("Thread ID"=w1300:u16)
        n480 = Variant To Data(error in=w1307, type=w1308, Variant=w1309) -> (data=w1289:T3, error out=w1291:errorcluster)
        n481 = Unbundle By Name(w1289) -> ("Command.Paraméter 1"=w1296:string)
        n482 = Index Array(array=w1301, index=w1300) -> (element=w1299:T2)
        n483 = Bundle By Name(cluster=w1299, "Command"="", "Response"=w1296) -> (w1298:T2)
        n484 = Bundle By Name(cluster=w1289, "Kiértékelés"=TRUE, "Command.Eredmény"="Response Sent") -> (w1294:T3)
        n485 = Replace Array Subset(array=w1301, new element=w1298, index=w1300) -> (w1302:T2[])
        n486 = Bundle By Name(cluster=w1290, "Data"=w1294) -> (w1293:T7)
        n487 = Unbundle By Name(w1293) -> ("Callback"=w1288:string)
        n488 = call-poly "Enqueue Message.vi"("error in (no error)"=w1291, "Message Data"=w1293, "Message"=w1288, "Message Queue"=w1287) -> ("error out"=w1292:errorcluster)  [unwired: 6 in, 1 out]
      }
      frame "ENGINE Score" {
        w1339 = T3 {"Thread ID"=0.0, "Mérésszám"="", "Mérés/Utasítás"="", "Command"={"Parancs"="", "Paraméter 1"="", "Paraméter 2"="", "Paraméter 3"="", "Paraméter 4"="", "Paraméter 5"="", "Eredmény"=""}, "Min"="", "Max"="", "Aktív?"=FALSE, "Log?"=FALSE, "Kiértékelés"=FALSE, "Etalon 1 exp"=FALSE, "Etalon 2 exp"=FALSE, "Etalon 3 exp"=FALSE, "Etalon 4 exp"=FALSE, "Etalon 5 exp"=FALSE}  # Teszt cluster
        w1341 = T7 {"Thread ID"=0, "Callback"="", "Data"=variant, "Error"={"status"=FALSE, "code"=0, "source"=""}}  # Message
        n489 = Variant To Data(error in=w1336, type=w1341, Variant=w1337) -> (data=w1312:T7, error out=w1338:errorcluster)
        n490 = Unbundle By Name(w1312) -> ("Data"=w1340:variant)
        n491 = Unbundle By Name(w1312) -> ("Thread ID"=w1334:u16)
        n492 = Index Array(array=w1328, index=w1334) -> (element=w1327:T2)
        n493 = Variant To Data(error in=w1338, type=w1339, Variant=w1340) -> (data=w1314:T3, error out=w1325:errorcluster)
        n494 = Unbundle By Name(w1327) -> ("Etalon number"=w1319:u32, "Meas Result"=w1321:bool)
        n495 = Greater Than 0?(x=w1319) -> (x > 0?=w1316:bool)
        n496 = case shown="False" w1316 {
          tunnel: w1326 -> [w1353 w1364]
          tunnel: w1312 -> [w1350 w1361]
          tunnel: w1325 -> [w1348 w1359]
          tunnel: [w1347 w1358] -> w1324
          tunnel: w1321 -> [w1345 w1356]
          tunnel: w1318 -> [w1346 w1357]
          tunnel: [w1346 w1357] -> w1317
          tunnel: [w1345 w1356] -> w1315
          tunnel: w1314 -> [w1344 w1355]
          tunnel: [w1344 w1355] -> w1313
          tunnel: w1312 -> [w1343 w1354]
          tunnel: [w1343 w1354] -> w1311
          frame False {
            # "TERMÉK MÉRÉS"
            n497 = Unbundle By Name(w1353) -> ("UI"=w1352:refnum<queue>)
            n498 = Bundle By Name(cluster=w1350, "Data"=w1345) -> (w1349:T7)
            n499 = call-poly "Enqueue Message.vi"("error in (no error)"=w1348, "Message Data"=w1349, "Message"="Kiértékelés UI", "Message Queue"=w1352) -> ("error out"=w1347:errorcluster)  [unwired: 6 in, 1 out]
          }
          frame True {
            # "ETALON MÉRÉS"
            n500 = Unbundle By Name(w1364) -> ("UI"=w1363:refnum<queue>)
            n501 = Bundle By Name(cluster=w1361, "Data"=w1356) -> (w1360:T7)
            n502 = call-poly "Enqueue Message.vi"("error in (no error)"=w1359, "Message Data"=w1360, "Message"="Kiértékelés Etalon UI", "Message Queue"=w1363) -> ("error out"=w1358:errorcluster)  [unwired: 6 in, 1 out]
          }
        }
        n503 = Select(t="OK" ("Command.Eredmény"), s=w1315, f="NOK" ("Command.Eredmény")) -> (s? t:f=w1320:string)
        n504 = Bundle By Name(cluster=w1313, "Kiértékelés"=TRUE, "Command.Eredmény"=w1320) -> (w1331:T3)
        n505 = Bundle By Name(cluster=w1311, "Data"=w1331) -> (w1330:T7)
        n506 = Unbundle By Name(w1330) -> ("Callback"=w1329:string)
        n507 = call-poly "Enqueue Message.vi"("error in (no error)"=w1324, "Message Data"=w1330, "Message"=w1329, "Message Queue"=w1317) -> ("error out"=w1333:errorcluster)  [unwired: 6 in, 1 out]
      }
      frame "ENGINE Write logfile" {
        w1388 = T3 {"Thread ID"=0.0, "Mérésszám"="", "Mérés/Utasítás"="", "Command"={"Parancs"="", "Paraméter 1"="", "Paraméter 2"="", "Paraméter 3"="", "Paraméter 4"="", "Paraméter 5"="", "Eredmény"=""}, "Min"="", "Max"="", "Aktív?"=FALSE, "Log?"=FALSE, "Kiértékelés"=FALSE, "Etalon 1 exp"=FALSE, "Etalon 2 exp"=FALSE, "Etalon 3 exp"=FALSE, "Etalon 4 exp"=FALSE, "Etalon 5 exp"=FALSE}  # Teszt cluster
        w1390 = T7 {"Thread ID"=0, "Callback"="", "Data"=variant, "Error"={"status"=FALSE, "code"=0, "source"=""}}  # Message
        n508 = Variant To Data(error in=w1385, type=w1390, Variant=w1386) -> (data=w1370:T7, error out=w1387:errorcluster)
        n509 = Unbundle By Name(w1370) -> ("Data"=w1389:variant)
        n510 = Variant To Data(error in=w1387, type=w1388, Variant=w1389) -> (data=w1380:T3, error out=w1368:errorcluster)
        n511 = Unbundle By Name(w1370) -> ("Thread ID"=w1383:u16)
        n512 = Index Array(array=w1375, index=w1383) -> (element=w1374:T2)
        n513 = Unbundle By Name(w1374) -> ("Etalon number"=w1366:u32)
        n514 = Unbundle By Name(w1373) -> ("UI"=w1372:refnum<queue>)
        n515 = Bundle By Name(cluster=w1370, "Data"=w1366) -> (w1369:T7)
        n516 = call-poly "Enqueue Message.vi"("error in (no error)"=w1368, "Message Data"=w1369, "Message"="Write logfile", "Message Queue"=w1372) -> ("error out"=w1367:errorcluster)  [unwired: 6 in, 1 out]
        n517 = Bundle By Name(cluster=w1380, "Kiértékelés"=TRUE, "Command.Eredmény"="") -> (w1378:T3)
        n518 = Bundle By Name(cluster=w1370, "Data"=w1378) -> (w1377:T7)
        n519 = Unbundle By Name(w1377) -> ("Callback"=w1376:string)
        n520 = call-poly "Enqueue Message.vi"("error in (no error)"=w1367, "Message Data"=w1377, "Message"=w1376, "Message Queue"=w1381) -> ("error out"=w1382:errorcluster)  [unwired: 6 in, 1 out]
      }
      frame "ENGINE Base Position" {
        w1413 = T3 {"Thread ID"=0.0, "Mérésszám"="", "Mérés/Utasítás"="", "Command"={"Parancs"="", "Paraméter 1"="", "Paraméter 2"="", "Paraméter 3"="", "Paraméter 4"="", "Paraméter 5"="", "Eredmény"=""}, "Min"="", "Max"="", "Aktív?"=FALSE, "Log?"=FALSE, "Kiértékelés"=FALSE, "Etalon 1 exp"=FALSE, "Etalon 2 exp"=FALSE, "Etalon 3 exp"=FALSE, "Etalon 4 exp"=FALSE, "Etalon 5 exp"=FALSE}  # Teszt cluster
        w1415 = T7 {"Thread ID"=0, "Callback"="", "Data"=variant, "Error"={"status"=FALSE, "code"=0, "source"=""}}  # Message
        n521 = Variant To Data(error in=w1410, type=w1415, Variant=w1411) -> (data=w1400:T7, error out=w1412:errorcluster)
        n522 = Unbundle By Name(w1400) -> ("Data"=w1414:variant)
        n523 = Variant To Data(error in=w1412, type=w1413, Variant=w1414) -> (data=w1395:T3, error out=w1396:errorcluster)
        n524 = Unbundle By Name(w1400) -> ("Thread ID"=w1404:u16)
        n525 = Unbundle By Name(w1395) -> ("Command.Paraméter 1"=w1394:string)
        n526 = Index Array(array=w1409, index=w1404) -> (element=w1405:T2)
        n527 = case shown="\"1\", Default" w1394 {
          tunnel: [TRUE ("Run") FALSE ("Run")] -> w1393
          frame "1", Default {
          }
          frame "0" {
          }
        }
        n528 = Bundle By Name(cluster=w1405, "Alaphelyzet"=w1393) -> (w1407:T2)
        n529 = Bundle By Name(cluster=w1395, "Kiértékelés"=TRUE, "Command.Eredmény"="") -> (w1399:T3)
        n530 = Bundle By Name(cluster=w1400, "Data"=w1399) -> (w1398:T7)
        n531 = Replace Array Subset(array=w1409, new element=w1407, index=w1404) -> (w1408:T2[])
        n532 = Unbundle By Name(w1398) -> ("Callback"=w1397:string)
        n533 = call-poly "Enqueue Message.vi"("error in (no error)"=w1396, "Message Data"=w1398, "Message"=w1397, "Message Queue"=w1402) -> ("error out"=w1403:errorcluster)  [unwired: 6 in, 1 out]
      }
      frame "ENGINE Check Base Position" {
        w1438 = T3 {"Thread ID"=0.0, "Mérésszám"="", "Mérés/Utasítás"="", "Command"={"Parancs"="", "Paraméter 1"="", "Paraméter 2"="", "Paraméter 3"="", "Paraméter 4"="", "Paraméter 5"="", "Eredmény"=""}, "Min"="", "Max"="", "Aktív?"=FALSE, "Log?"=FALSE, "Kiértékelés"=FALSE, "Etalon 1 exp"=FALSE, "Etalon 2 exp"=FALSE, "Etalon 3 exp"=FALSE, "Etalon 4 exp"=FALSE, "Etalon 5 exp"=FALSE}  # Teszt cluster
        w1440 = T7 {"Thread ID"=0, "Callback"="", "Data"=variant, "Error"={"status"=FALSE, "code"=0, "source"=""}}  # Message
        n534 = Variant To Data(error in=w1435, type=w1440, Variant=w1436) -> (data=w1430:T7, error out=w1437:errorcluster)
        n535 = Unbundle By Name(w1430) -> ("Data"=w1439:variant)
        n536 = Variant To Data(error in=w1437, type=w1438, Variant=w1439) -> (data=w1425:T3, error out=w1426:errorcluster)
        n537 = Unbundle By Name(w1430) -> ("Thread ID"=w1433:u16)
        n538 = Index Array(array=w1424, index=w1433) -> (element=w1423:T2)
        n539 = Unbundle By Name(w1423) -> ("Alaphelyzet"=w1422:bool)
        n540 = Select(t="Alaphelyzetben", s=w1422, f="Nincs Alaphelyzetben") -> (s? t:f=w1421:string)
        n541 = Bundle By Name(cluster=w1425, "Kiértékelés"=w1422, "Command.Eredmény"=w1421) -> (w1429:T3)
        n542 = Bundle By Name(cluster=w1430, "Data"=w1429) -> (w1428:T7)
        n543 = Unbundle By Name(w1428) -> ("Callback"=w1427:string)
        n544 = call-poly "Enqueue Message.vi"("error in (no error)"=w1426, "Message Data"=w1428, "Message"=w1427, "Message Queue"=w1431) -> ("error out"=w1432:errorcluster)  [unwired: 6 in, 1 out]
      }
      frame "ENGINE Check Meas Result" {
        w1461 = T3 {"Thread ID"=0.0, "Mérésszám"="", "Mérés/Utasítás"="", "Command"={"Parancs"="", "Paraméter 1"="", "Paraméter 2"="", "Paraméter 3"="", "Paraméter 4"="", "Paraméter 5"="", "Eredmény"=""}, "Min"="", "Max"="", "Aktív?"=FALSE, "Log?"=FALSE, "Kiértékelés"=FALSE, "Etalon 1 exp"=FALSE, "Etalon 2 exp"=FALSE, "Etalon 3 exp"=FALSE, "Etalon 4 exp"=FALSE, "Etalon 5 exp"=FALSE}  # Teszt cluster
        w1463 = T7 {"Thread ID"=0, "Callback"="", "Data"=variant, "Error"={"status"=FALSE, "code"=0, "source"=""}}  # Message
        n545 = Variant To Data(error in=w1458, type=w1463, Variant=w1459) -> (data=w1453:T7, error out=w1460:errorcluster)
        n546 = Unbundle By Name(w1453) -> ("Data"=w1462:variant)
        n547 = Variant To Data(error in=w1460, type=w1461, Variant=w1462) -> (data=w1446:T3, error out=w1452:errorcluster)
        n548 = Unbundle By Name(w1453) -> ("Thread ID"=w1456:u16)
        n549 = Unbundle By Name(w1446) -> ("Command.Paraméter 1"=w1445:string)
        n550 = Index Array(array=w1451, index=w1456) -> (element=w1450:T2)
        n551 = Unbundle By Name(w1450) -> ("Meas Result"=w1449:bool, "Etalon Result"=w1447:bool, "Etalon number"=w1448:u32, "Ignore Error"=w1443:bool)
        n552 = case shown="\"Enable Ignore Error Mode\", Default" w1445 {
          tunnel: [TRUE ("Run") FALSE ("Run")] -> w1444
          frame "Enable Ignore Error Mode", Default {
          }
          frame "Disable Ignore Error Mode" {
          }
        }
        n553 = And(x=w1443, y=w1444) -> (x .and. y?=w1442:bool)
        n554 = case shown="True" w1442 {
          tunnel: [w1474 w1506] -> w1455
          tunnel: w1454 -> [w1473 w1505]
          tunnel: w1453 -> [w1472 w1504]
          tunnel: w1452 -> [w1471 w1503]
          tunnel: w1446 -> [w1470 w1502]
          tunnel: w1449 -> [w1467 w1501]
          tunnel: w1448 -> [w1469 w1500]
          tunnel: w1447 -> [w1468 w1499]
          frame False {
            # "Ez az ág nem veszi figyelembe a végigmérés funkciót"
            n555 = case shown="0, Default" w1469 {
              tunnel: [w1486 w1498] -> w1474
              tunnel: w1473 -> [w1485 w1497]
              tunnel: w1472 -> [w1484 w1496]
              tunnel: w1471 -> [w1480 w1492]
              tunnel: w1470 -> [w1479 w1491]
              tunnel: w1467 -> [_ w1487]
              tunnel: w1468 -> [w1475 _]
              frame 1..5 {
                n556 = Select(t="ETALON OK", s=w1475, f="ETALON NOK") -> (s? t:f=w1478:string)
                n557 = Bundle By Name(cluster=w1479, "Kiértékelés"=w1475, "Command.Eredmény"=w1478) -> (w1483:T3)
                n558 = Bundle By Name(cluster=w1484, "Data"=w1483) -> (w1482:T7)
                n559 = Unbundle By Name(w1482) -> ("Callback"=w1481:string)
                n560 = call-poly "Enqueue Message.vi"("error in (no error)"=w1480, "Message Data"=w1482, "Message"=w1481, "Message Queue"=w1485) -> ("error out"=w1486:errorcluster)  [unwired: 6 in, 1 out]
              }
              frame 0, Default {
                n561 = Select(t="Mérés OK", s=w1487, f="Mérés NOK") -> (s? t:f=w1490:string)
                n562 = Bundle By Name(cluster=w1491, "Kiértékelés"=w1487, "Command.Eredmény"=w1490) -> (w1495:T3)
                n563 = Bundle By Name(cluster=w1496, "Data"=w1495) -> (w1494:T7)
                n564 = Unbundle By Name(w1494) -> ("Callback"=w1493:string)
                n565 = call-poly "Enqueue Message.vi"("error in (no error)"=w1492, "Message Data"=w1494, "Message"=w1493, "Message Queue"=w1497) -> ("error out"=w1498:errorcluster)  [unwired: 6 in, 1 out]
              }
            }
          }
          frame True {
            # "Ez az ág reagál a végigmérés funkcióra"
            n566 = case shown="0, Default" w1500 {
              tunnel: [w1519 w1532] -> w1506
              tunnel: w1505 -> [w1518 w1531]
              tunnel: w1504 -> [w1517 w1530]
              tunnel: w1503 -> [w1513 w1526]
              tunnel: w1502 -> [w1512 w1525]
              tunnel: w1501 -> [_ w1520]
              tunnel: w1499 -> [w1508 _]
              frame 1..5 {
                n567 = Select(t="ETALON OK", s=w1508, f="ETALON NOK") -> (s? t:f=w1511:string)
                n568 = Bundle By Name(cluster=w1512, "Kiértékelés"=TRUE, "Command.Eredmény"=w1511) -> (w1516:T3)
                n569 = Bundle By Name(cluster=w1517, "Data"=w1516) -> (w1515:T7)
                n570 = Unbundle By Name(w1515) -> ("Callback"=w1514:string)
                n571 = call-poly "Enqueue Message.vi"("error in (no error)"=w1513, "Message Data"=w1515, "Message"=w1514, "Message Queue"=w1518) -> ("error out"=w1519:errorcluster)  [unwired: 6 in, 1 out]
              }
              frame 0, Default {
                n572 = Select(t="Mérés OK", s=w1520, f="Mérés NOK") -> (s? t:f=w1524:string)
                n573 = Bundle By Name(cluster=w1525, "Kiértékelés"=TRUE, "Command.Eredmény"=w1524) -> (w1529:T3)
                n574 = Bundle By Name(cluster=w1530, "Data"=w1529) -> (w1528:T7)
                n575 = Unbundle By Name(w1528) -> ("Callback"=w1527:string)
                n576 = call-poly "Enqueue Message.vi"("error in (no error)"=w1526, "Message Data"=w1528, "Message"=w1527, "Message Queue"=w1531) -> ("error out"=w1532:errorcluster)  [unwired: 6 in, 1 out]
              }
            }
          }
        }
      }
      frame "ENGINE Store Data" {
        w1554 = T3 {"Thread ID"=0.0, "Mérésszám"="", "Mérés/Utasítás"="", "Command"={"Parancs"="", "Paraméter 1"="", "Paraméter 2"="", "Paraméter 3"="", "Paraméter 4"="", "Paraméter 5"="", "Eredmény"=""}, "Min"="", "Max"="", "Aktív?"=FALSE, "Log?"=FALSE, "Kiértékelés"=FALSE, "Etalon 1 exp"=FALSE, "Etalon 2 exp"=FALSE, "Etalon 3 exp"=FALSE, "Etalon 4 exp"=FALSE, "Etalon 5 exp"=FALSE}  # Teszt cluster
        w1556 = T7 {"Thread ID"=0, "Callback"="", "Data"=variant, "Error"={"status"=FALSE, "code"=0, "source"=""}}  # Message
        n577 = Variant To Data(error in=w1551, type=w1556, Variant=w1552) -> (data=w1541:T7, error out=w1553:errorcluster)
        n578 = Unbundle By Name(w1541) -> ("Thread ID"=w1548:u16)
        n579 = Unbundle By Name(w1541) -> ("Data"=w1555:variant)
        n580 = Index Array(array=w1549, index=w1548) -> (element=w1547:T2)
        n581 = Variant To Data(error in=w1553, type=w1554, Variant=w1555) -> (data=w1542:T3, error out=w1546:errorcluster)
        n582 = Unbundle By Name(w1547) -> ("Previous Test.Command.Eredmény"=w1535:string)
        n583 = Unbundle By Name(w1542) -> ("Command.Paraméter 1"=w1550:string)
        n584 = case shown="1" w1548 {
          tunnel: w1550 -> [w1564 w1572]
          tunnel: w1535 -> [w1561 w1569]
          tunnel: w1546 -> [w1563 w1571]
          tunnel: [w1563 w1571] -> w1536
          tunnel: w1538 -> [w1562 w1570]
          tunnel: [w1562 w1570] -> w1537
          tunnel: [w1560 w1567] -> w1534
          frame 0, Default {
            n585 = Decimal String To Number(string=w1564) -> (number=w1558:i32)  [unwired: 2 in, 1 out]
            n586 = global read "Global 1.vi" "Data Buffer 1"() -> (w1565:string[])
            n587 = Replace Array Subset(array=w1565, new element=w1561, index=w1558) -> (w1559:string[])
            n588 = global write "Global 1.vi" "Data Buffer 1"(w1559) -> ()
            n589 = Index Array(array=w1559, index=w1558) -> (element=w1560:string)
          }
          frame 1 {
            n590 = Decimal String To Number(string=w1572) -> (number=w1566:i32)  [unwired: 2 in, 1 out]
            n591 = global read "Global 1.vi" "Data Buffer 2"() -> (w1573:string[])
            n592 = Replace Array Subset(array=w1573, new element=w1569, index=w1566) -> (w1568:string[])
            n593 = Index Array(array=w1568, index=w1566) -> (element=w1567:string)
            n594 = global write "Global 1.vi" "Data Buffer 2"(w1568) -> ()
          }
        }
        n595 = Bundle By Name(cluster=w1542, "Kiértékelés"=TRUE, "Command.Eredmény"=w1534) -> (w1545:T3)
        n596 = Bundle By Name(cluster=w1541, "Data"=w1545) -> (w1544:T7)
        n597 = Unbundle By Name(w1544) -> ("Callback"=w1539:string)
        n598 = call-poly "Enqueue Message.vi"("error in (no error)"=w1536, "Message Data"=w1544, "Message"=w1539, "Message Queue"=w1537) -> ("error out"=w1543:errorcluster)  [unwired: 6 in, 1 out]
      }
      frame "ENGINE Compare Data" {
        w1596 = T3 {"Thread ID"=0.0, "Mérésszám"="", "Mérés/Utasítás"="", "Command"={"Parancs"="", "Paraméter 1"="", "Paraméter 2"="", "Paraméter 3"="", "Paraméter 4"="", "Paraméter 5"="", "Eredmény"=""}, "Min"="", "Max"="", "Aktív?"=FALSE, "Log?"=FALSE, "Kiértékelés"=FALSE, "Etalon 1 exp"=FALSE, "Etalon 2 exp"=FALSE, "Etalon 3 exp"=FALSE, "Etalon 4 exp"=FALSE, "Etalon 5 exp"=FALSE}  # Teszt cluster
        w1598 = T7 {"Thread ID"=0, "Callback"="", "Data"=variant, "Error"={"status"=FALSE, "code"=0, "source"=""}}  # Message
        n599 = Variant To Data(error in=w1593, type=w1598, Variant=w1594) -> (data=w1585:T7, error out=w1595:errorcluster)
        n600 = Unbundle By Name(w1585) -> ("Thread ID"=w1590:u16)
        n601 = Unbundle By Name(w1585) -> ("Data"=w1597:variant)
        n602 = Variant To Data(error in=w1595, type=w1596, Variant=w1597) -> (data=w1578:T3, error out=w1589:errorcluster)
        n603 = Unbundle By Name(w1578) -> ("Command.Paraméter 2"=w1592:string)
        n604 = Unbundle By Name(w1578) -> ("Command.Paraméter 1"=w1579:string)
        n605 = Unbundle By Name(w1578) -> ("Max"=w1577:string, "Min"=w1576:string)
        n606 = case shown="0, Default" w1590 {
          tunnel: w1592 -> [w1617 w1623]
          tunnel: w1589 -> [w1616 w1635]
          tunnel: [w1616 w1635] -> w1581
          tunnel: w1583 -> [w1615 w1634]
          tunnel: [w1615 w1634] -> w1582
          tunnel: [w1600 w1619] -> w1580
          tunnel: w1579 -> [w1613 w1622]
          tunnel: w1577 -> [w1606 w1621]
          tunnel: w1576 -> [w1604 w1620]
          tunnel: [w1602 w1618] -> w1575
          frame 0, Default {
            n607 = global read "Global 1.vi" "Data Buffer 1"() -> (w1611:string[])
            n608 = Decimal String To Number(string=w1617) -> (number=w1614:i32)  [unwired: 2 in, 1 out]
            n609 = Decimal String To Number(string=w1613) -> (number=w1612:i32)  [unwired: 2 in, 1 out]
            n610 = Fract/Exp String To Number(string=w1606) -> (number=w1605:dbl)  [unwired: 3 in, 1 out]
            n611 = Fract/Exp String To Number(string=w1604) -> (number=w1603:dbl)  [unwired: 3 in, 1 out]
            n612 = Index Array(array=w1611, index=w1614) -> (element=w1610:string)
            n613 = Index Array(array=w1611, index=w1612) -> (element=w1609:string)
            n614 = Fract/Exp String To Number(string=w1609) -> (number=w1607:dbl)  [unwired: 3 in, 1 out]
            n615 = Fract/Exp String To Number(string=w1610) -> (number=w1608:dbl)  [unwired: 3 in, 1 out]
            n616 = Subtract(x=w1608, y=w1607) -> (x-y=w1601:dbl)
            n617 = Number To Fractional String(number=w1601) -> (F-format string=w1600:string)  [unwired: 3 in]
            n618 = In Range and Coerce(upper limit=w1605, x=w1601, lower limit=w1603) -> (In Range?=w1602:bool)  [unwired: 1 out]
          }
          frame 1 {
            n619 = global read "Global 1.vi" "Data Buffer 2"() -> (w1631:string[])
            n620 = Decimal String To Number(string=w1623) -> (number=w1633:i32)  [unwired: 2 in, 1 out]
            n621 = Decimal String To Number(string=w1622) -> (number=w1632:i32)  [unwired: 2 in, 1 out]
            n622 = Fract/Exp String To Number(string=w1621) -> (number=w1626:dbl)  [unwired: 3 in, 1 out]
            n623 = Fract/Exp String To Number(string=w1620) -> (number=w1625:dbl)  [unwired: 3 in, 1 out]
            n624 = Index Array(array=w1631, index=w1633) -> (element=w1630:string)
            n625 = Index Array(array=w1631, index=w1632) -> (element=w1629:string)
            n626 = Fract/Exp String To Number(string=w1629) -> (number=w1627:dbl)  [unwired: 3 in, 1 out]
            n627 = Fract/Exp String To Number(string=w1630) -> (number=w1628:dbl)  [unwired: 3 in, 1 out]
            n628 = Subtract(x=w1628, y=w1627) -> (x-y=w1624:dbl)
            n629 = Number To Fractional String(number=w1624) -> (F-format string=w1619:string)  [unwired: 3 in]
            n630 = In Range and Coerce(upper limit=w1626, x=w1624, lower limit=w1625) -> (In Range?=w1618:bool)  [unwired: 1 out]
          }
        }
        n631 = Bundle By Name(cluster=w1578, "Kiértékelés"=w1575, "Command.Eredmény"=w1580) -> (w1588:T3)
        n632 = Bundle By Name(cluster=w1585, "Data"=w1588) -> (w1587:T7)
        n633 = Unbundle By Name(w1587) -> ("Callback"=w1584:string)
        n634 = call-poly "Enqueue Message.vi"("error in (no error)"=w1581, "Message Data"=w1587, "Message"=w1584, "Message Queue"=w1582) -> ("error out"=w1586:errorcluster)  [unwired: 6 in, 1 out]
      }
      frame "ENGINE Operator" {
        w1651 = T3 {"Thread ID"=0.0, "Mérésszám"="", "Mérés/Utasítás"="", "Command"={"Parancs"="", "Paraméter 1"="", "Paraméter 2"="", "Paraméter 3"="", "Paraméter 4"="", "Paraméter 5"="", "Eredmény"=""}, "Min"="", "Max"="", "Aktív?"=FALSE, "Log?"=FALSE, "Kiértékelés"=FALSE, "Etalon 1 exp"=FALSE, "Etalon 2 exp"=FALSE, "Etalon 3 exp"=FALSE, "Etalon 4 exp"=FALSE, "Etalon 5 exp"=FALSE}  # Teszt cluster
        w1653 = T7 {"Thread ID"=0, "Callback"="", "Data"=variant, "Error"={"status"=FALSE, "code"=0, "source"=""}}  # Message
        n635 = Variant To Data(error in=w1648, type=w1653, Variant=w1649) -> (data=w1642:T7, error out=w1650:errorcluster)
        n636 = Unbundle By Name(w1642) -> ("Data"=w1652:variant)
        n637 = Variant To Data(error in=w1650, type=w1651, Variant=w1652) -> (data=w1643:T3, error out=w1638:errorcluster)
        n638 = global read "Global 1.vi" "Operator"() -> (w1636:string)
        n639 = Bundle By Name(cluster=w1643, "Kiértékelés"=TRUE, "Command.Eredmény"=w1636) -> (w1646:T3)
        n640 = Bundle By Name(cluster=w1642, "Data"=w1646) -> (w1645:T7)
        n641 = Unbundle By Name(w1645) -> ("Callback"=w1641:string)
        n642 = call-poly "Enqueue Message.vi"("error in (no error)"=w1638, "Message Data"=w1645, "Message"=w1641, "Message Queue"=w1639) -> ("error out"=w1644:errorcluster)  [unwired: 6 in, 1 out]
      }
      frame "ENGINE Termék" {
        w1674 = T3 {"Thread ID"=0.0, "Mérésszám"="", "Mérés/Utasítás"="", "Command"={"Parancs"="", "Paraméter 1"="", "Paraméter 2"="", "Paraméter 3"="", "Paraméter 4"="", "Paraméter 5"="", "Eredmény"=""}, "Min"="", "Max"="", "Aktív?"=FALSE, "Log?"=FALSE, "Kiértékelés"=FALSE, "Etalon 1 exp"=FALSE, "Etalon 2 exp"=FALSE, "Etalon 3 exp"=FALSE, "Etalon 4 exp"=FALSE, "Etalon 5 exp"=FALSE}  # Teszt cluster
        w1676 = T7 {"Thread ID"=0, "Callback"="", "Data"=variant, "Error"={"status"=FALSE, "code"=0, "source"=""}}  # Message
        n643 = Variant To Data(error in=w1671, type=w1676, Variant=w1672) -> (data=w1662:T7, error out=w1673:errorcluster)
        n644 = Unbundle By Name(w1662) -> ("Data"=w1675:variant)
        n645 = Unbundle By Name(w1662) -> ("Thread ID"=w1659:u16)
        n646 = Variant To Data(error in=w1673, type=w1674, Variant=w1675) -> (data=w1667:T3, error out=w1664:errorcluster)
        n647 = Index Array(array=w1660, index=w1659) -> (element=w1661:T2)
        n648 = Unbundle By Name(w1661) -> ("Etalon number"=w1658:u32)
        n649 = Unbundle By Name(w1656) -> ("Termék név"=w1655:string)
        n650 = case shown="0, Default" w1658 {
          tunnel: [w1678 "Etalon1" ("Command.Eredmény") "Etalon2" ("Command.Eredmény") "Etalon3" ("Command.Eredmény") "Etalon4" ("Command.Eredmény") "Etalon5" ("Command.Eredmény")] -> w1657
          tunnel: w1655 -> [w1678 _ _ _ _ _]
          frame 0, Default {
          }
          frame 1 {
          }
          frame 2 {
          }
          frame 3 {
          }
          frame 4 {
          }
          frame 5 {
          }
        }
        n651 = Bundle By Name(cluster=w1667, "Kiértékelés"=TRUE, "Command.Eredmény"=w1657) -> (w1670:T3)
        n652 = Bundle By Name(cluster=w1662, "Data"=w1670) -> (w1669:T7)
        n653 = Unbundle By Name(w1669) -> ("Callback"=w1666:string)
        n654 = call-poly "Enqueue Message.vi"("error in (no error)"=w1664, "Message Data"=w1669, "Message"=w1666, "Message Queue"=w1665) -> ("error out"=w1668:errorcluster)  [unwired: 6 in, 1 out]
      }
      frame "ENGINE Set Statusbar" {
        w1704 = T3 {"Thread ID"=0.0, "Mérésszám"="", "Mérés/Utasítás"="", "Command"={"Parancs"="", "Paraméter 1"="", "Paraméter 2"="", "Paraméter 3"="", "Paraméter 4"="", "Paraméter 5"="", "Eredmény"=""}, "Min"="", "Max"="", "Aktív?"=FALSE, "Log?"=FALSE, "Kiértékelés"=FALSE, "Etalon 1 exp"=FALSE, "Etalon 2 exp"=FALSE, "Etalon 3 exp"=FALSE, "Etalon 4 exp"=FALSE, "Etalon 5 exp"=FALSE}  # Teszt cluster
        w1706 = T7 {"Thread ID"=0, "Callback"="", "Data"=variant, "Error"={"status"=FALSE, "code"=0, "source"=""}}  # Message
        n655 = Variant To Data(error in=w1701, type=w1706, Variant=w1702) -> (data=w1685:T7, error out=w1703:errorcluster)
        n656 = Unbundle By Name(w1685) -> ("Thread ID"=w1684:u16)
        n657 = Unbundle By Name(w1685) -> ("Data"=w1705:variant)
        n658 = Variant To Data(error in=w1703, type=w1704, Variant=w1705) -> (data=w1692:T3, error out=w1689:errorcluster)
        n659 = Unbundle By Name(w1692) -> ("Command.Paraméter 1"=w1688:string)
        n660 = Unbundle By Name(w1691) -> ("UI"=w1690:refnum<queue>)
        n661 = case shown="1" w1684 {
          tunnel: w1690 -> [w1712 w1717 _]
          tunnel: w1689 -> [w1711 w1716 w1718]
          tunnel: w1688 -> [w1710 w1715 _]
          tunnel: [w1708 w1713 w1718] -> w1686
          frame 0 {
            n662 = call-poly "Enqueue Message.vi"("error in (no error)"=w1711, "Message Data"=w1710, "Message"="Set Statusbar Main", "Message Queue"=w1712) -> ("error out"=w1708:errorcluster)  [unwired: 6 in, 1 out]
          }
          frame 1 {
            n663 = call-poly "Enqueue Message.vi"("error in (no error)"=w1716, "Message Data"=w1715, "Message"="Set Statusbar Main", "Message Queue"=w1717) -> ("error out"=w1713:errorcluster)  [unwired: 6 in, 1 out]
          }
          frame Default {
          }
        }
        n664 = Bundle By Name(cluster=w1692, "Kiértékelés"=TRUE, "Command.Eredmény"="") -> (w1699:T3)
        n665 = Bundle By Name(cluster=w1685, "Data"=w1699) -> (w1698:T7)
        n666 = Unbundle By Name(w1698) -> ("Callback"=w1696:string)
        n667 = call-poly "Enqueue Message.vi"("error in (no error)"=w1686, "Message Data"=w1698, "Message"=w1696, "Message Queue"=w1694) -> ("error out"=w1697:errorcluster)  [unwired: 6 in, 1 out]
      }
      frame "ENGINE Set Ellenállás" {
        w1739 = T3 {"Thread ID"=0.0, "Mérésszám"="", "Mérés/Utasítás"="", "Command"={"Parancs"="", "Paraméter 1"="", "Paraméter 2"="", "Paraméter 3"="", "Paraméter 4"="", "Paraméter 5"="", "Eredmény"=""}, "Min"="", "Max"="", "Aktív?"=FALSE, "Log?"=FALSE, "Kiértékelés"=FALSE, "Etalon 1 exp"=FALSE, "Etalon 2 exp"=FALSE, "Etalon 3 exp"=FALSE, "Etalon 4 exp"=FALSE, "Etalon 5 exp"=FALSE}  # Teszt cluster
        w1741 = T7 {"Thread ID"=0, "Callback"="", "Data"=variant, "Error"={"status"=FALSE, "code"=0, "source"=""}}  # Message
        n668 = Variant To Data(error in=w1736, type=w1741, Variant=w1737) -> (data=w1723:T7, error out=w1738:errorcluster)
        n669 = Unbundle By Name(w1723) -> ("Thread ID"=w1721:u16)
        n670 = Unbundle By Name(w1723) -> ("Data"=w1740:variant)
        n671 = Variant To Data(error in=w1738, type=w1739, Variant=w1740) -> (data=w1728:T3, error out=w1725:errorcluster)
        n672 = Index Array(array=w1722, index=w1721) -> (element=w1720:T2)
        n673 = Unbundle By Name(w1720) -> ("Previous Test.Kiértékelés"=w1719:bool)
        n674 = Unbundle By Name(w1727) -> ("UI"=w1726:refnum<queue>)
        n675 = case shown="1" w1721 {
          tunnel: w1726 -> [w1750 w1758 _]
          tunnel: w1725 -> [w1749 w1757 w1759]
          tunnel: [w1747 w1755 w1759] -> w1724
          tunnel: w1719 -> [w1746 w1754 _]
          frame 0 {
            n676 = Select(t=1, s=w1746, f=2) -> (s? t:f=w1743:i32)
            n677 = call-poly "Enqueue Message.vi"("error in (no error)"=w1749, "Message Data"=w1743, "Message"="Set Ellenállás", "Message Queue"=w1750) -> ("error out"=w1747:errorcluster)  [unwired: 6 in, 1 out]
          }
          frame 1 {
            n678 = Select(t=1, s=w1754, f=2) -> (s? t:f=w1751:i32)
            n679 = call-poly "Enqueue Message.vi"("error in (no error)"=w1757, "Message Data"=w1751, "Message"="Set Ellenállás", "Message Queue"=w1758) -> ("error out"=w1755:errorcluster)  [unwired: 6 in, 1 out]
          }
          frame Default {
          }
        }
        n680 = Bundle By Name(cluster=w1728, "Kiértékelés"=TRUE) -> (w1735:T3)
        n681 = Bundle By Name(cluster=w1723, "Data"=w1735) -> (w1734:T7)
        n682 = Unbundle By Name(w1734) -> ("Callback"=w1732:string)
        n683 = call-poly "Enqueue Message.vi"("error in (no error)"=w1724, "Message Data"=w1734, "Message"=w1732, "Message Queue"=w1730) -> ("error out"=w1733:errorcluster)  [unwired: 6 in, 1 out]
      }
      frame "ENGINE Clear Ellenállás" {
        w1778 = T3 {"Thread ID"=0.0, "Mérésszám"="", "Mérés/Utasítás"="", "Command"={"Parancs"="", "Paraméter 1"="", "Paraméter 2"="", "Paraméter 3"="", "Paraméter 4"="", "Paraméter 5"="", "Eredmény"=""}, "Min"="", "Max"="", "Aktív?"=FALSE, "Log?"=FALSE, "Kiértékelés"=FALSE, "Etalon 1 exp"=FALSE, "Etalon 2 exp"=FALSE, "Etalon 3 exp"=FALSE, "Etalon 4 exp"=FALSE, "Etalon 5 exp"=FALSE}  # Teszt cluster
        w1780 = T7 {"Thread ID"=0, "Callback"="", "Data"=variant, "Error"={"status"=FALSE, "code"=0, "source"=""}}  # Message
        n684 = Variant To Data(error in=w1775, type=w1780, Variant=w1776) -> (data=w1762:T7, error out=w1777:errorcluster)
        n685 = Unbundle By Name(w1762) -> ("Thread ID"=w1760:u16)
        n686 = Unbundle By Name(w1762) -> ("Data"=w1779:variant)
        n687 = Variant To Data(error in=w1777, type=w1778, Variant=w1779) -> (data=w1767:T3, error out=w1764:errorcluster)
        n688 = Unbundle By Name(w1766) -> ("UI"=w1765:refnum<queue>)
        n689 = case shown="0" w1760 {
          tunnel: w1765 -> [w1786 w1791 _]
          tunnel: w1764 -> [w1785 w1790 w1792]
          tunnel: [w1783 w1788 w1792] -> w1763
          frame 0 {
            n690 = call-poly "Enqueue Message.vi"("error in (no error)"=w1785, "Message Data"=0, "Message"="Set Ellenállás", "Message Queue"=w1786) -> ("error out"=w1783:errorcluster)  [unwired: 6 in, 1 out]
          }
          frame 1 {
            n691 = call-poly "Enqueue Message.vi"("error in (no error)"=w1790, "Message Data"=0, "Message"="Set Ellenállás", "Message Queue"=w1791) -> ("error out"=w1788:errorcluster)  [unwired: 6 in, 1 out]
          }
          frame Default {
          }
        }
        n692 = Bundle By Name(cluster=w1767, "Kiértékelés"=TRUE) -> (w1774:T3)
        n693 = Bundle By Name(cluster=w1762, "Data"=w1774) -> (w1773:T7)
        n694 = Unbundle By Name(w1773) -> ("Callback"=w1771:string)
        n695 = call-poly "Enqueue Message.vi"("error in (no error)"=w1763, "Message Data"=w1773, "Message"=w1771, "Message Queue"=w1769) -> ("error out"=w1772:errorcluster)  [unwired: 6 in, 1 out]
      }
      frame "ENGINE Date and Time" {
        w1813 = T3 {"Thread ID"=0.0, "Mérésszám"="", "Mérés/Utasítás"="", "Command"={"Parancs"="", "Paraméter 1"="", "Paraméter 2"="", "Paraméter 3"="", "Paraméter 4"="", "Paraméter 5"="", "Eredmény"=""}, "Min"="", "Max"="", "Aktív?"=FALSE, "Log?"=FALSE, "Kiértékelés"=FALSE, "Etalon 1 exp"=FALSE, "Etalon 2 exp"=FALSE, "Etalon 3 exp"=FALSE, "Etalon 4 exp"=FALSE, "Etalon 5 exp"=FALSE}  # Teszt cluster
        w1815 = T7 {"Thread ID"=0, "Callback"="", "Data"=variant, "Error"={"status"=FALSE, "code"=0, "source"=""}}  # Message
        n696 = Variant To Data(error in=w1810, type=w1815, Variant=w1811) -> (data=w1804:T7, error out=w1812:errorcluster)
        n697 = Unbundle By Name(w1804) -> ("Data"=w1814:variant)
        n698 = Variant To Data(error in=w1812, type=w1813, Variant=w1814) -> (data=w1805:T3, error out=w1800:errorcluster)
        n699 = Get Date/Time In Seconds() -> (seconds since 1Jan1904=w1796:timestamp)
        n700 = Format Date/Time String(seconds (now)=w1796) -> (date/time string=w1797:string)  [unwired: 2 in]
        n701 = Format Date/Time String(time format string (%c)="%Y%m%d_%H%M%S", seconds (now)=w1796) -> (date/time string=w1795:string)  [unwired: 1 in]
        n702 = Format Date/Time String(time format string (%c)="%d.%m.%y") -> (date/time string=w1793:string)  [unwired: 2 in]
        n703 = global write "Global 1.vi" "Date and Time to Print"(w1793) -> ()
        n704 = global write "Global 1.vi" "Date and Time"(w1795) -> ()
        n705 = Bundle By Name(cluster=w1805, "Kiértékelés"=TRUE, "Command.Eredmény"=w1797) -> (w1808:T3)
        n706 = Bundle By Name(cluster=w1804, "Data"=w1808) -> (w1807:T7)
        n707 = Unbundle By Name(w1807) -> ("Callback"=w1803:string)
        n708 = call-poly "Enqueue Message.vi"("error in (no error)"=w1800, "Message Data"=w1807, "Message"=w1803, "Message Queue"=w1801) -> ("error out"=w1806:errorcluster)  [unwired: 6 in, 1 out]
      }
      frame "ENGINE Dialog Window" {
        w1831 = T3 {"Thread ID"=0.0, "Mérésszám"="", "Mérés/Utasítás"="", "Command"={"Parancs"="", "Paraméter 1"="", "Paraméter 2"="", "Paraméter 3"="", "Paraméter 4"="", "Paraméter 5"="", "Eredmény"=""}, "Min"="", "Max"="", "Aktív?"=FALSE, "Log?"=FALSE, "Kiértékelés"=FALSE, "Etalon 1 exp"=FALSE, "Etalon 2 exp"=FALSE, "Etalon 3 exp"=FALSE, "Etalon 4 exp"=FALSE, "Etalon 5 exp"=FALSE}  # Teszt cluster
        w1833 = T7 {"Thread ID"=0, "Callback"="", "Data"=variant, "Error"={"status"=FALSE, "code"=0, "source"=""}}  # Message
        n709 = Variant To Data(error in=w1828, type=w1833, Variant=w1829) -> (data=w1822:T7, error out=w1830:errorcluster)
        n710 = Unbundle By Name(w1822) -> ("Thread ID"=w1817:u16)
        n711 = Unbundle By Name(w1822) -> ("Data"=w1832:variant)
        n712 = Variant To Data(error in=w1830, type=w1831, Variant=w1832) -> (data=w1825:T3, error out=w1827:errorcluster)
        n713 = Unbundle By Name(w1825) -> ("Command.Paraméter 1"=w1824:string, "Command.Paraméter 2"=w1821:string)
        n714 = case shown="0, Default" w1817 {
          tunnel: w1827 -> [w1842 w1855]
          tunnel: w1826 -> [w1843 w1856]
          tunnel: w1824 -> [w1834 w1847]
          tunnel: [w1840 w1853] -> w1823
          tunnel: w1822 -> [w1838 w1851]
          tunnel: w1821 -> [w1837 w1850]
          frame 0, Default {
            n715 = call <vilib>:"Application Directory.vi"() -> ("Application Directory"=w1836:path)
            n716 = Build Path(base path=w1836, name or relative path=w1834) -> (appended path=w1835:path)
            n717 = Open VI Reference(type specifier VI Refnum (for type only)=refnum<vi> refnum, vi path=w1835, options=192, error in (no error)=w1842) -> (vi reference=w1844:refnum<vi>, error out=w1841:errorcluster)  [unwired: 2 in]
            n718 = call-by-ref "Start Asynchronous Call"(reference=w1844, error in=w1841, "Front Panel Window:Panel Bounds"=T6 {"Left"=260, "Top"=260, "Right"=0, "Bottom"=0}, "Üzenet be"=w1837, "Error In"=w1841, "Message"=w1838, "Message Queue"=w1843) -> (error out=w1840:errorcluster)  [unwired: 6 in, 2 out]
          }
          frame 1 {
            n719 = call <vilib>:"Application Directory.vi"() -> ("Application Directory"=w1849:path)
            n720 = Build Path(base path=w1849, name or relative path=w1847) -> (appended path=w1848:path)
            n721 = Open VI Reference(type specifier VI Refnum (for type only)=refnum<vi> refnum, vi path=w1848, options=192, error in (no error)=w1855) -> (vi reference=w1857:refnum<vi>, error out=w1854:errorcluster)  [unwired: 2 in]
            n722 = call-by-ref "Start Asynchronous Call"(reference=w1857, error in=w1854, "Front Panel Window:Panel Bounds"=T6 {"Left"=1000, "Top"=260, "Right"=0, "Bottom"=0}, "Üzenet be"=w1850, "Error In"=w1854, "Message"=w1851, "Message Queue"=w1856) -> (error out=w1853:errorcluster)  [unwired: 6 in, 2 out]
          }
        }
      }
      frame "Error" {
        n723 = Unbundle By Name(w1870) -> ("UI"=w1869:refnum<queue>)
        n724 = call-poly "Enqueue Message.vi"("error in (no error)"=w1860, "Message Data"=w1868, "Message"="Error", "Message Queue"=w1869) -> ("error out"=w1861:errorcluster)  [unwired: 6 in, 1 out]
        n725 = call-poly "Enqueue Message.vi"("Priority Message? (F)"=TRUE, "error in (no error)"=w1860, "Message"="Initiate Stop", "Message Queue"=w1862) -> ("error out"=w1863:errorcluster)  [unwired: 6 in, 1 out]
        n726 = Merge Errors(w1861, w1863) -> (w1864:errorcluster)
      }
      frame "Initiate Stop" {
        n727 = call-poly "Enqueue Message.vi"("Priority Message? (F)"=TRUE, "error in (no error)"=w1878, "Message"="Program Stop", "Message Queue"=w1877) -> ("error out"=w1879:errorcluster)  [unwired: 6 in, 1 out]
      }
      frame "Program Stop" {
        # "Program Stop"
        n728 = Flush Queue(queue=w1887, error in (no error)=w1888) -> (error out=w1883:errorcluster)  [unwired: 2 out]
      }
      frame Default {
        # "Nem létezõ parancs esetén fut csak le, hibát generál"
        n729 = xnode "Error Ring"("parameter 0"=w1892) -> ("error out"=w1893:errorcluster)
      }
    }
    "Threads" <- w16
    n730 = call "Error Handler - Message Handling Loop.vi"("error in (no error)"=w10, "Message Queue"=w8) -> ("dup error in"=w9:errorcluster)  [unwired: 8 in, 1 out]
  }
  "Error Out" <- w5
